vi "ControlProgram5.7.vi"() -> ()   [LabVIEW 2016]
uses:
  <vilib>/Utility/miscctls.llb/LVPoint32TypeDef.ctl
  <vilib>/Platform/TimedLoop/XDataNode/timing_clust.ctl
  <vilib>/Platform/TimedLoop/XDataNode/nitl_modes.ctl
  <vilib>/Platform/TimedLoop/XDataNode/wakeup.ctl
  <vilib>/vision/Avi1.llb/AviRefnum.ctl
  <vilib>/Utility/error.llb/DialogType.ctl
  <vilib>/DAQmx/write.llb/DAQmx Write (Analog 1D DBL NChan 1Samp).vi
  <vilib>/DAQmx/read.llb/DAQmx Read (Analog 2D DBL NChan NSamp).vi
  <vilib>/Analysis/baseanly.llb/Mean (DBL).vi
  <vilib>/DAQmx/write.llb/DAQmx Write (Digital Bool 1Line 1Point).vi
  <vilib>/DAQmx/create/channels.llb/DAQmx Create Channel (DO-Digital Output).vi
  <vilib>/Instr/_visa.llb/VISA Configure Serial Port (Instr).vi
  <vilib>/DAQmx/create/channels.llb/DAQmx Create Channel (AI-Voltage-Basic).vi
  <vilib>/DAQmx/create/channels.llb/DAQmx Create Channel (AO-Voltage-Basic).vi
  <vilib>/DAQmx/configure/timing.llb/DAQmx Timing (Sample Clock).vi
  <vilib>/DAQmx/miscellaneous.llb/DAQmx Fill In Error Info.vi
  <vilib>/Utility/inputDevices.llb/mouseAcquire.vi
  <vilib>/Utility/inputDevices.llb/closeMouse.vi
  <vilib>/platform/TimedLoop/XDataNode/XDataNode.xnode
  <vilib>/Platform/TimedLoop/XDataNode/XDNodeRunTimeDep.lvlib
  <resource>/objmgr/daqmx.rc
  <vilib>/Analysis/NI_AALBase.lvlib
panel:
  out "Primary Video Display":T1(plugin-control)
  in  "Save file index":i32
  out "Flush Sample Start Time":u32=2111292881
  out "Sample flush time (s)":dbl=48.0
  in  "Inject Sample":bool
  out "Chart Freq (Hz)":dbl=500.0
  out "Cal values":T2={"AX alpha"=612.9626061060078, "BX alpha"=549.6584469744151, "AX kappa"=0.3485731373010688, "BX kappa"=0.3853424216291352, "AX offset"=-0.03900484438240665, "BX offset"=-0.11295550662085417, "AY alpha"=582.7562541114835, "BY alpha"=571.1587543790358, "AY kappa"=0.37498408087930674, "BY kappa"=0.36252029651198364, "AY offset"=-0.21125584642206058, "BY offset"=-0.12469077200400738}
  in  "Inject Pump 1":bool
  in  "Inject Pump 2":bool
  in  "Tab Control 2":T3(tab)
  in  "Force FB script":bool
  in  "Got ADig bead":bool
  in  "Move Cap. 2 (ADig Top)":bool
  in  "Dump beads":bool
  in  "Got DNA bead":bool
  in  "Flow on\ncap 2?":bool=TRUE
  in  "Flow on\ncap 1?":bool=TRUE
  in  "Flow on\ndump?":bool=TRUE
  in  "Fish After TA?":bool=TRUE
  in  "Delta after tether":dbl=1700.0
  in  "TA Cancel Save?":bool=TRUE
  in  "Min fish\ndelta (nm)":dbl=1425.0 min=0.0 max=5000.0 step=50.0
  in  "Max fish\ndelta (nm)":dbl=1900.0 min=0.0 max=5000.0 step=25.0
  in  "Fish Speed (ms)":i32=5000
  in  "Wait (ms)":i32=1500
  in  "# attempts":dbl=10.0
  in  "Cutoff force (pN)":dbl=4.5
  in  "Raster after\n tether?":bool=TRUE
  out "Tether":bool
  out "Attempt #":i32
  in  "Flow on\nwhile fish?":bool=TRUE
  in  "Flow on\nafter raster?":bool=TRUE
  in  "Offset @ Delta (nm)":dbl=1700.0
  in  "Cal @ Delta (nm)":dbl=2500.0
  in  "Cal stage position":i32=3
  out "Cal Final Sampling Rate":dbl=125000.0
  in  "Cal Averaging":i32=1
  in  "Wait before dip (s)":dbl=3.0
  in  "Start dipping after?":bool
  in  "Start trap delta (nm)":dbl=1700.0
  in  "Cancel dwell":bool
  in  "Pause dwell":bool
  in  "Return position":dbl=3.0
  in  "Dip duration":dbl=15.0
  in  "Dip position":dbl=4.0
  in  "Dip":bool
  out "Dip time":i32
  in  "Stop":bool=TRUE
  in  "?":T4(tab)
  in  "Cal time (s)":dbl=5.0
  in  "Save N sets":bool
  in  "N sets":i32=200
  out "Cal sets to save":i32=500
  in  "Reset data stream":bool
  out "Buffer Overflow":bool
  out "Stage moving":bool
  in  "Comment":string
  in  "Raster scan":bool
  out "Saving":bool
  in  "Save cal":bool
  in  "Save Data":bool
  in  "Stop saving":bool
  out "Calibrating":bool
  out "Progress":dbl(slide) scale=0.0..100.0
  in  "Read Cal":bool
  in  "Fish":bool
  in  "Averaging Number":i32=1250
  out "Final Sampling Rate":dbl=100.0
  in  "Trap position (V)":cluster{"X":dbl, "Y":dbl}={"X"=3.9042624789680316, "Y"=0.2}
  in  "Trap delta (nm)":dbl=2500.0 min=0.0 max=5000.0 step=50.0
  in  "Fixed X":dbl=1.3
  in  "Fixed Y":dbl=1.8
  in  "Shutter 1 (B)":bool
  in  "Shutter 2 (A)":bool
  in  "Pulling direction":bool
  out "Raster scanning...":bool
  out "Current file name":path=path "D:/data/160111/160111_006.dat"
  in  "AX alpha":dbl=612.9626061060078 format="%#_3p"
  in  "BX alpha":dbl=549.6584469744151 format="%#_3g"
  in  "AX kappa":dbl=0.3485731373010688 format="%#_3g"
  in  "BX kappa":dbl=0.3853424216291352 format="%#_3g"
  in  "AX offset":dbl=-0.03900484438240665 format="%#_3g"
  in  "BX offset":dbl=-0.11295550662085417 format="%#_3g"
  in  "AY alpha":dbl=582.7562541114835 format="%#_3g"
  in  "BY alpha":dbl=571.1587543790358 format="%#_3g"
  in  "AY kappa":dbl=0.37498408087930674 format="%#_3g"
  in  "BY kappa":dbl=0.36252029651198364 format="%#_3g"
  in  "AY offset":dbl=-0.21125584642206058 format="%#_3g"
  in  "BY offset":dbl=-0.12469077200400738 format="%#_3g"
  out "Buffer status":u8(slide) scale=0.0..100.0
  in  "Target":bool
  in  "Set Current\nPos to (0,0,0)":bool
  in  "dump spot":string="Dump beads spot"
  in  "up flow spot":string="Upper flow spot"
  in  "low flow spot":string="Lower flow spot"
  in  "up cap":string="Upper capillary (ADig beads)"
  in  "bottom cap":string="Lower capillary (DNA beads)"
  in  "Move to Position 5":bool
  in  "Set Position 5":bool
  in  "Saved stage positions":dbl[][](array[numeric])=[[1.0, 0.0, 0.0, 0.0], [2.0, -0.13716, -3.21132, 0.01436], [3.0, 0.45, -0.73974, 0.005], [4.0, 0.45, -2.1978, 0.005], [5.0, 0.45, -2.63158, -0.02256]]
  in  "Set Position 2":bool
  in  "Move to Position 2":bool
  in  "Set Position 1":bool
  in  "Move to Position 1":bool
  in  "Set Position 4":bool
  in  "Move to Position 4":bool
  in  "Set Position 3":bool
  in  "Move to Position 3":bool
  out "Stage error":errorcluster
  in  "Clear Volume":bool
  out "Sample Flush Meter":u8(slide) scale=0.0..100.0
  out "Flushing Sample":bool
  in  "Flush Sample":bool
  in  "Normal \nRate (ul/hr)  3":dbl=100.0
  in  "Normal \nVolume (ul) 3":dbl=250.0
  in  "Normal \nVolume (ul) 2":dbl
  in  "Normal \nRate (ul/hr)":dbl
  in  "Normal \nVolume (ul)":dbl
  in  "Flush\nRate (ul/min)":dbl
  in  "Flush\nVolume (ul)":dbl
  in  "Flush \nRate (ul/min)  2":dbl
  in  "Flush Pump 2":bool
  in  "Flush\nVolume (ul)  2":dbl
  in  "Flush Pump 1":bool
  in  "Normal \nRate (ul/hr)  2":dbl
  in  "Write Wait":i32=1000
  in  "Flush \nRate (ul/min)  3":dbl=100.0
  in  "Flush\nVolume (ul)  3":dbl=80.0
  out "error out":errorcluster
  in  "Use Mouse to Move Trap?":bool
  in  "Pause Mouse/Mirror Connection":bool
  out "Reference Voltage":cluster{dbl, dbl}={0.0, -0.0}
  out "Saved voltage":cluster{dbl, dbl}={5.766666666666665, 1.45}
  out "Real Coordinates":cluster{"Horizontal":i32, "Vertical":i32}={"Horizontal"=897, "Vertical"=-1271}
  out "CoordinatesMousePressed":T5
  out "Sum error":dbl(knob) scale=-0.03..0.03
  out "Trap sep":waveform(dbl)[](graph)=[{"t0"=timestamp(16.979999999999855 s since 1904-01-01), "dt"=0.002, "Y"=[2501.0314192873643, 2501.00154430026, 2501.0038423761266, 2500.885491465706, 2500.985457768662], "attributes"=variant("NI_ChannelName"=variant(string "T2 X"))}, {"t0"=timestamp(16.979999999999855 s since 1904-01-01), "dt"=0.002, "Y"=[3.686857270925411, 3.6764288887082217, 3.712276452521894, 3.65426857654364, 3.634715359919401], "attributes"=variant("NI_ChannelName"=variant(string "T2 Y"))}]
  in  "Set reading to\nsetpoint":bool
  in  "Offset Y (nm)":dbl format="%0.2f"
  in  "Offset X (nm)":dbl format="%0.2f"
  in  "Remove offsets":bool
  in  "Force Feedback":bool
  out "Feedback Output Voltage 2":cluster{dbl, dbl} {"?" format="%#_4g"; "?" format="%#_4g"}
  in  "Offset":cluster{"Off Y":dbl, "Off X":dbl}={"Off Y"=1.5, "Off X"=0.17}
  in  "Setpoint voltage":cluster{"SP Y":dbl, "SP X":dbl}={"SP Y"=0.6, "SP X"=0.0}
  in  "Feedback const":T6={"Ki_B_Y"=0.5, "Ki_B_X"=0.0, "Kp Y"=1.0, "Kp X"=0.0}
  out "Mean Trap Pos X 2 (nm)":dbl=2500.981551039624 format="%0.2f"
  out "Mean Trp Pos Y 2 (nm)":dbl=3.6729093097237135 format="%0.2f"
  out "T2 X RMS (A)":dbl=0.5025172745235221 format="%0.2f"
  out "T2 Y RMS (A)":dbl=0.2669441786272784 format="%0.2f"
  in  "Scan range (nm)":dbl=425.0
  in  "Scan speed (nm/s)":dbl=100.0 min=0.0 max=100.0
  in  "Step size (nm)":dbl=1.0
  in  "Save scans":bool=TRUE
  in  "# scans":i32=1
  in  "Load param":bool
  in  "Scan Parameters":T7(array[cluster])=[{"Label"="Offset", "Max delta 2"=3.8, "Start delta 2"=2.4, "Speed (ms) 2"=10000, "# scans 2"=1}]
  in  "Trap delta\nafter (nm)":dbl=1750.0
  in  "Stop raster":bool
  out "Scan range (V)":dbl=0.47672462142456534
  out "Scan steps (mirror)":u64=425
  out "Scan increment (V)":dbl=0.0011217049915872126
  out "Time per step (ms)":dbl=10.0
  out "Total raster time (s)":dbl=8.5
  out "N sets to be saved":dbl=850.0
  in  "Zoom Factor":sgl=7.0
  in  "Center Point":cluster{"X":i32, "Y":i32}={"X"=335, "Y"=271}
  in  "Intensity Upper":dbl=88.0
  in  "Intensity Lower":dbl=66.0
  out "Window Size":cluster{"Height":i32, "Width":i32}
  in  "Image Index":dbl=1.0 min=1.0
  in  "Save Image":bool
  in  "Averaging":bool
  in  "Reset Averaging":bool
  in  "Save Video":bool
  in  "New Video File":bool
  in  "Video Index":dbl=1.0 min=1.0 step=1.0
  in  "Video Capture Rate (Hz)":dbl=30.0
  in  "Initial Window Size":cluster{"Width":i32, "Height":i32}={"Width"=884, "Height"=619}
  in  "Initial Window Position":cluster{"X Position":i32, "Y Position":i32}={"X Position"=796, "Y Position"=4}
  out "Window Position":cluster{"X Position":i32, "Y Position":i32}={"X Position"=40, "Y Position"=40}
  out "Path Out":path
  in  "Target coordinates":cluster{"X1":dbl, "Y1":dbl, "X2":dbl, "Y2":dbl}={"X1"=328.0, "Y1"=274.0, "X2"=368.0, "Y2"=314.0}
  in  "# Samples/channel (in)":i32=40000 format="%.2f"
  out "Buffer size\n(Samples/channel)":u32=511
  out "DAQ rate\n(Samples/s)":dbl=125000.0 format="%#_6p"
  out "# Samples/channel":i32=1250
  out "# Samples/channel/s":dbl=100.0
  out "AvailSampPerChan":u32=9
  out "Data update period (s/set)":dbl=0.01 format="%#_6p"
  out "AvailSampPerChan 2":u32=110
  in  "PC samp per channel":i32=1000
  in  "Sampling Rate":dbl=125000.0 format="%0.0p"
  in  "DAQ Rate2":dbl=1000000.0 format="%#_6p"
  out "Data period (s)":dbl=8e-06 format="%#_6p"
  in  "Tether break\nforce (pN)":dbl=1.0
  in  "Path":path=path "E:/Data"
  out "Mirror task":refnum<k21>
  in  "Conv X (nm/V)":dbl=891.5
  in  "Conv Y (nm/V)":dbl=505.7
  in  "Min value Y":dbl format="%.1g"
  in  "Max value Y":dbl=10.0 format="%.1f"
  in  "Min value X":dbl format="%0.1f"
  in  "Max value X":dbl=10.0 format="%.1f"
  in  "HWP1":string="Half waveplate 1: differential trap power"
  in  "HWP0":string="Half waveplate 0: total trap power"
  in  "Move 1":bool
  in  "\"Degrees\" 1":dbl
  in  "Move 0":bool
  in  "\"Degrees\" 0":dbl
  out "Deflection":T5
  in  "Sampling Rate":dbl=125000.0 format="%0.2f"
  in  "Averaging Number":i32=12500
  in  "DAQ Rate":dbl=1000000.0
  out "Final Sampling Rate":dbl
  in  "Tab Control":T8(tab)
  in  "Downsamp\nfact":dbl=250.0
  out "Bead sep":waveform(dbl)[](graph)=[{"t0"=timestamp(16.979999999999855 s since 1904-01-01), "dt"=0.002, "Y"=[1328.897036761212, 1305.1388835394264, 1332.9488147379952, 1348.9983032616292, 1330.6351248700973], "attributes"=variant("NI_ChannelName"=variant(string "T2"))}, {"t0"=timestamp(16.979999999999855 s since 1904-01-01), "dt"=0.002, "Y"=[125.02264592216193, 122.42682026580995, 123.20185663198687, 125.52620860986364, 123.54404369854063], "attributes"=variant("NI_ChannelName"=variant(string "T1"))}]
  out "Force (pN)":waveform(dbl)[](graph)=[{"t0"=timestamp(16.979999999999855 s since 1904-01-01), "dt"=0.002, "Y"=[464.2815568920448, 456.0098292427729, 465.67524311796336, 471.29790632841843, 464.8843576940994], "attributes"=variant("NI_ChannelName"=variant(string "T2"))}, {"t0"=timestamp(16.979999999999855 s since 1904-01-01), "dt"=0.002, "Y"=[45.46636056045166, 44.5015348242116, 44.800567281242486, 45.640259630893546, 44.914644785188166], "attributes"=variant("NI_ChannelName"=variant(string "T1"))}]
  out "Mean force (pN)":dbl=254.74722603572863 format="%0.2f"
  out "Force noise (pN)":dbl=2.6193969378282405 format="%0.2f"
  out "Mean Bead Sep\n(nm)":dbl=726.6339738298723 format="%0.2f"
  out "Bead Sep Noise\n(A)":dbl=74.90033509004418 format="%0.2f"
  out "PSD 2":cluster{dbl[], dbl[]}(graph)
  out "PSD 1":cluster{dbl[], dbl[]}(graph)
  out "PSD 1 Sum":dbl(slide) scale=0.0..10.0
  out "PSD 2 Sum":dbl(slide) scale=0.0..10.0
  in  "Start":bool
  out "All signals":waveform(dbl)[](graph)=[{"t0"=timestamp(16.979999999999855 s since 1904-01-01), "dt"=0.002, "Y"=[0.0016346282006063629, 0.0016395264340522623, 0.0015951845291293394, 0.001643393460571591, 0.001619417895638828], "attributes"=variant("NI_ChannelName"=variant(string "A y"))}, {"t0"=timestamp(16.979999999999855 s since 1904-01-01), "dt"=0.002, "Y"=[0.019187765824921398, 0.019071754997447867, 0.019093410352219186, 0.01908722310790174, 0.01906840357389384], "attributes"=variant("NI_ChannelName"=variant(string "A x"))}, {"t0"=timestamp(16.979999999999855 s since 1904-01-01), "dt"=0.002, "Y"=[-0.0018054787241975109, -0.0017869169958937155, -0.0017822765638718496, -0.001786143590850525, -0.0017809875549530127], "attributes"=variant("NI_ChannelName"=variant(string "B y"))}, {"t0"=timestamp(16.979999999999855 s since 1904-01-01), "dt"=0.002, "Y"=[-0.00033504945472925915, -0.00036108743413889715, -0.0003409788953336346, -0.00033788527392585174, -0.0003489707505394131], "attributes"=variant("NI_ChannelName"=variant(string "B x"))}, {"t0"=timestamp(16.979999999999855 s since 1904-01-01), "dt"=0.002, "Y"=[0.009149844795781155, 0.009267130525609176, 0.00907380239980559, 0.008962960940972408, 0.00908024667059773], "attributes"=variant("NI_ChannelName"=variant(string "A sum"))}, {"t0"=timestamp(16.979999999999855 s since 1904-01-01), "dt"=0.002, "Y"=[0.005338703023696027, 0.005341280732029953, 0.005316792503079397, 0.005262660628286258, 0.005297459690626533], "attributes"=variant("NI_ChannelName"=variant(string "B sum"))}, {"t0"=timestamp(16.979999999999855 s since 1904-01-01), "dt"=0.002, "Y"=[3.905419427131087, 3.9053859162089286, 3.9053884939720995, 3.9052557391651215, 3.905367871866138], "attributes"=variant("NI_ChannelName"=variant(string "Trap x"))}, {"t0"=timestamp(16.979999999999855 s since 1904-01-01), "dt"=0.002, "Y"=[0.2072906016826684, 0.2072699800053554, 0.20734086702100435, 0.2072261589411581, 0.20718749329626143], "attributes"=variant("NI_ChannelName"=variant(string "Trap y"))}]
  # "Bead Calibration"
  # "Y"
  # "X"
  # "Pump #1 Controls"
  # "Pump #2 Controls"
  # "Sample Pump Controls"
  # "Retract the pumps manually. Change it back to INFUSE when you're done. Suck it up, don't whine."
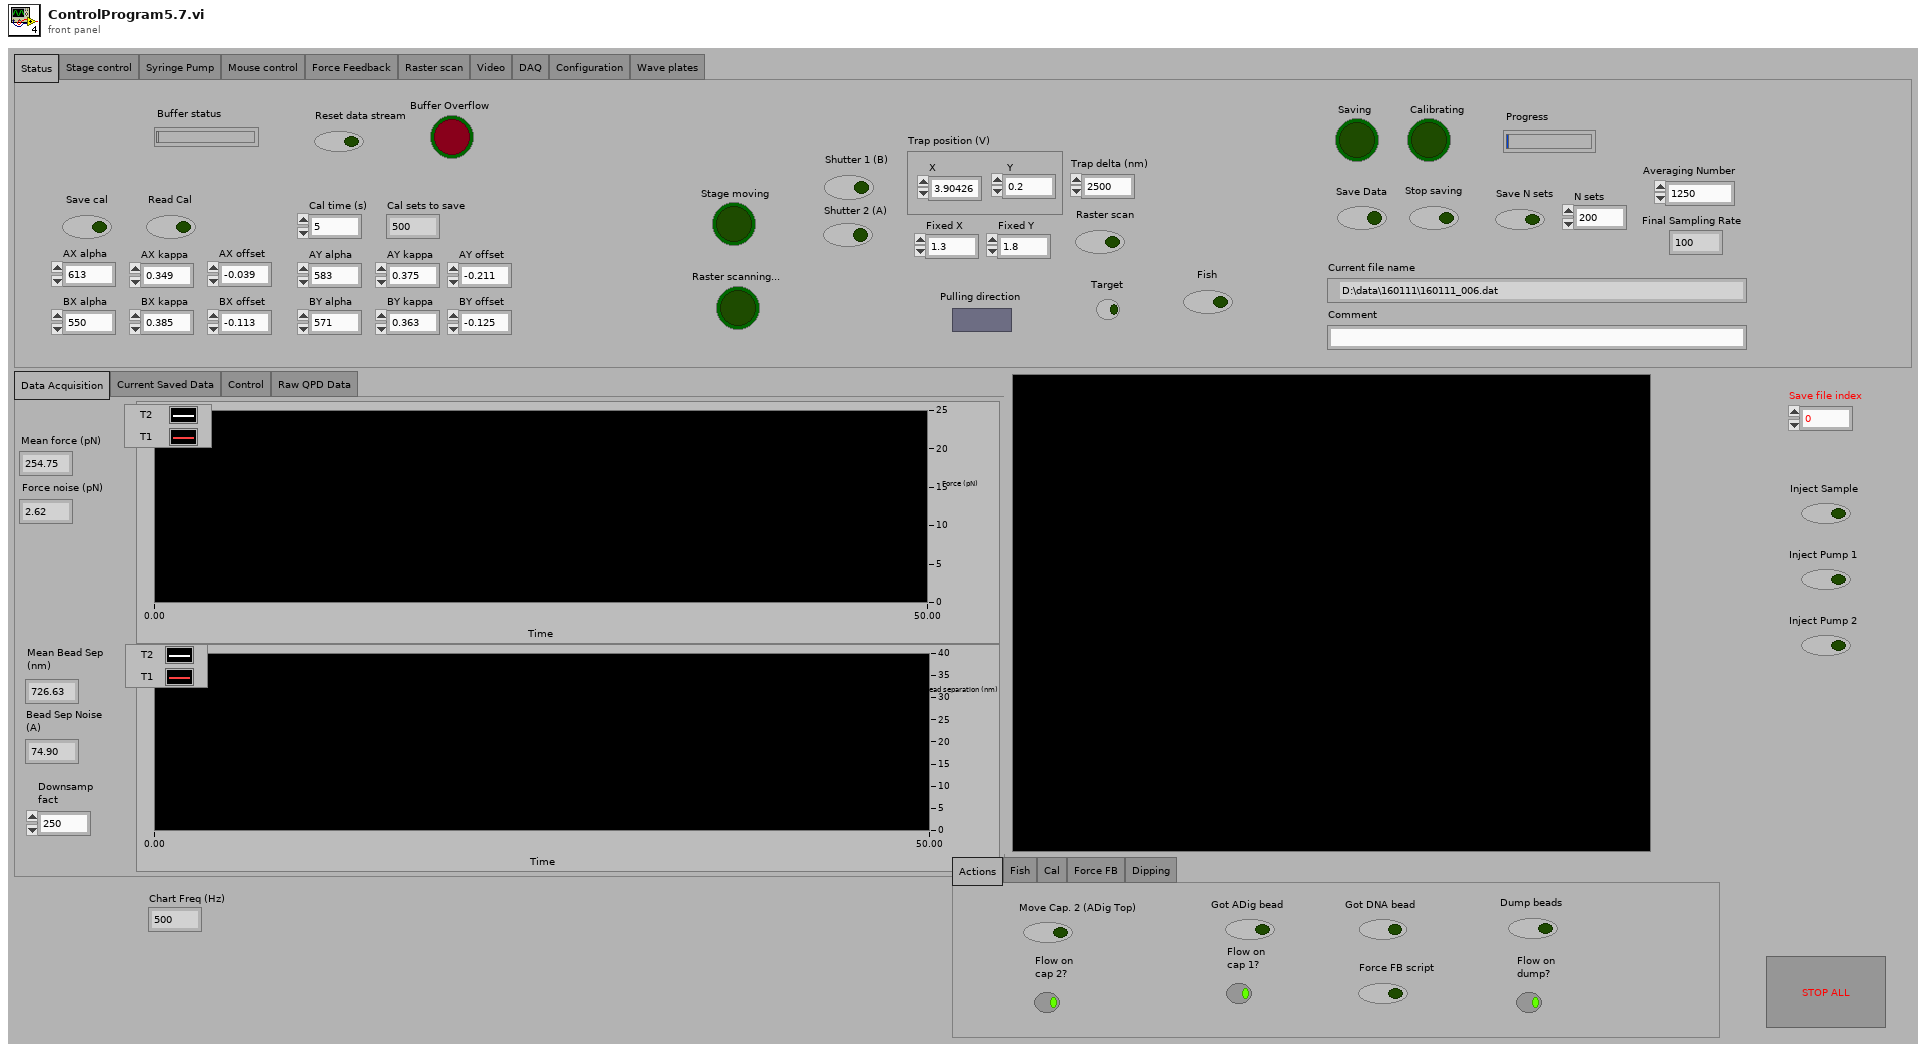
[diagram p1: front panel]
types:
  T1 = typedef "IMAQ Image.ctl" = refnum<image>
  T2 = cluster{"AX alpha":dbl, "BX alpha":dbl, "AX kappa":dbl, "BX kappa":dbl, "AX offset":dbl, "BX offset":dbl, "AY alpha":dbl, "BY alpha":dbl, "AY kappa":dbl, "BY kappa":dbl, "AY offset":dbl, "BY offset":dbl}
  T3 = enum32{"Actions", "Fish", "Cal", "Force FB", "Dipping"}
  T4 = enum32{"Status", "Stage control", "Syringe Pump", "Mouse control", "Force Feedback", "Raster scan", "Video", "DAQ", "Configuration", "Wave plates"}
  T5 = typedef "LVPoint32TypeDef.ctl" = cluster{"Horizontal":i32, "Vertical":i32}
  T6 = cluster{"Ki_B_Y":dbl, "Ki_B_X":dbl, "Kp Y":dbl, "Kp X":dbl}
  T7 = cluster{"Label":string, "Max delta 2":dbl, "Start delta 2":dbl, "Speed (ms) 2":i32, "# scans 2":i32}[]
  T8 = enum32{"Data Acquisition", "Current Saved Data", "Control", "Raw QPD Data"}
  T9 = enum32{"setting", "request", "request control", "info", "statistics", "system settings", "I/O sub system", "HRT control", "camera descriptions", "device specific data", "event sub system settings", "event sub system results", "image memory manager"}
  T10 = typedef "AviRefnum.ctl" = refnum<k1>
  T11 = typedef "XDNodeRunTimeDep.lvlib/timing_clust.ctl" = cluster{"Expected End [f-1]":u64, "Actual End [f-1]":u64, "Finished Late? [f-1]":bool, "Expected End [i-1]":u64, "Actual End [i-1]":u64, "Finished Late? [i-1]":bool, "Expected Start [i]":u64, "Actual Start [i]":u64, "Expected Start [f]":u64, "Actual Start [f]":u64, "Source Name":string, "Structure Name":string, "Period":i64, "Deadline":i64, "Offset":i64, "Start":i64, "Priority":i32, "Timeout":i32, "Mode":T12, "Wakeup Reason":T13, "Error":errorcluster, "Source Type":string, "Secondary Source Type":string, "Global End Time":u64, "Global Start Time":u64, "Frame Duration":u64, "Iteration Duration":u64, "Assigned CPU":i32, "I/O Scan Engine Mode":u32}
  T12 = typedef "XDNodeRunTimeDep.lvlib/nitl_modes.ctl" = enum32{"No Change", "Process missed periods, maintain original phase", "Discard missed periods, maintain original phase", "Process missed periods, ignore original phase", "Discard missed periods, ignore original phase"}
  T13 = typedef "XDNodeRunTimeDep.lvlib/wakeup.ctl" = enum32{"Normal", "Aborted", "Asynchronous wakeup", "Timing source error", "Timed loop error", "Timeout"}
  T14 = typedef "Image Type" = u32
  T15 = typedef "imagedata.ctl" = cluster{"image type":i32, "image depth":i32, "image":u8[], "mask":u8[], "colors":u32[], "Rectangle":cluster{"left":i16, "top":i16, "right":i16, "bottom":i16}}
  T16 = enum16{"open", "replace", "create", "open or create", "replace or create", "replace or create with confirmation"}
  T17 = enum16{"big-endian, network order", "native, host order", "little-endian"}
  T18 = cluster{string, string, string, string, string, string, string, string}
  T19 = typedef "DialogType.ctl" = u16
  T20 = cluster{"button 1":bool, "button 2":bool, "button 3":bool, "button 4":bool}
  T21 = cluster{"[0]":dbl, "[1]":dbl, "[2]":dbl, "[3]":dbl, "[4]":dbl, "[5]":dbl, "[6]":dbl, "[7]":dbl, "[8]":dbl, "[9]":dbl, "[10]":dbl, "[11]":dbl}
  T22 = cluster{"Label":string, "Max delta 2":dbl, "Start delta 2":dbl, "Speed (ms) 2":i32, "# scans 2":i32}
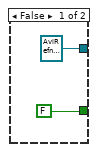
[diagram p2: hidden frame]
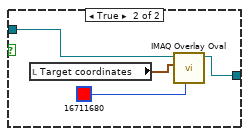
[diagram p5: hidden frame]
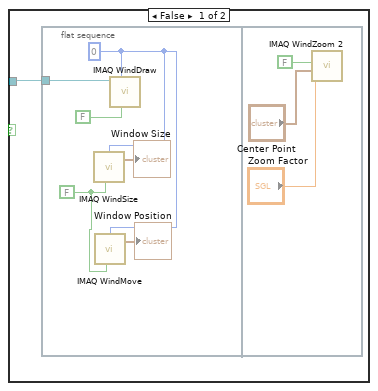
[diagram p6: hidden frame]
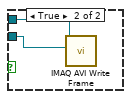
[diagram p8: hidden frame]
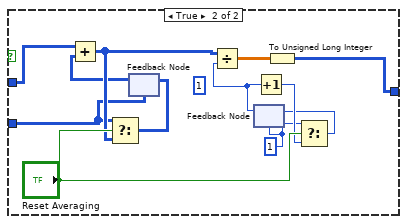
[diagram p9: hidden frame]
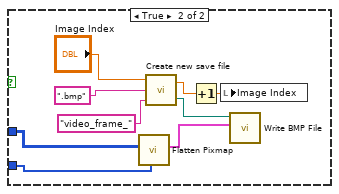
[diagram p10: hidden frame]
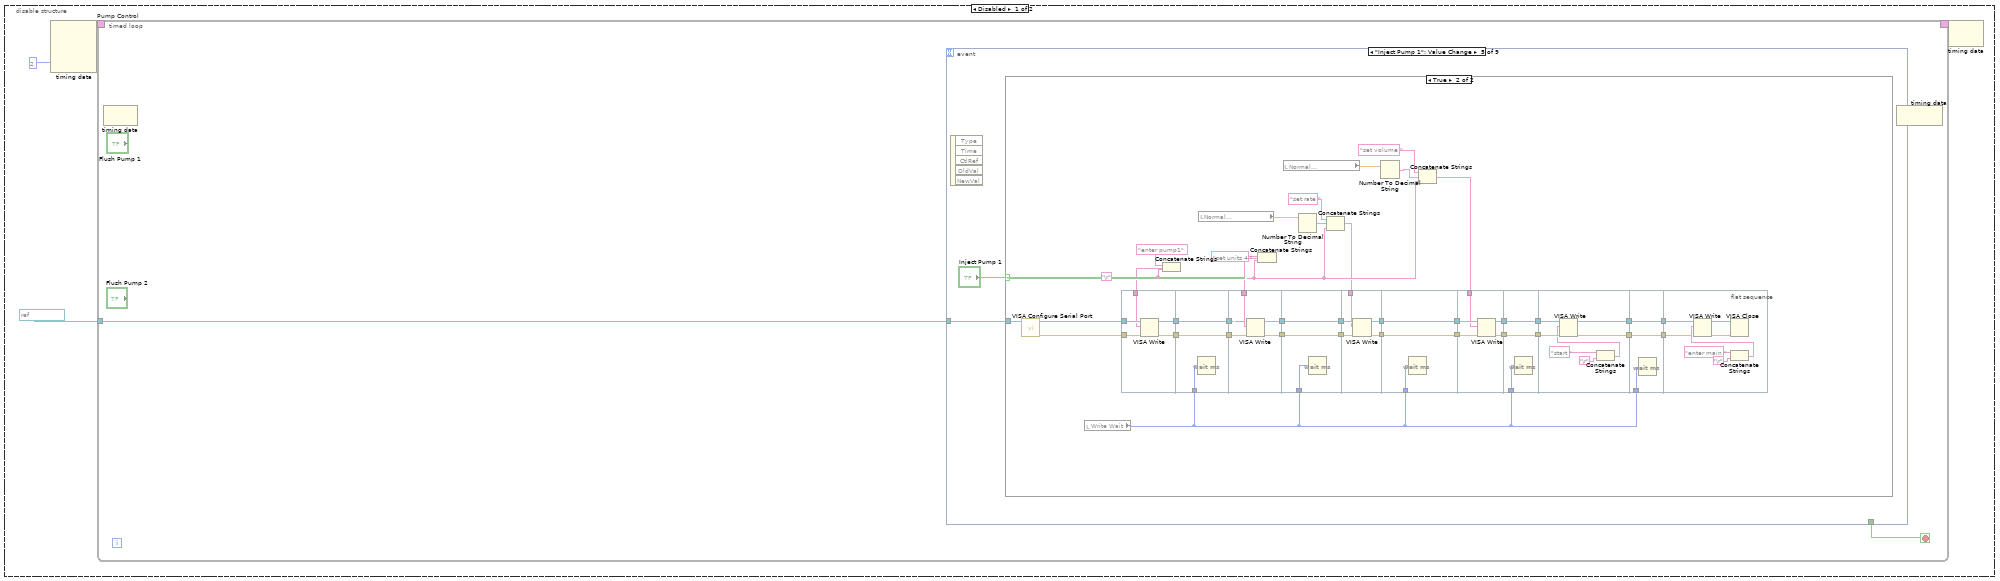
[diagram p11: hidden frame]
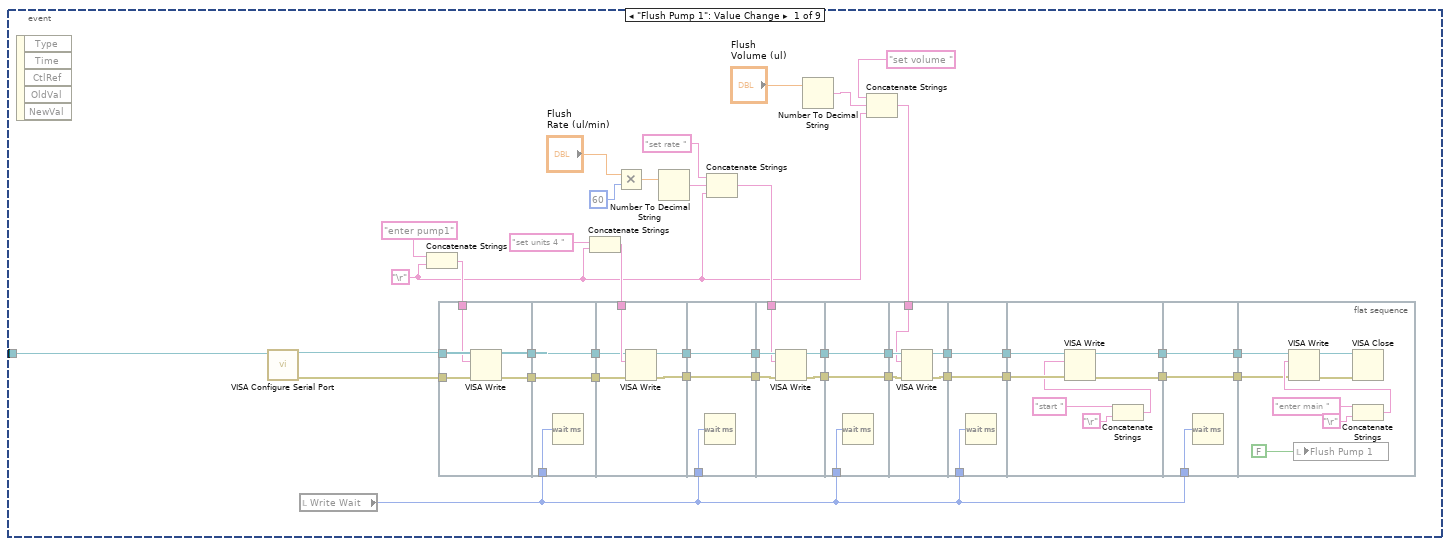
[diagram p12: hidden frame]
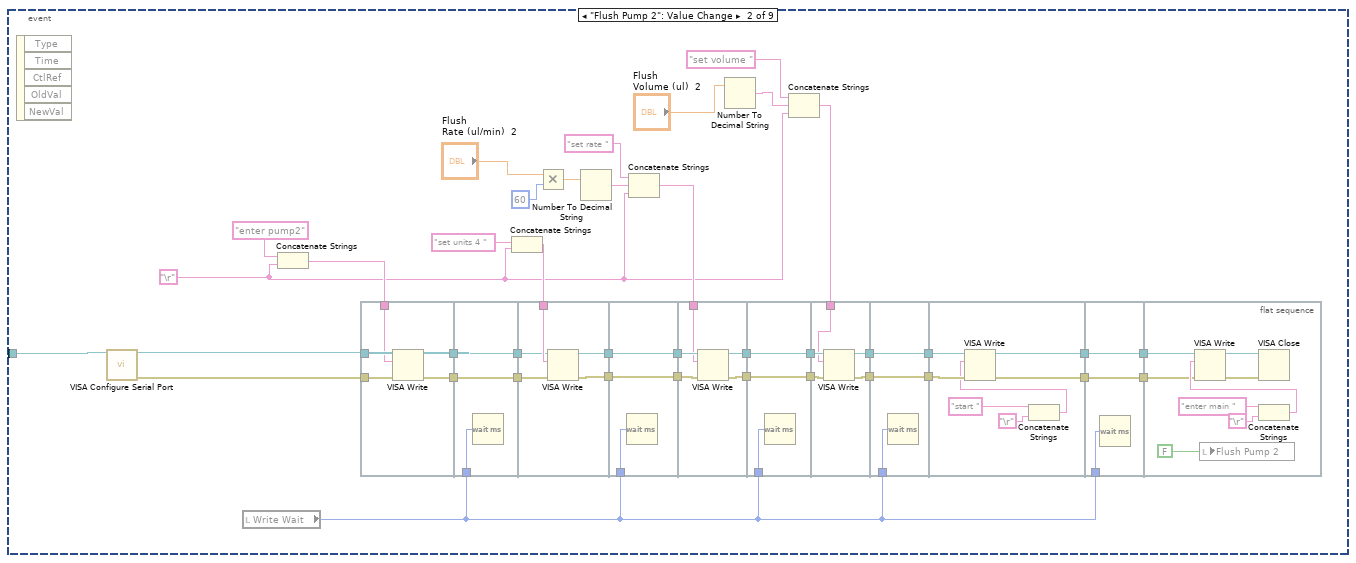
[diagram p13: hidden frame]
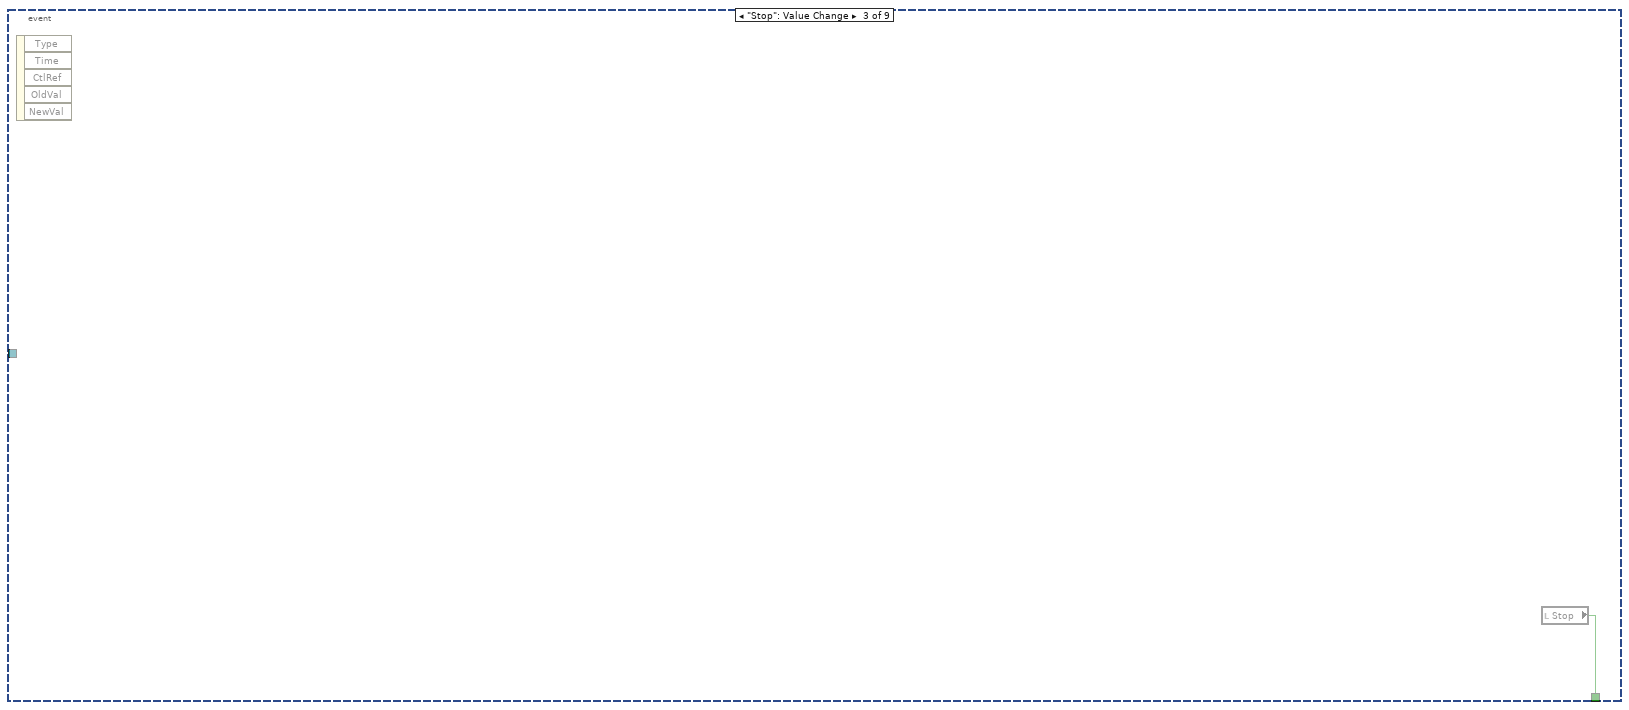
[diagram p14: hidden frame]
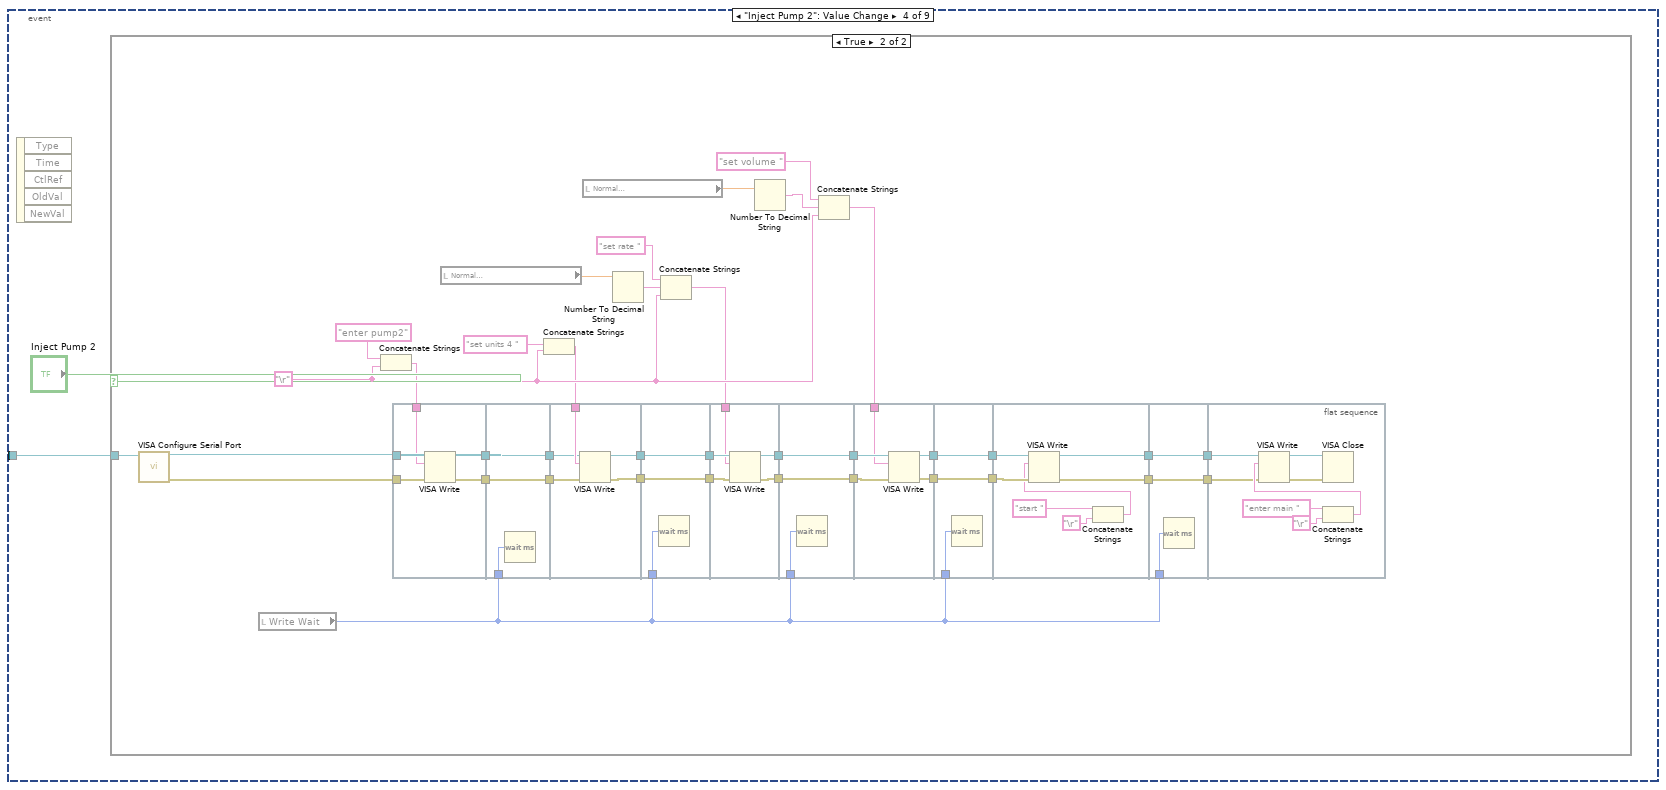
[diagram p15: hidden frame]
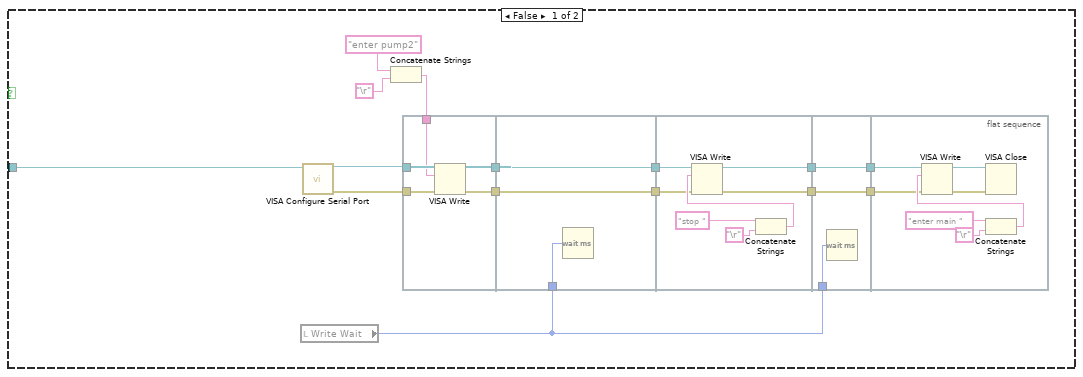
[diagram p16: hidden frame]
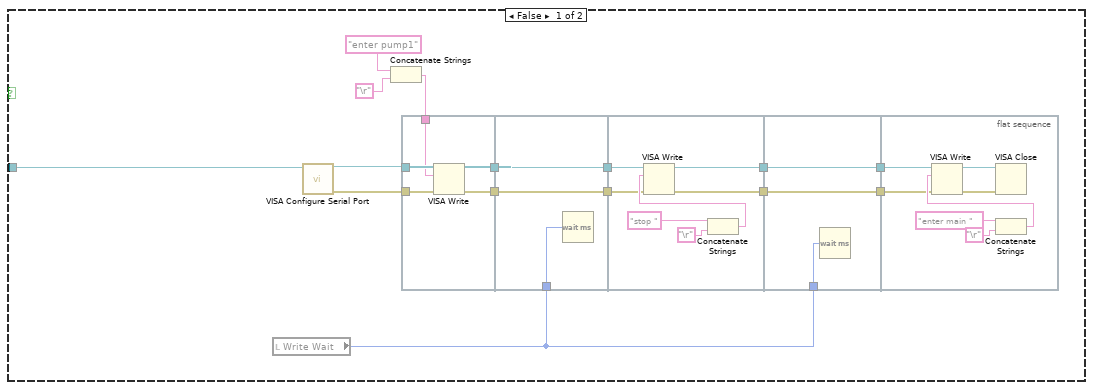
[diagram p17: hidden frame]
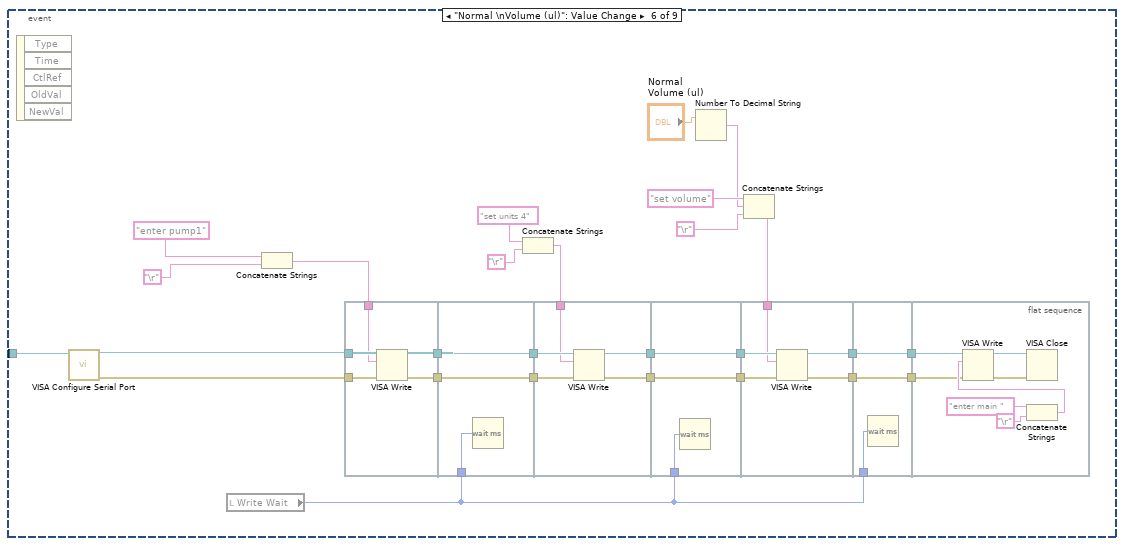
[diagram p18: hidden frame]
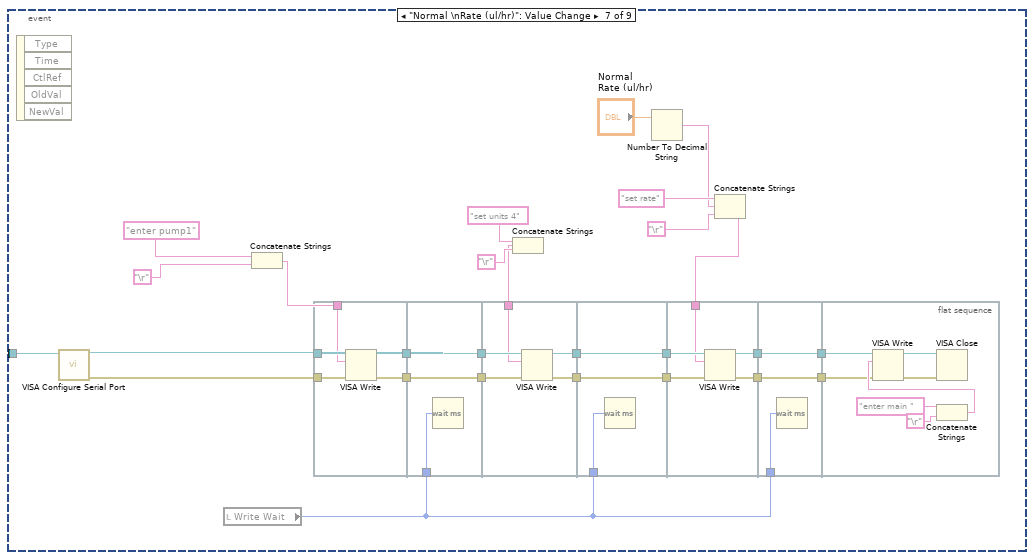
[diagram p19: hidden frame]
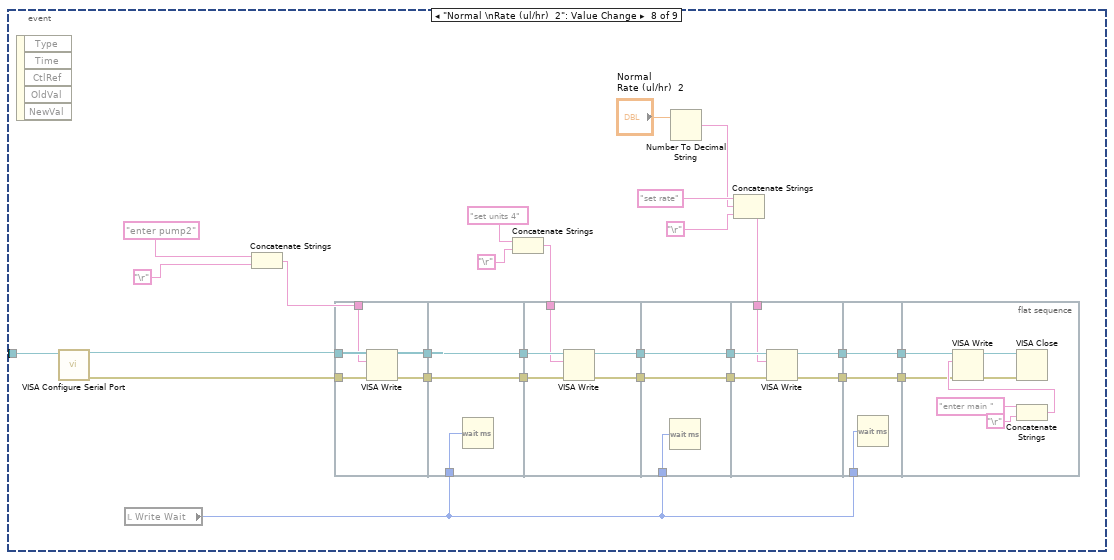
[diagram p20: hidden frame]
diagram:
  w38 = 10.0 ("Minimum Value")
  w39 = -10.0 ("Minimum Value")
  w41 = -2.0 ("Minimum Value")
  w42 = 2.0 ("Maximum Value")
  w67 = 10123 items=["Finite Samples"=10178, "Continuous Samples"=10123] ("sample mode")
  w88 = tag "Dev1/port2/line1"  # Shutter 2
  w91 = tag "Dev1/port1/line4"  # Shutter 1
  # "Create channels for movable mirror"
  # "Create channels for detectors"
  n1 = call-poly <vilib>:"DAQmx Create Virtual Channel.vi"("maximum value"=w42, "minimum value"=w41, "physical channels"=tag "Dev1/ai0" ("Physical Channel")) -> ("task out"=w43:refnum<k21>, "error out"=w66:errorcluster)  [unwired: 11 in]
  n2 = call-poly <vilib>:"DAQmx Create Virtual Channel.vi"("task in"=w43, "maximum value"=w42, "minimum value"=w41, "physical channels"=tag "Dev1/ai1", "error in"=w66) -> ("task out"=w64:refnum<k21>, "error out"=w63:errorcluster)  [unwired: 9 in]
  n3 = call-poly <vilib>:"DAQmx Create Virtual Channel.vi"("task in"=w64, "maximum value"=w42, "minimum value"=w41, "physical channels"=tag "Dev1/ai2", "error in"=w63) -> ("task out"=w55:refnum<k21>, "error out"=w54:errorcluster)  [unwired: 9 in]
  n4 = call-poly <vilib>:"DAQmx Create Virtual Channel.vi"("task in"=w55, "maximum value"=w42, "minimum value"=w41, "physical channels"=tag "Dev1/ai3" ("Physical Channel"), "error in"=w54) -> ("task out"=w40:refnum<k21>, "error out"=w60:errorcluster)  [unwired: 9 in]
  n5 = call-poly <vilib>:"DAQmx Create Virtual Channel.vi"("task in"=w40, "maximum value"=w38, "minimum value"=w39, "physical channels"=tag "Dev1/ai4", "error in"=w60) -> ("task out"=w58:refnum<k21>, "error out"=w57:errorcluster)  [unwired: 9 in]
  n6 = call-poly <vilib>:"DAQmx Create Virtual Channel.vi"("task in"=w58, "maximum value"=w38, "minimum value"=w39, "physical channels"=tag "Dev1/ai5", "error in"=w57) -> ("task out"=w53:refnum<k21>, "error out"=w52:errorcluster)  [unwired: 9 in]
  n7 = call-poly <vilib>:"DAQmx Create Virtual Channel.vi"("task in"=w53, "maximum value"=w38, "minimum value"=w39, "physical channels"=tag "Dev1/ai6", "error in"=w52) -> ("task out"=w47:refnum<k21>, "error out"=w45:errorcluster)  [unwired: 9 in]
  n8 = call-poly <vilib>:"DAQmx Create Virtual Channel.vi"("task in"=w47, "maximum value"=w38, "minimum value"=w39, "physical channels"=tag "Dev1/ai7", "error in"=w45) -> ("task out"=w46:refnum<k21>, "error out"=w44:errorcluster)  [unwired: 9 in]
  n9 = call-poly <vilib>:"DAQmx Timing.vi"("task/channels in"=w46, "sample mode"=w67, "samples per channel"="PC samp per channel", "rate"="Sampling Rate", "error in"=w44) -> ("task out"=w50:refnum<k21>, "error out"=w49:errorcluster)  [unwired: 9 in]
  n10 = call-poly <vilib>:"DAQmx Create Virtual Channel.vi"("maximum value"="Max value Y", "minimum value"="Min value Y", "physical channels"=tag "Dev1/ao1" ("Trap X Axis")) -> ("task out"=w35:refnum<k21>, "error out"=w37:errorcluster)  [unwired: 11 in]
  n11 = property class="DAQmx Timing"(reference=w50, error in=w49, "More:AI Convert:Rate"="DAQ Rate2") -> (reference out=w7:refnum<k21>, error out=w6:errorcluster, "SampClk.Rate"=→"DAQ rate\n(Samples/s)":dbl)
  n12 = call-poly <vilib>:"DAQmx Create Virtual Channel.vi"("task in"=w35, "maximum value"="Max value X", "minimum value"="Min value X", "physical channels"=tag "Dev1/ao0" ("Trap Y Axis"), "error in"=w37) -> ("task out"=w26:refnum<k21>, "error out"=w25:errorcluster)  [unwired: 9 in]
  "Mirror task" <- w26
  n13 = property class="DAQmx Buffer"(reference=w7, error in=w6) -> (reference out=w4:refnum<k21>, error out=w3:errorcluster, "Input.OnbrdBufSize"=→"Buffer size\n(Samples/channel)":u32)
  n14 = call <vilib>:"DAQmx Start Task.vi"("task/channels in"=w4, "error in"=w3) -> ("task out"=w27:refnum<k21>)  [unwired: 12 in, 1 out]
  n15 = flat-sequence "Video" {
    tunnel: [w104] -> w1
    tunnel: w1 -> [w145]
    frame #0 {
      n16 = while {
        stop <- w97 continue-if-true
        n17 = call "Close Video Capture.vi"() -> ("error code OUT"=w99:i32)
        n18 = Equal?(x=w99, y=0) -> (x = y?=w97:bool)
      }
      n19 = local write "Stop"(FALSE ("Stop All")) -> ()
    }
    frame #1 {
      n20 = call "DMR_Init.vi"() -> ()  [unwired: 3 out]
    }
    frame #2 {
      # "Setting the destination format to Mono8 makes sure that the image can be displayed in the intensity plot."
      n21 = call "DMR_GetDevice.vi"("search string IN"="DE514724602") -> ("device handle OUT"=w122:i32)  [unwired: 4 in, 2 out]
      n22 = call "DMR_OpenDevice.vi"("device handle IN"=w122) -> ("driver handle OUT"=w105:i32)  [unwired: 4 out]
      n23 = call "DMR_FindList.vi"("flags IN"=u32 0 ("flags"), "list name IN"="" ("String"), "list type IN"=T9."camera descriptions", "driver handle IN"=w105) -> ("list handle OUT"=w108:i32)  [unwired: 2 out]
      n24 = call "DMR_FindList.vi"("flags IN"=u32 0 ("flags"), "list name IN"="Base", "list type IN"=T9."setting", "driver handle IN"=w105) -> ("list handle OUT"=w106:i32)  [unwired: 2 out]
      n25 = call "OBJ_GetHandle.vi"("object name IN"="VideoStandard", "list handle IN"=w108) -> ("object handle OUT"=w102:i32)  [unwired: 3 out]
      n26 = call "OBJ_GetHandle.vi"("object name IN"="PixelFormat", "list handle IN"=w106) -> ("object handle OUT"=w116:i32)  [unwired: 3 out]
      n27 = call "OBJ_SetS.vi"("value index IN"=0, "value IN"="NTSC M", "object handle IN"=w102) -> ()  [unwired: 2 out]
      n28 = call "OBJ_SetS.vi"("value index IN"=0, "value IN"="Mono8" ("value"), "object handle IN"=w116) -> ()  [unwired: 2 out]
      n29 = call "OBJ_GetHandle.vi"("object name IN"="VideoChannel", "list handle IN"=w106) -> ("object handle OUT"=w112:i32)  [unwired: 3 out]
      n30 = while {
        tunnel: [w127] -> w104
        tunnel: w105 -> [w124]
        stop <- w125 continue-if-true
        n31 = call "DMR_ImageRequestSingle.vi"("request control IN"=0, "driver handle IN"=w124) -> ("error code OUT"=w126:i32, "driver handle OUT"=w127:i32)  [unwired: 2 out]
        n32 = Equal To 0?(x=w126) -> (x = 0?=w125:bool)
      }
      n33 = call "OBJ_SetI.vi"("value index IN"=0, "value IN"=0 ("Video channel"), "object handle IN"=w112) -> ()  [unwired: 2 out]
    }
    frame #3 {
      w133 = T14 0 items=["Grayscale (U8)", "Grayscale (I16)", "Grayscale (SGL)", "Complex (CSG)", "RGB (U32)", "HSL (U32)", "RGB (U64)"] ("Image Type")
      w141 = T14 0 items=["Grayscale (U8)", "Grayscale (I16)", "Grayscale (SGL)", "Complex (CSG)", "RGB (U32)", "HSL (U32)", "RGB (U64)"] ("Image Type")
      n34 = for "Create Greyscale map" {
        N: 256 -> [_]
        tunnel: [w147] -> w130 mode=indexing
        workers-P: _ -> [_]
        i -> [w150]
        n35 = To Unsigned Byte Integer(number=w150) -> (unsigned 8bit integer=w146:u8)
        n36 = Join Numbers(hi=w146, lo=w146) -> ((hi.lo)=w149:u16)
        n37 = Join Numbers(hi=w146, lo=w146) -> ((hi.lo)=w148:u16)
        n38 = Join Numbers(hi=w149, lo=w148) -> ((hi.lo)=w147:u32)
      }
      n39 = call "IMAQ Create"("Image Name"="Scaled video", "Image Type"=w133) -> ("New Image"=w132:T1)  [unwired: 2 in, 2 out]
      n40 = call "IMAQ Create"("Image Name"="Main video", "Image Type"=w141) -> ("New Image"=w142:T1)  [unwired: 2 in, 2 out]
      n41 = node-c288(0 ("Processor")) -> (w140:T11)  [unwired: 3 out]
      n42 = Initialize Array(u32 0 ("Window Number (0...15)"), 480 ("dimension size"), 640 ("dimension size")) -> (w135:u32[][])
      n43 = timed-loop {
        tunnel: w145 -> [w167]
        tunnel: [w166] -> w144
        tunnel: w142 -> [w165]
        timing: w140 -> [_]
        timing-out: [_] -> w139
        tunnel: w135 -> [w154]
        tunnel: w132 -> [w152]
        tunnel: w130 -> [w151]
        stop <- w153 stop-if-true
        # "This block performs the \nactual image capture."
        n44 = node-c288() -> ()  [unwired: 2 out]
        n45 = local read "Stop"() -> (w153:bool)
        n46 = Reciprocal(x="Video Capture Rate (Hz)") -> (1/x=w157:dbl)
        n47 = Multiply(x=w157, y=1000.0) -> (x*y=w155:dbl)
        n48 = call "DMR_ImageRequestWaitFor.vi"("queue number IN"=0, "timeout(ms) IN"=500, "driver handle IN"=w167) -> ("error code OUT"=w171:i32, "request number OUT"=w168:i32, "driver handle OUT"=w169:i32)
        n49 = feedback #1(T10 refnum ("Avi Refnum")) -> (w159:T10)
        n50 = case shown="True" "New Video File" {
          tunnel: [T10 refnum ("Avi Refnum") w188] -> w161
          tunnel: [FALSE TRUE] -> w162
          tunnel: w159 -> [_ w184]
          frame False {
          }
          frame True {
            n51 = call "Create new save file.vi"("Ext"=".avi" ("string"), "Index In"="Video Index") -> ("Path Out"=w180:path, "Index Out"=w181:dbl)  [unwired: 1 in]
            "Path Out" <- w180
            n52 = Not Equal?(x=w184, y=T10 refnum ("Avi Refnum")) -> (x != y?=w185:bool)
            n53 = Increment(x=w181) -> (x+1=w190:dbl)
            n54 = case shown="True" w185 {
              tunnel: w184 -> [_ w191]
              frame False {
              }
              frame True {
                n55 = call "IMAQ AVI Close"("Avi Refnum"=w191) -> ()  [unwired: 1 in, 10 out]
              }
            }
            n56 = local write "Video Index"(w190) -> ()
            n57 = call "IMAQ AVI Create"("Frames Per Second"=u32 30, "AVI Path"=w180) -> ("Avi Refnum"=w188:T10)  [unwired: 5 in, 4 out]
          }
        }
        n58 = Equal To 0?(x=w171) -> (x = 0?=w170:bool)
        n59 = Select(t=w161, s=w162, f=w159) -> (s? t:f=w160:T10)
        n60 = feedback-in #1(w160) -> ()
        n61 = case shown="True" w170 {
          tunnel: w169 -> [w192 w219]
          tunnel: w168 -> [_ w218]
          tunnel: [w192 w215] -> w166
          tunnel: w165 -> [_ w196]
          tunnel: w154 -> [_ w203]
          tunnel: w160 -> [_ w201]
          tunnel: w152 -> [_ w197]
          tunnel: w151 -> [_ w198]
          frame False {
          }
          frame True {
            w209 = u32 0 ("X-offset IN")
            n62 = call "DMR_GetImageRequestBufferData.vi"("driver handle IN"=w219, "request number IN"=w218) -> ("width OUT"=w208:i32, "height OUT"=w207:i32, "driver handle OUT"=w214:i32, "request number OUT"=w213:i32, "bytes per pixel OUT"=w210:i32)  [unwired: 13 out]
            n63 = call "DMR_GetImageRequestBufferImageData.vi"("driver handle IN"=w214, "request number IN"=w213, "bytes per pixel IN"=w210, "X-offset IN"=w209, "Y-offset IN"=w209, "height IN"=w207, "width IN"=w208) -> ("driver handle OUT"=w212:u32, "request number OUT"=w211:u32, "image OUT"=w204:u32[][])  [unwired: 10 out]
            n64 = call "DMR_ImageRequestUnlock.vi"("request number IN"=w211, "driver handle IN"=w212) -> ("driver handle OUT"=w217:i32)  [unwired: 1 in, 2 out]
            n65 = case shown="False" "Averaging" {
              tunnel: w204 -> [w260 w265]
              tunnel: [w260 w264] -> w200
              tunnel: w203 -> [_ w262]
              frame False {
              }
              frame True {
                (unwired) 1
                w270 = 1
                n66 = feedback #2(w262) -> (w261:u32[][])
                n67 = Add(x=w265, y=w261) -> (x+y=w266:u32[][])
                n68 = Select(t=w262, s="Reset Averaging", f=w266) -> (s? t:f=w268:u32[][])
                n69 = feedback-in #2(w268) -> ()
                n70 = feedback #3(w270) -> (w263:i32)
                n71 = Divide(x=w266, y=w263) -> (x/y=w267:dbl[][])
                n72 = Increment(x=w263) -> (x+1=w271:i32)
                n73 = To Unsigned Long Integer(number=w267) -> (unsigned 32bit integer=w264:u32[][])
                n74 = Select(t=w270, s="Reset Averaging", f=w271) -> (s? t:f=w269:i32)
                n75 = feedback-in #3(w269) -> ()
              }
            }
            n76 = call "DMR_ImageRequestSingle.vi"("request control IN"=0, "driver handle IN"=w217) -> ("driver handle OUT"=w215:i32)  [unwired: 3 out]
            n77 = disable-structure shown="Disabled" {
              disable-tunnel: w200 -> [w237 _]
              disable-tunnel: w197 -> [w236 _]
              frame Disabled {
                n78 = To Double Precision Float(number=w237) -> (double precision float=w235:dbl[][])
                n79 = In Range and Coerce(upper limit="Intensity Upper", x=w235, lower limit="Intensity Lower") -> (coerced(x)=w234:dbl[][])  [unwired: 1 out]
                n80 = Subtract(x="Intensity Upper", y="Intensity Lower") -> (x-y=w231:dbl)
                n81 = Subtract(x=w234, y="Intensity Lower") -> (x-y=w232:dbl[][])
                n82 = Divide(x=w232, y=w231) -> (x/y=w233:dbl[][])
                n83 = Multiply(x=255.0, y=w233) -> (x*y=w229:dbl[][])
                n84 = To Unsigned Byte Integer(number=w229) -> (unsigned 8bit integer=w238:u8[][])
                n85 = call "IMAQ ArrayToImage"("Image Pixels (U8)"=w238, "Image"=w236) -> ("Image Out"=w225:T1)  [unwired: 4 in, 5 out]
                n86 = First Call?() -> (First Call?: T/F=w226:bool)
                n87 = case shown="True" w226 {
                  tunnel: w225 -> [w239 w250]
                  frame False {
                    n88 = flat-sequence {
                      tunnel: w239 -> [w245]
                      frame #0 {
                        w242 = FALSE ("Get/Set Status? (Set)")
                        w241 = 0 ("Window Number (0...15)")
                        n89 = call "IMAQ WindSize"("Get/Set Status? (Set)"=w242, "Window Number"=w241) -> ("Width & Height out"=→"Window Size":cluster{"Width":i32, "Height":i32})  [unwired: 4 in, 2 out]
                        n90 = call "IMAQ WindMove"("Window Number (0...15)"=w241, "Get/Set Status? (Set)"=w242) -> ("Coordinates (screen)"=→"Window Position":cluster{"X Position":i32, "Y Position":i32})  [unwired: 3 in, 1 out]
                        n91 = call "IMAQ WindDraw"("Resize to Image Size? (Y)"=FALSE, "Window Number (0...15)"=w241, "Image"=w245) -> ()  [unwired: 7 in, 2 out]
                      }
                      frame #1 {
                        n92 = call "IMAQ WindZoom 2"("Center Point"="Center Point", "Zoom to Fit? (False)"=FALSE, "Zoom Factor"="Zoom Factor") -> ()  [unwired: 5 in, 4 out]
                      }
                    }
                  }
                  frame True {
                    n93 = flat-sequence {
                      tunnel: w250 -> [w253]
                      tunnel: [w251] -> w249
                      tunnel: w249 -> [w255]
                      frame #0 {
                        w252 = TRUE ("Resize to Image Size? (Y)")
                        w251 = 0 ("Window Number (0...15)")
                        n94 = call "IMAQ WindNonTearing"("Window Number"=w251, "NonTearing? (True)"=w252) -> ()  [unwired: 8 in, 2 out]
                        n95 = call "IMAQ WindDraw"("Resize to Image Size? (Y)"=w252, "Window Number (0...15)"=w251, "Image"=w253) -> ()  [unwired: 7 in, 2 out]
                      }
                      frame #1 {
                        n96 = call "IMAQ WindSize"("Scrollbars? (N)"=FALSE, "Width & Height"="Initial Window Size", "Window Number"=w255) -> ()  [unwired: 3 in, 3 out]
                        n97 = call "IMAQ WindMove"("Window Number (0...15)"=w255, "Coordinates (screen)"="Initial Window Position") -> ()  [unwired: 3 in, 2 out]
                      }
                    }
                  }
                }
              }
              frame Enabled {
              }
            }
            n98 = To Unsigned Byte Integer(number=w200) -> (unsigned 8bit integer=w199:u8[][])
            n99 = call "IMAQ ArrayToImage"("Image Pixels (U8)"=w199, "Image"=w196) -> ("Image Out"=w194:T1)  [unwired: 4 in, 5 out]
            n100 = case shown="False" "Save Video" {
              tunnel: w201 -> [_ w259]
              tunnel: w194 -> [_ w258]
              frame False {
              }
              frame True {
                n101 = call "IMAQ AVI Write Frame"("Image"=w258, "Avi Refnum"=w259) -> ()  [unwired: 2 in, 8 out]
              }
            }
            n102 = case shown="False" "Save Image" {
              tunnel: w199 -> [_ w274]
              tunnel: w198 -> [_ w273]
              frame False {
              }
              frame True {
                n103 = call <vilib>:"Flatten Pixmap.vi"("colors"=w273, "8-bit pixmap"=w274) -> ("image data"=w280:T15)  [unwired: 4 in, 5 out]
                n104 = call "Create new save file.vi"("Insert"="video_frame_" ("string"), "Ext"=".bmp" ("string"), "Index In"="Image Index") -> ("Path Out"=w276:path, "Index Out"=w281:dbl)
                n105 = Increment(x=w281) -> (x+1=w275:dbl)
                n106 = local write "Image Index"(w275) -> ()
                n107 = call <vilib>:"Write BMP File.vi"("image data"=w280, "path to BMP file"=w276) -> ()  [unwired: 1 in, 9 out]
              }
            }
            n108 = case shown="False" "Target" {
              tunnel: w194 -> [w220 w224]
              tunnel: [w220 w222] -> w193
              frame False {
              }
              frame True {
                n109 = local read "Target coordinates"() -> (w221:cluster{"X1":dbl, "Y1":dbl, "X2":dbl, "Y2":dbl})
                n110 = call "IMAQ Overlay Oval"("Color"=u32 16711680, "Bounding Rectangle"=w221, "Image"=w224) -> ("Image Out"=w222:T1)  [unwired: 7 in, 1 out]
              }
            }
            "Primary Video Display" <- w193
          }
        }
        n111 = node-c288(w155) -> ()  [unwired: 1 out]
      }
      n112 = node-c288(w139) -> ()  [unwired: 1 out]
      n113 = call "DMR_CloseDevice2.vi"("driver handle IN"=w144) -> ()  [unwired: 3 in, 2 out]
    }
    frame #4 {
      n114 = call "DMR_Close.vi"() -> ()  [unwired: 1 out]
    }
  }
  n115 = while {
    tunnel: [w311] -> w73
    tunnel: [w502] -> w74
    tunnel: [w309] -> w72
    tunnel: [w614] -> w69
    tunnel: w27 -> [w296]
    tunnel: w26 -> [w610]
    tunnel: w25 -> [w615]
    stop <- w614 stop-if-true
    w351 = "NI_ChannelName" ("name")
    w427 = -1
    # "Scan # counter"
    # "DAQ loop iteration\ncounter (for timing)"
    # "Step counter"
    # "Force feedback"
    # "Raster scan"
    # "Rewire everything"
    # "Invert these because changed\nfrom PSD to QPD"
    # "Trap Y"
    # "Trap X"
    # "Convert to\npN"
    # "Convert to\nnm"
    # "Subtract\noffset"
    # "Normalize by\nsum"
    # "B sum"
    # "BX"
    # "BY"
    # "AX"
    # "AY"
    # "A sum"
    # "Close files when done saving"
    n116 = disable-structure shown="Disabled" {
      frame Disabled {
        n117 = property class="DAQmx Read"() -> ("AvailSampPerChan"=→"AvailSampPerChan 2":u32)  [unwired: 2 in, 2 out]
      }
      frame Enabled {
      }
    }
    n118 = local read "Averaging Number"() -> (w319:i32)
    n119 = local read "Averaging Number"() -> (w322:i32)
    "# Samples/channel" <- w322
    n120 = local read "Sampling Rate"() -> (w613:dbl)
    n121 = call-poly <vilib>:"DAQmx Read.vi"("task/channels in"=w296, "number of samples per channel"=w319, "timeout"=10.0) -> ("task out"=w295:refnum<k21>, "data"=w320:dbl[][], "error out"=w430:errorcluster)  [unwired: 10 in]
    n122 = Unbundle By Name(w430) -> ("status"=w550:bool)
    n123 = Divide(x=w613, y="Cal Averaging") -> (x/y=→"Cal Final Sampling Rate":dbl)
    n124 = Divide(x=w613, y=w322) -> (x/y=→"Final Sampling Rate" →"# Samples/channel/s":dbl)
    n125 = disable-structure shown="Disabled" {
      frame Disabled {
        n126 = local read "Buffer size\n(Samples/channel)"() -> (w617:u32)
        n127 = property class="DAQmx Read"() -> ("AvailSampPerChan"=w618:u32)  [unwired: 2 in, 2 out]
        "AvailSampPerChan" <- w618
        n128 = Divide(x=w618, y=w617) -> (x/y=→"Buffer status":dbl)
      }
      frame Enabled {
      }
    }
    n129 = case shown="True" w550 {
      frame False {
      }
      frame True {
        n130 = call <vilib>:"Beep.vi"() -> ()  [unwired: 12 in]
        "Buffer Overflow" <- TRUE
      }
    }
    n131 = local read "Cal values"() -> (w542:T2)
    n132 = Index Array(array=w320, index (row)=4) -> (element=w419:dbl[])  [unwired: 1 in]
    n133 = Index Array(array=w320, index (row)=0) -> (element=w429:dbl[])  [unwired: 1 in]
    n134 = Index Array(array=w320, index (row)=2) -> (element=w424:dbl[])  [unwired: 1 in]
    n135 = Index Array(array=w320, index (row)=1) -> (element=w428:dbl[])  [unwired: 1 in]
    n136 = Index Array(array=w320, index (row)=3) -> (element=w422:dbl[])  [unwired: 1 in]
    n137 = Index Array(array=w320, index (row)=6) -> (element=w421:dbl[])  [unwired: 1 in]
    n138 = Index Array(array=w320, index (row)=7) -> (element=w420:dbl[])  [unwired: 1 in]
    n139 = Index Array(array=w320, index (row)=5) -> (element=w418:dbl[])  [unwired: 1 in]
    n140 = Unbundle(w542) -> ("AX alpha"=w530:dbl, "BX alpha"=w526:dbl, "AX kappa"=w522:dbl, "BX kappa"=w518:dbl, "AX offset"=w536:dbl, "BX offset"=w534:dbl, "AY alpha"=w533:dbl, "BY alpha"=w528:dbl, "AY kappa"=w524:dbl, "BY kappa"=w520:dbl, "AY offset"=w540:dbl, "BY offset"=w538:dbl)
    n141 = Multiply(x=w428, y=w427) -> (x*y=w423:dbl[])
    n142 = Multiply(x=w429, y=w427) -> (x*y=w425:dbl[])
    n143 = local write "AX alpha"(w530) -> ()
    n144 = local write "BY offset"(w538) -> ()
    n145 = Build Array(w425, w424, w423, w422, w421, w420, w419, w418) -> (w348:dbl[][])
    n146 = local write "BX alpha"(w526) -> ()
    n147 = case shown="True" "Reset data stream" {
      selector: "Reset data stream" -> [_ w757]
      tunnel: w295 -> [w749 w755]
      tunnel: [w749 w753] -> w502
      tunnel: w430 -> [w748 w752]
      tunnel: [w748 w750] -> _
      frame False {
      }
      frame True {
        n148 = Not(x=w757) -> (.not. x?=w756:bool)
        n149 = call <vilib>:"DAQmx Stop Task.vi"("task/channels in"=w755, "error in"=w752) -> ("task out"=w754:refnum<k21>, "error out"=w751:errorcluster)  [unwired: 12 in]
        n150 = local write "Reset data stream"(w756) -> ()
        n151 = local write "Buffer Overflow"(w756) -> ()
        n152 = call <vilib>:"DAQmx Start Task.vi"("task/channels in"=w754, "error in"=w751) -> ("task out"=w753:refnum<k21>, "error out"=w750:errorcluster)  [unwired: 12 in]
      }
    }
    n153 = call-poly <vilib>:"Mean.vi"("X"=w418) -> ("mean"=w556:dbl)  [unwired: 1 out]
    n154 = local write "AY offset"(w540) -> ()
    n155 = call-poly <vilib>:"Mean.vi"("X"=w419) -> ("mean"=w557:dbl)  [unwired: 1 out]
    n156 = call-poly <vilib>:"Mean.vi"("X"=w424) -> ("mean"=w563:dbl)  [unwired: 1 out]
    n157 = call-poly <vilib>:"Mean.vi"("X"=w422) -> ("mean"=w561:dbl)  [unwired: 1 out]
    n158 = call-poly <vilib>:"Mean.vi"("X"=w421) -> ("mean"=w560:dbl)  [unwired: 1 out]
    n159 = call-poly <vilib>:"Mean.vi"("X"=w420) -> ("mean"=w559:dbl)  [unwired: 1 out]
    n160 = local read "Averaging Number"() -> (w318:i32)
    n161 = local write "BY kappa"(w520) -> ()
    n162 = local write "AX kappa"(w522) -> ()
    n163 = call-poly <vilib>:"Mean.vi"("X"=w423) -> ("mean"=w562:dbl)  [unwired: 1 out]
    n164 = local write "AY kappa"(w524) -> ()
    n165 = call-poly <vilib>:"Mean.vi"("X"=w425) -> ("mean"=w564:dbl)  [unwired: 1 out]
    n166 = local read "DAQ rate\n(Samples/s)"() -> (w326:dbl)
    n167 = Build Array(w557, w556) -> (w555:dbl[])
    n168 = local write "BX kappa"(w518) -> ()
    n169 = local write "BY alpha"(w528) -> ()
    n170 = local write "AX offset"(w536) -> ()
    n171 = local write "BX offset"(w534) -> ()
    n172 = local write "AY alpha"(w533) -> ()
    n173 = Build Array(w564, w563, w562, w561, w560, w559) -> (w553:dbl[])
    n174 = local read "Total raster time (s)"() -> (w292:dbl)
    n175 = Divide(x=w318, y=w326) -> (x/y=w288:dbl)
    "Data update period (s/set)" <- w288
    n176 = Reciprocal(x=w326) -> (1/x=w327:dbl)
    "Data period (s)" <- w327
    n177 = Divide(x=w292, y=w288) -> (x/y=w291:dbl)
    n178 = Divide(x="Cal time (s)", y=w288) -> (x/y=w287:dbl)
    n179 = Divide(x=w564, y=w560) -> (x/y=w594:dbl)
    n180 = Divide(x=w563, y=w560) -> (x/y=w595:dbl)
    n181 = Round Toward -Infinity(1:w291) -> (0:w290:dbl)
    n182 = Divide(x=w562, y=w559) -> (x/y=w602:dbl)
    n183 = Divide(x=w561, y=w559) -> (x/y=w603:dbl)
    n184 = Round Toward -Infinity(1:w287) -> (0:→"Cal sets to save":dbl)
    n185 = local write "N sets to be saved"(w290) -> ()
    n186 = Subtract(x=w594, y="AY offset") -> (x-y=w576:dbl)
    n187 = Subtract(x=w595, y="AX offset") -> (x-y=w577:dbl)
    n188 = Subtract(x=w602, y="BY offset") -> (x-y=w575:dbl)
    n189 = Subtract(x=w603, y="BX offset") -> (x-y=w578:dbl)
    n190 = Subtract(x=w602, y=w594) -> (x-y=w592:dbl)
    n191 = Subtract(x=w603, y=w595) -> (x-y=w593:dbl)
    n192 = feedback #4(0.0) -> (w501:dbl)
    n193 = Multiply(x="Downsamp\nfact", y=w327) -> (x*y=w328:dbl)
    n194 = Multiply(x=w576, y="AY alpha") -> (x*y=w510:dbl)
    n195 = Multiply(x=w577, y="AX alpha") -> (x*y=w508:dbl)
    n196 = Multiply(x=w578, y="BX alpha") -> (x*y=w509:dbl)
    n197 = Multiply(x=w575, y="BY alpha") -> (x*y=w511:dbl)
    n198 = Add(x=w288, y=w501) -> (x+y=w499:dbl)
    n199 = feedback-in #4(w499) -> ()
    n200 = Square(x=w510) -> (x^2=w586:dbl)
    n201 = Square(x=w508) -> (x^2=w587:dbl)
    n202 = Square(x=w511) -> (x^2=w588:dbl)
    n203 = Square(x=w509) -> (x^2=w589:dbl)
    n204 = Bundle(w592, w593) -> (w321:cluster{dbl, dbl})  [unwired: 1 in]
    n205 = case shown="True" "Set reading to\nsetpoint" {
      tunnel: w321 -> [_ w746]
      frame False {
      }
      frame True {
        n206 = local write "Set reading to\nsetpoint"(FALSE ("Set reading to\nsetpoint")) -> ()
        n207 = local read "Trap position (V)"() -> (w745:cluster{"X":dbl, "Y":dbl})
        n208 = property on="Setpoint voltage" class="Clust (strict)"("Val(Sgnl)"=w746) -> ()  [unwired: 2 in, 2 out]
        n209 = Unbundle(w745) -> ("X"=w744:dbl, "Y"=w743:dbl)
        n210 = Bundle("Y"=w743, "X"=w744) -> (w742:cluster{"Y":dbl, "X":dbl})  [unwired: 1 in]
        n211 = property on="Offset" class="Clust (strict)"("Val(Sgnl)"=w742) -> ()  [unwired: 2 in, 2 out]
      }
    }
    n212 = Reciprocal(x=w328) -> (1/x=→"Chart Freq (Hz)":dbl)
    n213 = To Time Stamp(1:w499) -> (0:w498:timestamp)
    n214 = Add(x=w586, y=w587) -> (x+y=w590:dbl)
    n215 = Add(x=w588, y=w589) -> (x+y=w601:dbl)
    n216 = Multiply(x=w508, y="AX kappa") -> (x*y=w504:dbl)
    n217 = Bundle("A y", "A x", "B y", "B x", "A sum", "B sum", "Trap x", "Trap y") -> (w489:T18)  [unwired: 1 in]
    n218 = Multiply(x=w509, y="BX kappa") -> (x*y=w505:dbl)
    n219 = Square Root(x=w590) -> (sqrt(x)=w606:dbl)
    n220 = Square Root(x=w601) -> (sqrt(x)=w605:dbl)
    n221 = Multiply(x=w510, y="AY kappa") -> (x*y=w506:dbl)
    n222 = Multiply(x=w511, y="BY kappa") -> (x*y=w507:dbl)
    n223 = Subtract(x=w556, y="Fixed Y") -> (x-y=w591:dbl)
    n224 = Subtract(x=w557, y="Fixed X") -> (x-y=w596:dbl)
    n225 = Cluster To Array(cluster=w489) -> (array=w488:string[])
    n226 = for {
      tunnel: w348 -> [w734] mode=indexing
      tunnel: w328 -> [w733]
      tunnel: "Downsamp\nfact" -> [w739]
      tunnel: [w737] -> w404 mode=indexing
      tunnel: w498 -> [w741]
      tunnel: w488 -> [w736] mode=indexing
      tunnel: "NI_ChannelName" ("name") -> [w735]
      n227 = call "Downsample 1D array.vi"("Ave N"=w739, "Arrray In"=w734) -> ("Array Out"=w740:dbl[])  [unwired: 9 in]
      n228 = Bundle By Name("Y"=w740, "dt"=w733, "t0"=w741) -> (w738:waveform(dbl))  [unwired: 1 in]
      n229 = Set Waveform Attribute(5:w736, 6:w735, 7:w738) -> (3:w737:waveform(dbl))  [unwired: 1 in, 2 out]
    }
    "All signals" <- w404
    n230 = Square(x=w506) -> (x^2=w579:dbl)
    n231 = Square(x=w504) -> (x^2=w580:dbl)
    n232 = Square(x=w507) -> (x^2=w581:dbl)
    n233 = Square(x=w505) -> (x^2=w582:dbl)
    n234 = Add(x=w579, y=w580) -> (x+y=w583:dbl)
    n235 = Add(x=w581, y=w582) -> (x+y=w584:dbl)
    n236 = Multiply(x=w591, y="Conv Y (nm/V)") -> (x*y=w513:dbl)
    n237 = Multiply(x=w596, y="Conv X (nm/V)") -> (x*y=w514:dbl)
    n238 = feedback #5() -> (w551:cluster{"B_Y":dbl, "B_X":dbl})  [unwired: 1 in]
    n239 = case shown="True" "Force Feedback" {
      tunnel: [w1031 w1047] -> w312
      tunnel: [w1030 w1046] -> w310
      tunnel: w321 -> [_ w1045]
      tunnel: [cluster{"B_Y":dbl, "B_X":dbl} {"B_Y"=0.0, "B_X"=0.0} ("Sum error past") w1037] -> w552
      tunnel: w551 -> [_ w1044]
      tunnel: w610 -> [w1031 w1040]
      tunnel: w615 -> [w1030 w1039]
      frame False {
        # "Force feedback"
      }
      frame True {
        n240 = call "ForceFeedback2.vi"("PSD/Mirror Voltages"=w1045, "Sum error"=w1044, "task/channels in"=w1040, "error in"=w1039, "Desired voltage"="Setpoint voltage", "Feedback const"="Feedback const", "offset"="Offset") -> ("task out"=w1047:refnum<k21>, "Sum error past"=w1037:cluster{"B_Y":dbl, "B_X":dbl}, "Output Voltage"=→"Feedback Output Voltage 2":cluster{dbl, dbl}, "error out"=w1046:errorcluster)  [unwired: 8 in, 1 out]
        n241 = local read "Pulling direction"() -> (w1036:bool)
        n242 = Unbundle(w1037) -> ("B_Y"=w1034:dbl, "B_X"=w1033:dbl)
        n243 = Select(t=w1034, s=w1036, f=w1033) -> (s? t:f=→"Sum error":dbl)
      }
    }
    n244 = feedback-in #5(w552) -> ()
    n245 = Square Root(x=w583) -> (sqrt(x)=w512:dbl)
    n246 = Square Root(x=w584) -> (sqrt(x)=w607:dbl)
    n247 = Add(x=w512, y=w607) -> (x+y=w585:dbl)
    n248 = Build Array(w594, w595, w602, w603, w560, w559, w512, w607, w606, w605, w514, w513) -> ()  [unwired: 1 out]
    n249 = Divide(x=w585, y=2.0) -> (x/y=w549:dbl)
    n250 = Index Array(array=w404, index=6) -> (element=w353:waveform(dbl))
    n251 = Index Array(array=w404, index=7) -> (element=w355:waveform(dbl))
    n252 = local read "Fixed X"() -> (w408:dbl)
    n253 = local read "Fixed Y"() -> (w410:dbl)
    n254 = Unbundle By Name(w353) -> ("Y"=w412:dbl[])
    n255 = Unbundle By Name(w355) -> ("Y"=w411:dbl[])
    n256 = Index Array(array=w404, index=0) -> (element=w361:waveform(dbl))
    n257 = Index Array(array=w404, index=1) -> (element=w485:waveform(dbl))
    n258 = Index Array(array=w404, index=4) -> (element=w479:waveform(dbl))
    n259 = Subtract(x=w412, y=w408) -> (x-y=w409:dbl[])
    n260 = Subtract(x=w411, y=w410) -> (x-y=w406:dbl[])
    n261 = Unbundle By Name(w361) -> ("Y"=w477:dbl[])
    n262 = Unbundle By Name(w485) -> ("Y"=w476:dbl[])
    n263 = Unbundle By Name(w479) -> ("Y"=w475:dbl[])
    n264 = Index Array(array=w404, index=5) -> (element=w478:waveform(dbl))
    n265 = local read "Conv X (nm/V)"() -> (w407:dbl)
    n266 = local read "Conv Y (nm/V)"() -> (w405:dbl)
    n267 = Index Array(array=w404, index=2) -> (element=w358:waveform(dbl))
    n268 = Index Array(array=w404, index=3) -> (element=w482:waveform(dbl))
    n269 = Set Waveform Attribute(5:"T2 X", 6:w351, 7:w353) -> (3:w352:waveform(dbl))  [unwired: 1 in, 2 out]
    n270 = Set Waveform Attribute(5:"T2 Y", 6:w351, 7:w355) -> (3:w354:waveform(dbl))  [unwired: 1 in, 2 out]
    n271 = Unbundle By Name(w478) -> ("Y"=w472:dbl[])
    n272 = Unbundle By Name(w358) -> ("Y"=w474:dbl[])
    n273 = Unbundle By Name(w482) -> ("Y"=w473:dbl[])
    n274 = Divide(x=w477, y=w475) -> (x/y=w376:dbl[])
    n275 = Divide(x=w476, y=w475) -> (x/y=w374:dbl[])
    n276 = local read "AY offset"() -> (w463:dbl)
    n277 = local read "AX offset"() -> (w461:dbl)
    n278 = Multiply(x=w409, y=w407) -> (x*y=w345:dbl[])
    n279 = Multiply(x=w406, y=w405) -> (x*y=w347:dbl[])
    n280 = Divide(x=w473, y=w472) -> (x/y=w375:dbl[])
    n281 = Subtract(x=w374, y=w461) -> (x-y=w464:dbl[])
    n282 = local read "BY offset"() -> (w468:dbl)
    n283 = local read "BX offset"() -> (w471:dbl)
    n284 = Subtract(x=w376, y=w463) -> (x-y=w465:dbl[])
    n285 = Divide(x=w474, y=w472) -> (x/y=w377:dbl[])
    n286 = local read "AY alpha"() -> (w462:dbl)
    n287 = local read "AX alpha"() -> (w460:dbl)
    n288 = call-poly <vilib>:"Mean.vi"("X"=w347) -> ("mean"=w387:dbl)  [unwired: 1 out]
    "Mean Trp Pos Y 2 (nm)" <- w387
    n289 = Subtract(x=w377, y=w376) -> (x-y=w373:dbl[])
    n290 = Subtract(x=w375, y=w374) -> (x-y=w372:dbl[])
    n291 = Subtract(x=w345, y="Offset X (nm)") -> (x-y=w344:dbl[])
    n292 = Subtract(x=w347, y="Offset Y (nm)") -> (x-y=w346:dbl[])
    n293 = Subtract(x=w377, y=w468) -> (x-y=w470:dbl[])
    n294 = Subtract(x=w375, y=w471) -> (x-y=w469:dbl[])
    n295 = Subtract(x=w387, y=w347) -> (x-y=w386:dbl[])
    n296 = call-poly <vilib>:"Mean.vi"("X"=w345) -> ("mean"=w391:dbl)  [unwired: 1 out]
    "Mean Trap Pos X 2 (nm)" <- w391
    n297 = Build Array(w373, w372) -> (w370:dbl[][])
    n298 = Index Array(array=w370, index (row)=0) -> (element=w368:dbl[])  [unwired: 1 in]
    n299 = Index Array(array=w370, index (row)=1) -> (element=w367:dbl[])  [unwired: 1 in]
    n300 = call-poly <vilib>:"Mean.vi"("X"=w368) -> ("mean"=w366:dbl)  [unwired: 1 out]
    n301 = call-poly <vilib>:"Mean.vi"("X"=w367) -> ("mean"=w365:dbl)  [unwired: 1 out]
    n302 = Bundle("mean"=w366, "mean"=w365) -> ()  [unwired: 1 in, 1 out]
    n303 = local read "BY alpha"() -> (w467:dbl)
    n304 = local read "BX alpha"() -> (w466:dbl)
    n305 = Multiply(x=w465, y=w462) -> (x*y=w453:dbl[])
    n306 = Multiply(x=w464, y=w460) -> (x*y=w452:dbl[])
    n307 = Square(x=w386) -> (x^2=w385:dbl[])
    n308 = Subtract(x=w391, y=w345) -> (x-y=w390:dbl[])
    n309 = Bundle By Name(cluster=w354, "Y"=w346) -> (w402:waveform(dbl))
    n310 = Bundle By Name(cluster=w352, "Y"=w344) -> (w403:waveform(dbl))
    n311 = local read "Raster scanning..."() -> (w294:bool)
    n312 = local read "Saving"() -> (w515:bool)
    n313 = local read "Tether"() -> (w516:bool)
    n314 = Square(x=w390) -> (x^2=w389:dbl[])
    n315 = call-poly <vilib>:"Mean.vi"("X"=w385) -> ("mean"=w384:dbl)  [unwired: 1 out]
    n316 = Square(x=w453) -> (x^2=w459:dbl[])
    n317 = Multiply(x=w470, y=w467) -> (x*y=w451:dbl[])
    n318 = Square(x=w452) -> (x^2=w458:dbl[])
    n319 = Multiply(x=w469, y=w466) -> (x*y=w450:dbl[])
    n320 = Less?(x=w549, y="Tether break\nforce (pN)") -> (x < y?=w547:bool)
    n321 = call-poly <vilib>:"Mean.vi"("X"=w389) -> ("mean"=w388:dbl)  [unwired: 1 out]
    n322 = Build Array(w403, w402) -> (w313:waveform(dbl)[])
    "Trap sep" <- w313
    n323 = Square Root(x=w384) -> (sqrt(x)=w383:dbl)
    n324 = Square(x=w451) -> (x^2=w457:dbl[])
    n325 = Square(x=w450) -> (x^2=w456:dbl[])
    n326 = Add(x=w459, y=w458) -> (x+y=w455:dbl[])
    n327 = Square Root(x=w388) -> (sqrt(x)=w381:dbl)
    n328 = Compound Arithmetic op=AND(w515, w516, w547) -> (w546:bool)
    n329 = Multiply(x=w383, y=10) -> (x*y=→"T2 Y RMS (A)":dbl)
    n330 = Square Root(x=w455) -> (sqrt(x)=w340:dbl[])
    n331 = Add(x=w457, y=w456) -> (x+y=w454:dbl[])
    n332 = Set Waveform Attribute(5:"T2", 6:"NI_ChannelName" ("name"), 7:w361) -> (3:w360:waveform(dbl))  [unwired: 1 in, 2 out]
    n333 = Set Waveform Attribute(5:"T1", 6:"NI_ChannelName" ("name"), 7:w358) -> (3:w357:waveform(dbl))  [unwired: 1 in, 2 out]
    n334 = case shown="True" w546 {
      selector: w546 -> [_ w764]
      tunnel: w294 -> [w758 w759]
      tunnel: [w758 w759] -> w293
      frame False {
      }
      frame True {
        n335 = call <vilib>:"Beep.vi"() -> ()  [unwired: 12 in]
        n336 = Not(x=w764) -> (.not. x?=w762:bool)
        n337 = And(x=w759, y="Fish After TA?") -> (x .and. y?=w761:bool)
        n338 = local write "Tether"(w762) -> ()
        n339 = local write "Force Feedback"(w762) -> ()
        n340 = case shown="True" w761 {
          selector: w761 -> [_ w765]
          frame False {
          }
          frame True {
            n341 = property on="Fish" class="Bool (strict)"("Val(Sgnl)"=w765) -> ()  [unwired: 2 in, 2 out]
          }
        }
        n342 = property on="Stop saving" class="Bool (strict)"("Val(Sgnl)"="TA Cancel Save?") -> ()  [unwired: 2 in, 2 out]
      }
    }
    n343 = Square Root(x=w454) -> (sqrt(x)=w339:dbl[])
    n344 = Multiply(x=w381, y=10) -> (x*y=→"T2 X RMS (A)":dbl)
    n345 = Bundle By Name(cluster=w360, "Y"=w340) -> (w364:waveform(dbl))
    n346 = Bundle By Name(cluster=w357, "Y"=w339) -> (w432:waveform(dbl))
    n347 = Add(x=w340, y=w339) -> (x+y=w338:dbl[])
    n348 = case shown="True" "Remove offsets" {
      selector: "Remove offsets" -> [_ w731]
      frame False {
      }
      frame True {
        n349 = local read "Mean Trp Pos Y 2 (nm)"() -> (w729:dbl)
        n350 = Not(x=w731) -> (.not. x?=w732:bool)
        n351 = local read "Mean Trap Pos X 2 (nm)"() -> (w730:dbl)
        n352 = local write "Remove offsets"(w732) -> ()
        n353 = local write "Offset Y (nm)"(w729) -> ()
        n354 = local write "Offset X (nm)"(w730) -> ()
      }
    }
    n355 = Build Array(w364, w432) -> (→"Bead sep":waveform(dbl)[])
    n356 = local read "AY kappa"() -> (w449:dbl)
    n357 = local read "AX kappa"() -> (w448:dbl)
    n358 = Divide(x=w338, y=2) -> (x/y=w336:dbl[])
    n359 = local read "BX kappa"() -> (w446:dbl)
    n360 = local read "BY kappa"() -> (w447:dbl)
    n361 = call-poly <vilib>:"Mean.vi"("X"=w336) -> ("mean"=w335:dbl)  [unwired: 1 out]
    "Mean Bead Sep\n(nm)" <- w335
    n362 = local read "Calibrating"() -> (w608:bool)
    n363 = Multiply(x=w453, y=w449) -> (x*y=w442:dbl[])
    n364 = Multiply(x=w452, y=w448) -> (x*y=w443:dbl[])
    n365 = Square(x=w442) -> (x^2=w441:dbl[])
    n366 = Square(x=w443) -> (x^2=w440:dbl[])
    n367 = Subtract(x=w336, y=w335) -> (x-y=w334:dbl[])
    n368 = Multiply(x=w451, y=w447) -> (x*y=w444:dbl[])
    n369 = Multiply(x=w450, y=w446) -> (x*y=w445:dbl[])
    n370 = Or(x=w293, y="Raster scan") -> (x .or. y?=w308:bool)
    n371 = Add(x=w441, y=w440) -> (x+y=w437:dbl[])
    n372 = Square(x=w334) -> (x^2=w333:dbl[])
    n373 = Square Root(x=w437) -> (sqrt(x)=w401:dbl[])
    n374 = Square(x=w444) -> (x^2=w439:dbl[])
    n375 = Square(x=w445) -> (x^2=w438:dbl[])
    n376 = call-poly <vilib>:"Mean.vi"("X"=w333) -> ("mean"=w332:dbl)  [unwired: 1 out]
    n377 = Add(x=w439, y=w438) -> (x+y=w436:dbl[])
    n378 = Bundle By Name(cluster=w360, "Y"=w401) -> (w435:waveform(dbl))
    n379 = local read "Saving"() -> (w545:bool)
    n380 = Or(x=w608, y=w545) -> ()  [unwired: 1 out]
    n381 = Square Root(x=w332) -> (sqrt(x)=w331:dbl)
    n382 = Square Root(x=w436) -> (sqrt(x)=w400:dbl[])
    n383 = Multiply(x=10, y=w331) -> (x*y=→"Bead Sep Noise\n(A)":dbl)
    n384 = Bundle By Name(cluster=w357, "Y"=w400) -> (w434:waveform(dbl))
    n385 = Add(x=w401, y=w400) -> (x+y=w399:dbl[])
    n386 = Build Array(w435, w434) -> (→"Force (pN)":waveform(dbl)[])
    n387 = Divide(x=w399, y=2) -> (x/y=w396:dbl[])
    n388 = call-poly <vilib>:"Mean.vi"("X"=w396) -> ("mean"=w397:dbl)  [unwired: 1 out]
    "Mean force (pN)" <- w397
    n389 = Subtract(x=w397, y=w396) -> (x-y=w395:dbl[])
    n390 = Square(x=w395) -> (x^2=w394:dbl[])
    n391 = call-poly <vilib>:"Mean.vi"("X"=w394) -> ("mean"=w393:dbl)  [unwired: 1 out]
    n392 = Square Root(x=w393) -> (sqrt(x)=→"Force noise (pN)":dbl)
    n393 = flat-sequence {
      tunnel: w608 -> [w805]
      tunnel: w545 -> [_]
      tunnel: w608 -> [_]
      tunnel: w545 -> [_]
      tunnel: w348 -> [w792]
      tunnel: [w792] -> w566
      tunnel: w430 -> [w791]
      tunnel: [w791] -> w565
      tunnel: w553 -> [w790]
      tunnel: [w790] -> w558
      tunnel: w555 -> [w789]
      tunnel: [w789] -> w554
      tunnel: [w786] -> w544
      tunnel: [w783] -> w543
      tunnel: [w780] -> w417
      tunnel: [w779] -> w416
      tunnel: [w776] -> w415
      tunnel: w315 -> [w773]
      tunnel: ["Save Data"] -> w314
      tunnel: w566 -> [w953]
      tunnel: w565 -> [w952]
      tunnel: w558 -> [_]
      tunnel: w554 -> [_]
      tunnel: w544 -> [w951]
      tunnel: w543 -> [w950]
      tunnel: w417 -> [w949]
      tunnel: w416 -> [w948]
      tunnel: w415 -> [w947]
      tunnel: w314 -> [w945]
      tunnel: w313 -> [w944]
      frame #0 {
        w771 = 0.0
        # "1: old trap\n0: fleezers"
        # "Create files if saving data"
        n394 = local read "Save N sets"() -> (w775:bool)
        n395 = local read "Sampling Rate"() -> (w803:dbl)
        n396 = Or(x=w775, y="Save Data") -> (x .or. y?=w774:bool)
        n397 = Build Array(w774, "Save cal", w773) -> (w794:bool[])
        n398 = Compound Arithmetic op=OR("Save Data", "Save cal", w773) -> (w796:bool)
        n399 = Boolean Array To Number(Boolean array=w794) -> (number=w793:u32)
        n400 = local read "Trap position (V)"() -> (w800:cluster{"X":dbl, "Y":dbl})
        n401 = local read "Fixed X"() -> (w770:dbl)
        n402 = local read "Fixed Y"() -> (w769:dbl)
        n403 = Unbundle(w800) -> ("X"=w768:dbl, "Y"=w767:dbl)
        n404 = Build Array(w768, w767, w770, w769, w771, w771) -> (w799:dbl[])
        n405 = feedback #6(refnum<k0> refnum) -> (w784:refnum<file>)
        n406 = feedback #7() -> (w781:dbl)  [unwired: 1 in]
        n407 = feedback #8(FALSE) -> (w777:bool)
        n408 = feedback #9(0) -> (w797:i32)
        n409 = feedback #10(refnum<k0> refnum) -> (w787:refnum<file>)
        n410 = case shown="True" w796 {
          tunnel: w805 -> [_ _]
          tunnel: 9 -> [_ w848]
          tunnel: w803 -> [_ w847]
          tunnel: 6 -> [_ w846]
          tunnel: 5 -> [_ w845]
          tunnel: w799 -> [_ w844]
          tunnel: [w810 1] -> w780
          tunnel: w797 -> [w811 _]
          tunnel: w793 -> [_ w819]
          tunnel: [w809 w818] -> w786
          tunnel: w787 -> [w809 _]
          tunnel: [w808 w817] -> w783
          tunnel: w784 -> [w808 _]
          tunnel: 1.0 -> [_ w816]
          tunnel: [w807 w815] -> w779
          tunnel: w781 -> [w807 _]
          tunnel: [w806 w814] -> w776
          tunnel: w777 -> [w806 _]
          frame False {
            n411 = Increment(x=w811) -> (x+1=w810:i32)
          }
          frame True {
            w820 = FALSE ("Save Data")
            w826 = FALSE
            w827 = T17."big-endian, network order" ("byte order (0:big-endian, network order)")
            n412 = local write "Save cal"(w820) -> ()
            n413 = local write "Save Data"(w820) -> ()
            n414 = case shown="4" w819 {
              tunnel: w848 -> [w895 w913 w943]
              tunnel: w847 -> [w873 w912 w918]
              tunnel: w846 -> [w894 w910 w939]
              tunnel: w845 -> [w893 w909 w938]
              tunnel: w844 -> [w891 w906 w935]
              tunnel: [w890 w905 w924] -> w841
              tunnel: [w892 w902 w923] -> w814
              tunnel: ["Averaging Number" 200 w921] -> _
              tunnel: w816 -> [w878 w897 w920]
              tunnel: [w874 w896 w914] -> w815
              frame 1, Default {
                w892 = TRUE
                w879 = 0.0
                # "Time trace"
                n415 = local read "Averaging Number"() -> (w889:i32)
                n416 = Boolean To (0,1)(Boolean=w892) -> (0, 1=w884:i16)
                n417 = Increment(x=w884) -> (x+1=w883:i16)
                n418 = Divide(x=w873, y=w889) -> (x/y=w888:dbl)
                n419 = To Double Precision Float(number=w883) -> (double precision float=w882:dbl)
                n420 = Reciprocal(x=w888) -> (1/x=w887:dbl)
                n421 = Reciprocal(x=w873) -> (1/x=w872:dbl)
                n422 = Build Array(w895, w872, w887, w894, w893, 0 ("f")) -> (w886:dbl[])
                n423 = Build Array(w882, w878, w879, w879, w879) -> (w885:dbl[])
                n424 = Build Array (concatenate)(w886, w891, w885) -> (w890:dbl[])
                n425 = Select(t="N sets", s="Save N sets", f=2147483647) -> (s? t:f=w874:i32)
              }
              frame 2 {
                w902 = FALSE
                w900 = 0.0
                # "Calibration file"
                n426 = Reciprocal(x=w912) -> (1/x=w911:dbl)
                n427 = Boolean To (0,1)(Boolean=w902) -> (0, 1=w904:i16)
                n428 = To Double Precision Float(number=w904) -> (double precision float=w903:dbl)
                n429 = Build Array(w913, w911, w911, w910, w909, 1) -> (w907:dbl[])
                n430 = Build Array(w903, w897, w900, w900, w900) -> (w901:dbl[])
                n431 = Build Array (concatenate)(w907, w906, w901) -> (w905:dbl[])
                n432 = local read "Cal sets to save"() -> (w896:i32)
                "Calibrating" <- TRUE ("Calibrating")
              }
              frame 4 {
                w931 = 0.0
                w923 = TRUE
                # "Not using ncycles"
                # "FX curve"
                n433 = local read "Averaging Number"() -> (w942:i32)
                n434 = Boolean To (0,1)(Boolean=w923) -> (0, 1=w934:i16)
                n435 = Increment(x=w934) -> (x+1=w933:i16)
                n436 = local write "Raster scan"(FALSE ("Raster scan")) -> ()
                n437 = To Double Precision Float(number=w933) -> (double precision float=w932:dbl)
                n438 = Divide(x=w918, y=w942) -> (x/y=w941:dbl)
                n439 = Reciprocal(x=w941) -> (1/x=w940:dbl)
                n440 = Build Array(w932, w920, w931, w931, w931) -> (w930:dbl[])
                n441 = Reciprocal(x=w918) -> (1/x=w917:dbl)
                n442 = Build Array(w943, w917, w940, w939, w938, 2) -> (w936:dbl[])
                n443 = local read "Pulling direction"() -> (w928:bool)
                n444 = local read "Scan range (V)"() -> (w915:dbl)
                n445 = local read "N sets to be saved"() -> (w914:dbl)
                n446 = local read "Scan steps (mirror)"() -> (w916:u64)
                n447 = local read "# scans"() -> (w926:i32)
                n448 = Not(x=w928) -> (.not. x?=w927:bool)
                n449 = local read "Averaging Number"() -> (w921:i32)
                n450 = Boolean To (0,1)(Boolean=w927) -> (0, 1=w929:i16)
                n451 = Build Array(w929, w915, w916, 0, w926) -> (w925:dbl[])
                n452 = Build Array (concatenate)(w936, w935, w930, w925) -> (w924:dbl[])
              }
            }
            n453 = call "CreateSaveFile.vi"("Index In"="Save file index", "Ext"=".dat", "Insert"="", "Directory"="Path") -> ("Index Out"=w813:i32, "Path Out"=w825:path)  [unwired: 6 in]
            "Current file name" <- w825
            n454 = Open/Create/Replace File(file path (use dialog)=w825, operation (0:open)=T16."create", access (0:read/write)=enum16{"read/write", "read-only", "write-only"}."write-only") -> (refnum out=w834:refnum<file>, error out=w835:errorcluster)  [unwired: 3 in, 1 out]
            n455 = local write "Save file index"(w813) -> ()
            n456 = Array Size(array=w841) -> (size(s)=w843:i32)
            n457 = case shown="True" w814 {
              tunnel: w825 -> [_ w871]
              tunnel: [refnum<k0> refnum w850] -> w817
              frame False {
              }
              frame True {
                w857 = 0.0
                n458 = Path To String(path=w871) -> (string=w867:string)
                n459 = Build Array(w857, w857, w857, w857, w857, w857, w857, w857) -> (w854:dbl[])
                n460 = String Length(string=w867) -> (length=w870:i32)
                n461 = Array Size(array=w854) -> (size(s)=w856:i32)
                n462 = Subtract(x=w870, y=4) -> (x-y=w868:i32)
                n463 = To Double Precision Float(number=w856) -> (double precision float=w855:dbl)
                n464 = String Subset(string=w867, length (rest)=w868) -> (substring=w866:string)  [unwired: 1 in]
                n465 = Build Array (concatenate)(w855, w854) -> (w853:dbl[])
                n466 = Concatenate Strings(w866, "_pos.dat" ("string")) -> (w864:string)
                n467 = String To Path(string=w864) -> (path=w863:path)
                n468 = Open/Create/Replace File(file path (use dialog)=w863, operation (0:open)=T16."create", access (0:read/write)=enum16{"read/write", "read-only", "write-only"}."write-only") -> (refnum out=w859:refnum<file>, error out=w860:errorcluster)  [unwired: 3 in, 1 out]
                n469 = Deny Access(4:w860, 7:w859) -> (3:w858:refnum<file>)  [unwired: 1 in, 1 out]
                n470 = Write to Binary File(file (use dialog)=w858, data=w853, 5:FALSE ("prepend array or string size? (T)"), 9:T17."big-endian, network order" ("byte order (0:big-endian, network order)")) -> (refnum out=w850:refnum<file>)  [unwired: 2 in, 2 out]
              }
            }
            n471 = Deny Access(4:w835, 7:w834) -> (0:w824:errorcluster, 3:w833:refnum<file>)  [unwired: 1 in]
            n472 = String Length(string="Comment") -> (length=w840:i32)
            n473 = To Double Precision Float(number=w843) -> (double precision float=w842:dbl)
            n474 = To Double Precision Float(number=w840) -> (double precision float=w839:dbl)
            n475 = Build Array (concatenate)(w842, w841, w839) -> (w830:dbl[])
            n476 = Write to Binary File(file (use dialog)=w833, data=w830, error in=w824, 5:w826, 9:w827) -> (refnum out=w829:refnum<file>, error out=w823:errorcluster)  [unwired: 1 in, 1 out]
            n477 = Write to Binary File(file (use dialog)=w829, data="Comment", error in=w823, 5:w826, 9:w827) -> (refnum out=w818:refnum<file>)  [unwired: 1 in, 2 out]
            "Saving" <- TRUE
          }
        }
        n478 = feedback-in #6(w783) -> ()
        n479 = feedback-in #7(w779) -> ()
        n480 = feedback-in #8(w776) -> ()
        n481 = feedback-in #9(w780) -> ()
        n482 = feedback-in #10(w786) -> ()
      }
      frame #1 {
        n483 = local read "Saving"() -> (w946:bool)
        n484 = case shown="True" w946 {
          tunnel: w953 -> [_ w972]
          tunnel: w952 -> [_ w971]
          tunnel: w951 -> [_ w970]
          tunnel: w950 -> [_ w969]
          tunnel: w949 -> [_ w959]
          tunnel: w948 -> [_ w960]
          tunnel: w947 -> [_ w963]
          tunnel: w945 -> [_ w955]
          tunnel: w944 -> [_ w954]
          frame False {
            (unwired) FALSE ("Calibrating")
          }
          frame True {
            n485 = local read "Stop"() -> (w967:bool)
            n486 = Less Or Equal?(x=w959, y=w960) -> (x <= y?=w968:bool)
            n487 = Divide(x=w959, y=w960) -> (x/y=w958:dbl)
            n488 = Or(x=w967, y="Stop saving") -> (x .or. y?=w966:bool)
            n489 = Not(x=w966) -> (.not. x?=w965:bool)
            n490 = Multiply(x=100.0, y=w958) -> (x*y=w957:dbl)
            n491 = And(x=w968, y=w965) -> (x .and. y?=w964:bool)
            n492 = case shown="False" w964 {
              tunnel: w970 -> [w977 w986]
              tunnel: w971 -> [_ w985]
              tunnel: w972 -> [_ w984]
              tunnel: w969 -> [w976 w983]
              tunnel: w963 -> [w974 _]
              tunnel: [0.0 ("Progress") w982] -> w962
              tunnel: w957 -> [_ w982]
              tunnel: w955 -> [_ w979]
              tunnel: w954 -> [_ w980]
              frame False {
                w975 = FALSE
                n493 = Close File(refnum=w977) -> ()  [unwired: 1 in, 2 out]
                n494 = case shown="True" w974 {
                  tunnel: w976 -> [_ w978]
                  frame False {
                  }
                  frame True {
                    n495 = Close File(refnum=w978) -> ()  [unwired: 1 in, 2 out]
                  }
                }
                n496 = call <vilib>:"Beep.vi"() -> ()  [unwired: 12 in]
                n497 = local write "Saving"(w975) -> ()
                n498 = local write "Stop saving"(w975) -> ()
                n499 = local write "Calibrating"(w975) -> ()
              }
              frame True {
                n500 = local read "Calibrating"() -> (w981:bool)
                n501 = case shown="True" w981 {
                  tunnel: w986 -> [w1013 w1029]
                  tunnel: w985 -> [_ w1028]
                  tunnel: w984 -> [w1000 w1022]
                  tunnel: w983 -> [w999 _]
                  tunnel: w980 -> [w991 _]
                  tunnel: w979 -> [_ _]
                  frame False {
                    n502 = local read "Averaging Number"() -> (w1007:i32)
                    n503 = Array Subset(array=w1000, index (row)=0 ("index"), length (row)=6 ("length")) -> (w996:dbl[][])  [unwired: 2 in]
                    n504 = Array Subset(array=w1000, index (row)=6 ("index"), length (row)=2 ("length")) -> (w995:dbl[][])  [unwired: 2 in]
                    n505 = Array Size(array=w995) -> (size(s)=w1006:i32[])
                    n506 = Array Size(array=w996) -> (size(s)=w1003:i32[])
                    n507 = Index Array(array=w991, index=0) -> (element=w988:waveform(dbl))
                    n508 = Index Array(array=w991, index=1) -> (element=w987:waveform(dbl))
                    n509 = for {
                      tunnel: w996 -> [w1017] mode=indexing
                      tunnel: w1007 -> [w1019]
                      tunnel: [w1018] -> w994 mode=indexing
                      n510 = call "Downsample 1D array.vi"("Ave N"=w1019, "Arrray In"=w1017) -> ("Array Out"=w1018:dbl[])  [unwired: 9 in]
                    }
                    n511 = Unbundle By Name(w988) -> ()  [unwired: 1 out]
                    n512 = Unbundle By Name(w987) -> ()  [unwired: 1 out]
                    n513 = Multiply Array Elements(1:w1003) -> (0:w1002:i32)
                    n514 = for {
                      tunnel: w995 -> [w1016] mode=indexing
                      tunnel: w1007 -> [w1015]
                      tunnel: [w1014] -> w998 mode=indexing
                      n515 = call "Downsample 1D array.vi"("Ave N"=w1015, "Arrray In"=w1016) -> ("Array Out"=w1014:dbl[])  [unwired: 9 in]
                    }
                    n516 = Multiply Array Elements(1:w1006) -> (0:w1005:i32)
                    n517 = Divide(x=w1002, y=w1007) -> (x/y=w1008:dbl)
                    n518 = Divide(x=w1005, y=w1007) -> (x/y=w1004:dbl)
                    n519 = Transpose 2D Array(2D array=w994) -> (transposed array=w993:dbl[][])
                    n520 = Transpose 2D Array(2D array=w998) -> (transposed array=w992:dbl[][])
                    n521 = Reshape Array(w993, w1008) -> (w997:dbl[])
                    n522 = Reshape Array(w992, w1004) -> (w1001:dbl[])
                    n523 = call <vilib>:"Write File+ [SGL].vi"("1D array"=w1001, "refnum"=w999) -> ()  [unwired: 7 in, 3 out]
                    n524 = call <vilib>:"Write File+ [SGL].vi"("1D array"=w997, "refnum"=w1013) -> ()  [unwired: 7 in, 3 out]
                  }
                  frame True {
                    n525 = Array Subset(array=w1022, index (row)=0 ("index"), length (row)=6 ("length")) -> (w1020:dbl[][])  [unwired: 2 in]
                    n526 = Transpose 2D Array(2D array=w1020) -> (transposed array=w1026:dbl[][])
                    n527 = Array Size(array=w1020) -> (size(s)=w1021:i32[])
                    n528 = Multiply Array Elements(1:w1021) -> (0:w1027:i32)
                    n529 = Reshape Array(w1026, w1027) -> (w1025:dbl[])
                    n530 = call <vilib>:"Write File+ [SGL].vi"("1D array"=w1025, "error in (no error)"=w1028, "refnum"=w1029) -> ()  [unwired: 6 in, 3 out]
                  }
                }
              }
            }
            "Progress" <- w962
          }
        }
      }
    }
    n531 = local read "Flushing Sample"() -> (w317:bool)
    n532 = case shown="True" w317 {
      frame False {
      }
      frame True {
        n533 = local read "Flush Sample Start Time"() -> (w725:u32)
        n534 = local read "Sample flush time (s)"() -> (w718:dbl)
        n535 = Tick Count (ms)() -> (millisecond timer value=w726:u32)
        n536 = Subtract(x=w726, y=w725) -> (x-y=w716:u32)
        n537 = Multiply(x=u32 1000, y=w718) -> (x*y=w717:dbl)
        n538 = Divide(x=w716, y=w717) -> (x/y=w721:dbl)
        n539 = Greater?(x=w716, y=w717) -> (0:w724:bool)
        n540 = Not(x=w724) -> (.not. x?=w723:bool)
        n541 = Boolean To (0,1)(Boolean=w723) -> (0, 1=w722:i16)
        n542 = Compound Arithmetic op=MULTIPLY(w722, w721, 100.0 ("value")) -> (→"Sample Flush Meter":dbl)
        n543 = case shown="True" w724 {
          frame False {
          }
          frame True {
            w728 = FALSE ("Inject Sample")
            n544 = property on="Clear Volume" class="Bool (strict)"("Val(Sgnl)"=TRUE ("Value (Signaling)")) -> ()  [unwired: 2 in, 2 out]
            n545 = local write "Inject Sample"(w728) -> ()
            n546 = local write "Flushing Sample"(w728) -> ()
          }
        }
      }
    }
    n547 = feedback #11(0) -> (w301:i32)
    n548 = feedback #12(0) -> (w298:i32)
    n549 = feedback #13(0) -> (w303:i32)
    n550 = case shown="True" w308 {
      tunnel: w312 -> [w626 w674]
      tunnel: [w626 w658] -> w311
      tunnel: w310 -> [w625 w673]
      tunnel: [w625 w657] -> w309
      tunnel: "Raster scan" -> [w624 w650]
      tunnel: [w624 w649] -> w306
      tunnel: [0 w648] -> w304
      tunnel: w303 -> [_ w642]
      tunnel: w301 -> [_ w630]
      tunnel: [0 w633] -> w300
      tunnel: w298 -> [_ w639]
      tunnel: [0 w638] -> w297
      frame False {
      }
      frame True {
        # "Reset step counter"
        # "Current position"
        # "Initial values"
        n551 = disable-structure shown="Disabled" {
          frame Disabled {
            n552 = local write "Raster scan"(FALSE ("Raster scan")) -> ()
            n553 = property on="Reset data stream" class="Bool (strict)"("Val(Sgnl)"=TRUE) -> ()  [unwired: 2 in, 2 out]
          }
          frame Enabled {
          }
        }
        n554 = local read "Data update period (s/set)"() -> (w647:dbl)
        n555 = local read "Time per step (ms)"() -> (w644:dbl)
        n556 = local read "Trap position (V)"() -> (w629:cluster{"X":dbl, "Y":dbl})
        n557 = local read "Fixed X"() -> (w667:dbl)
        n558 = local read "Fixed Y"() -> (w668:dbl)
        n559 = Unbundle(w629) -> ("X"=w627:dbl, "Y"=w628:dbl)
        n560 = local read "Scan steps (mirror)"() -> (w656:u64)
        n561 = Multiply(x=w647, y=1000.0) -> (x*y=w645:dbl)
        n562 = local read "Stop raster"() -> (w663:bool)
        n563 = local read "Stop saving"() -> (w664:bool)
        n564 = Select(t=w667, s="Pulling direction", f=w668) -> (s? t:f=w675:dbl)
        n565 = Divide(x=w644, y=w645) -> (x/y=w643:dbl)
        n566 = Quotient & Remainder(x=w642, y=w643) -> (x-y*floor(x/y)=w641:dbl)  [unwired: 1 out]
        n567 = Not(x=w663) -> (.not. x?=w662:bool)
        n568 = Not(x=w664) -> (.not. x?=w661:bool)
        n569 = Multiply(x=u64 2, y=w656) -> (x*y=w652:u64)
        n570 = Select(t=w628, s="Pulling direction", f=w627) -> (s? t:f=w651:dbl)
        n571 = Equal To 0?(x=w641) -> (x = 0?=w640:bool)
        n572 = Less?(x=w630, y=w652) -> (x < y?=w653:bool)
        n573 = Compound Arithmetic op=AND(w653, w662, w661, w640) -> (w654:bool)
        n574 = Not(x=w653) -> (.not. x?=w636:bool)
        n575 = feedback #14() -> (w659:dbl)  [unwired: 1 in]
        n576 = case shown="True" w654 {
          tunnel: w675 -> [_ w711]
          tunnel: w651 -> [_ w693]
          tunnel: w674 -> [w688 w710]
          tunnel: w673 -> [w687 w709]
          tunnel: [w688 w708] -> w658
          tunnel: [w687 w707] -> w657
          tunnel: [w684 w696] -> w660
          tunnel: w630 -> [w685 w691]
          tunnel: w659 -> [w684 w690]
          tunnel: w650 -> [w686 w695]
          tunnel: [w686 w695] -> w649
          tunnel: [w685 w694] -> w634
          frame False {
          }
          frame True {
            # "Go forward or backward?"
            n577 = local read "Scan increment (V)"() -> (w689:dbl)
            n578 = local read "Scan steps (mirror)"() -> (w700:u64)
            n579 = Multiply(x=w689, y=w691) -> (x*y=w692:dbl)
            n580 = Less?(x=w691, y=w700) -> (x < y?=w699:bool)
            n581 = Add(x=w693, y=w692) -> (x+y=w702:dbl)
            n582 = Subtract(x=w690, y=w689) -> (x-y=w701:dbl)
            n583 = Select(t=w702, s=w699, f=w701) -> (s? t:f=w696:dbl)
            n584 = local read "Pulling direction"() -> (w698:bool)
            n585 = Build Array(w696, w711) -> (w705:dbl[])
            n586 = Build Array(w711, w696) -> (w704:dbl[])
            n587 = Select(t=w705, s=w698, f=w704) -> (s? t:f=w703:dbl[])
            n588 = call-poly <vilib>:"DAQmx Write.vi"("task/channels in"=w710, "auto start"=TRUE, "data"=w703, "error in"=w709) -> ("task out"=w708:refnum<k21>, "error out"=w707:errorcluster)  [unwired: 9 in, 1 out]
            n589 = Increment(x=w691) -> (x+1=w694:i32)
            "Raster scanning..." <- TRUE ("Raster scanning...")
          }
        }
        n590 = feedback-in #14(w660) -> ()
        n591 = case shown="True" w636 {
          tunnel: w639 -> [w681 w683]
          tunnel: [w681 w682] -> w638
          frame False {
          }
          frame True {
            n592 = Increment(x=w683) -> (x+1=w682:i32)
          }
        }
        n593 = local read "# scans"() -> (w637:i32)
        n594 = local read "Stop saving"() -> (w666:bool)
        n595 = Greater Or Equal?(x=w638, y=w637) -> (x >= y?=w631:bool)
        n596 = Not(x=w631) -> (.not. x?=w632:bool)
        n597 = And(x=w636, y=w632) -> (x .and. y?=w635:bool)
        n598 = Compound Arithmetic op=OR(w631, "Stop raster", w666) -> (w669:bool)
        n599 = case shown="True" w669 {
          frame False {
          }
          frame True {
            n600 = flat-sequence {
              frame #0 {
                n601 = Wait (ms)(milliseconds to wait=u32 300) -> ()  [unwired: 1 out]
              }
              frame #1 {
                n602 = property on="Trap delta (nm)" class="DigNum (strict)"("Val(Sgnl)"="Trap delta\nafter (nm)") -> ()  [unwired: 2 in, 2 out]
              }
            }
          }
        }
        n603 = And(x="Flow on\nafter raster?", y=w669) -> (x .and. y?=w670:bool)
        n604 = case shown="True" w670 {
          frame False {
          }
          frame True {
            n605 = property on="Inject Sample" class="Bool (strict)"("Val(Sgnl)"=TRUE ("Value (Signaling)")) -> ()  [unwired: 2 in, 2 out]
          }
        }
        n606 = case shown="True" w635 {
          tunnel: w634 -> [w679 _]
          tunnel: [w679 0] -> w633
          frame False {
          }
          frame True {
          }
        }
        n607 = Not(x=w669) -> (.not. x?=w672:bool)
        n608 = local write "Raster scanning..."(w672) -> ()
        n609 = Increment(x=w642) -> (x+1=w648:i32)
      }
    }
    n610 = And(x="Save scans", y=w306) -> (x .and. y?=w315:bool)
    n611 = feedback-in #11(w300) -> ()
    n612 = feedback-in #12(w297) -> ()
    n613 = feedback-in #13(w304) -> ()
    n614 = local read "Stop"() -> (w614:bool)
  }
  n615 = local write "Progress"(u8 0 ("Progress")) -> ()
  n616 = local write "Calibrating"(FALSE ("Calibrating")) -> ()
  n617 = call-poly "VISA Configure Serial Port"("VISA resource name"=refnum<visa-resource-name> "COM6") -> ("VISA resource name out"=w17:refnum<visa-resource-name>, "error out"=w16:errorcluster)  [unwired: 13 in]
  n618 = node-c288(i64 100 ("Period"), 2 ("Processor")) -> (w19:T11)  [unwired: 2 in]
  n619 = timed-loop {
    timing: w19 -> [_]
    timing-out: [_] -> w18
    tunnel: w17 -> [w1048]
    tunnel: w16 -> [w1050]
    tunnel: [w1048] -> w15
    stop <- w1049 stop-if-true
    n620 = node-c288() -> ()  [unwired: 1 in, 1 out]
    n621 = event shown="[3] \"Got ADig bead\": Value Change" {
      selector: _ -> [_ _ _ _ _ _ _ _ _ _ _ _]
      dyn-events: _ -> [_ _ _ _ _ _ _ _ _ _ _ _]
      timeout: _ -> [_ _ _ _ _ _ _ _ _ _ _ _]
      tunnel: w1048 -> [w1057 w1096 w1116 w1133 w1150 w1169 w1192 w1202 _ _ _ _]
      tunnel: w1050 -> [w1056 w1095 w1115 w1132 w1149 w1168 w1191 w1201 _ _ _ _]
      tunnel: [_ _ _ _ _ _ _ _ _ _ _ w1255] -> w1049
      event "Got DNA bead": Value Change {
        n622 = event-data() -> ()  [unwired: 1 in, 5 out]
        n623 = flat-sequence {
          tunnel: w1057 -> [w1061]
          tunnel: w1056 -> [w1059]
          tunnel: [w1076] -> w1055
          tunnel: w1055 -> [w1079]
          tunnel: [w1079] -> w1054
          tunnel: w1054 -> [w1081]
          tunnel: [w1081] -> w1053
          tunnel: w1053 -> [w1085]
          tunnel: [w1085] -> w1052
          tunnel: w1052 -> [w1087]
          tunnel: [w1087] -> w1051
          tunnel: w1051 -> [w1089]
          frame #0 {
            n624 = local read "Saved stage positions"() -> (w1062:dbl[][])
            n625 = disable-structure shown="Disabled" {
              frame Disabled {
                n626 = property on="Inject Pump 2" class="Bool (strict)"("Val(Sgnl)"=FALSE ("Inject Pump 2")) -> ()  [unwired: 2 in, 2 out]
              }
              frame Enabled {
              }
            }
            n627 = property on="Inject Sample" class="Bool (strict)"("Val(Sgnl)"=TRUE ("Value (Signaling)")) -> ()  [unwired: 2 in, 2 out]
            n628 = local write "Stage moving"(TRUE ("Stage moving")) -> ()
            n629 = property on="Trap delta (nm)" class="DigNum (strict)"("Val(Sgnl)"="Cal @ Delta (nm)") -> ()  [unwired: 2 in, 2 out]
            n630 = call "move to saved stage position.vi"("error in"=w1059, "Stage VISA resource name in"=w1061, "Position"="Cal stage position", "Saved Stage Positions"=w1062) -> ()  [unwired: 2 out]
          }
          frame #1 {
            n631 = local write "Stage moving"(FALSE ("Stage moving")) -> ()
            n632 = property on="Inject Sample" class="Bool (strict)"("Val(Sgnl)"=FALSE ("Value (Signaling)")) -> ()  [unwired: 2 in, 2 out]
            n633 = call <vilib>:"Beep.vi"() -> ()  [unwired: 12 in]
          }
          frame #2 {
            n634 = Wait (ms)(milliseconds to wait=u32 1000) -> ()  [unwired: 1 out]
          }
          frame #3 {
            n635 = property on="Save cal" class="Bool (strict)"("Val(Sgnl)"=TRUE ("Value (Signaling)")) -> ()  [unwired: 2 in, 2 out]
          }
          frame #4 {
            n636 = Wait (ms)(milliseconds to wait=u32 2000) -> ()  [unwired: 1 out]
          }
          frame #5 {
            n637 = while {
              stop <- w1072 stop-if-true
              n638 = local read "Saving"() -> (w1073:bool)
              n639 = Not(x=w1073) -> (.not. x?=w1072:bool)
              n640 = Wait (ms)(milliseconds to wait=u32 100) -> ()  [unwired: 1 out]
            }
          }
          frame #6 {
            n641 = Wait (ms)(milliseconds to wait=u32 2000) -> ()  [unwired: 1 out]
            n642 = property on="Trap delta (nm)" class="DigNum (strict)"("Val(Sgnl)"="Offset @ Delta (nm)") -> ()  [unwired: 2 in, 2 out]
          }
          frame #7 {
            # "Only continue if there is no buffer\noverflow error"
            n643 = local read "Buffer Overflow"() -> (w1077:bool)
            n644 = Not(x=w1077) -> (.not. x?=w1076:bool)
            n645 = case shown="True" w1076 {
              frame False {
              }
              frame True {
                n646 = property on="Raster scan" class="Bool (strict)"("Val(Sgnl)"=TRUE ("Value (Signaling)")) -> ()  [unwired: 2 in, 2 out]
              }
            }
          }
          frame #8 {
            n647 = case shown="True" w1079 {
              frame False {
              }
              frame True {
                n648 = Wait (ms)(milliseconds to wait=u32 2000) -> ()  [unwired: 1 out]
              }
            }
          }
          frame #9 {
            n649 = case shown="True" w1081 {
              frame False {
              }
              frame True {
                n650 = while {
                  stop <- w1083 stop-if-true
                  n651 = local read "Saving"() -> (w1084:bool)
                  n652 = Not(x=w1084) -> (.not. x?=w1083:bool)
                  n653 = Wait (ms)(milliseconds to wait=u32 100) -> ()  [unwired: 1 out]
                }
              }
            }
          }
          frame #10 {
            n654 = case shown="True" w1085 {
              frame False {
              }
              frame True {
                n655 = property on="Read Cal" class="Bool (strict)"("Val(Sgnl)"=TRUE ("Value (Signaling)")) -> ()  [unwired: 2 in, 2 out]
              }
            }
          }
          frame #11 {
            n656 = case shown="True" w1087 {
              frame False {
              }
              frame True {
                n657 = Wait (ms)(milliseconds to wait=u32 1000) -> ()  [unwired: 1 out]
              }
            }
          }
          frame #12 {
            n658 = case shown="True" w1089 {
              frame False {
              }
              frame True {
                n659 = property on="Fish" class="Bool (strict)"("Val(Sgnl)"=TRUE ("Value (Signaling)")) -> ()  [unwired: 2 in, 2 out]
                n660 = case shown="True" "Flow on\nwhile fish?" {
                  frame False {
                  }
                  frame True {
                    n661 = property on="Inject Sample" class="Bool (strict)"("Val(Sgnl)"=TRUE ("Value (Signaling)")) -> ()  [unwired: 2 in, 2 out]
                  }
                }
              }
            }
          }
        }
      }
      event "Dump beads": Value Change {
        n662 = event-data() -> ()  [unwired: 1 in, 5 out]
        n663 = flat-sequence {
          tunnel: w1095 -> [w1099]
          tunnel: w1096 -> [w1100]
          tunnel: [w1100] -> w1094
          tunnel: [w1099] -> w1093
          tunnel: w1094 -> [w1103]
          tunnel: w1093 -> [w1102]
          frame #0 {
            w1097 = FALSE ("Fish")
            n664 = local read "Saving"() -> (w1098:bool)
            n665 = local write "Pause dwell"(w1097) -> ()
            n666 = local write "Force Feedback"(w1097) -> ()
            n667 = local write "Dump beads"(w1097) -> ()
            n668 = property on="Stop saving" class="Bool (strict)"("Val(Sgnl)"=w1098) -> ()  [unwired: 2 in, 2 out]
            n669 = local write "Fish"(w1097) -> ()
          }
          frame #1 {
            n670 = local read "Saved stage positions"() -> (w1105:dbl[][])
            n671 = case shown="True" "Flow on\ndump?" {
              frame False {
              }
              frame True {
                n672 = property on="Inject Sample" class="Bool (strict)"("Val(Sgnl)"=TRUE ("Value (Signaling)")) -> ()  [unwired: 2 in, 2 out]
              }
            }
            n673 = local write "Stage moving"(TRUE ("Stage moving")) -> ()
            n674 = call "move to saved stage position.vi"("error in"=w1102, "Stage VISA resource name in"=w1103, "Position"=5, "Saved Stage Positions"=w1105) -> ()  [unwired: 2 out]
          }
          frame #2 {
            n675 = local read "Shutter 1 (B)"() -> (w1110:bool)
            n676 = local read "Shutter 2 (A)"() -> (w1109:bool)
            n677 = call <vilib>:"Beep.vi"() -> ()  [unwired: 12 in]
            n678 = case shown="True" w1110 {
              frame False {
              }
              frame True {
                n679 = property on="Shutter 1 (B)" class="Bool (strict)"("Val(Sgnl)"=FALSE ("Value (Signaling)")) -> ()  [unwired: 2 in, 2 out]
              }
            }
            n680 = case shown="True" w1109 {
              frame False {
              }
              frame True {
                n681 = property on="Shutter 2 (A)" class="Bool (strict)"("Val(Sgnl)"=FALSE) -> ()  [unwired: 2 in, 2 out]
              }
            }
            n682 = local write "Stage moving"(FALSE ("Stage moving")) -> ()
            n683 = local write "Tether"(FALSE ("Tether")) -> ()
          }
          frame #3 {
            n684 = property on="Move Cap. 2 (ADig Top)" class="Bool (strict)"("Val(Sgnl)"=TRUE ("Value (Signaling)")) -> ()  [unwired: 2 in, 2 out]
          }
        }
      }
      event "Move Cap. 2 (ADig Top)": Value Change {
        n685 = event-data() -> ()  [unwired: 1 in, 5 out]
        n686 = flat-sequence {
          tunnel: w1116 -> [w1120]
          tunnel: w1115 -> [w1119]
          frame #0 {
            n687 = local read "Saved stage positions"() -> (w1118:dbl[][])
            n688 = case shown="True" "Flow on\ncap 2?" {
              frame False {
              }
              frame True {
                n689 = property on="Inject Sample" class="Bool (strict)"("Val(Sgnl)"=TRUE ("Value (Signaling)")) -> ()  [unwired: 2 in, 2 out]
              }
            }
            n690 = local write "Move Cap. 2 (ADig Top)"(FALSE ("Move Cap. 2 (ADig Top)")) -> ()
            n691 = local write "Stage moving"(TRUE ("Stage moving")) -> ()
            n692 = call "move to saved stage position.vi"("error in"=w1119, "Stage VISA resource name in"=w1120, "Position"=2, "Saved Stage Positions"=w1118) -> ()  [unwired: 2 out]
          }
          frame #1 {
            # "Make sure you don't reverse\nwhich is ON and OFF"
            n693 = local read "Cal @ Delta (nm)"() -> (w1127:dbl)
            n694 = local write "Stage moving"(FALSE ("Stage moving")) -> ()
            n695 = call <vilib>:"Beep.vi"() -> ()  [unwired: 12 in]
            n696 = property on="Trap delta (nm)" class="DigNum (strict)"("Val(Sgnl)"=w1127) -> ()  [unwired: 2 in, 2 out]
            n697 = disable-structure shown="Disabled" {
              frame Disabled {
                n698 = property on="Inject Pump 1" class="Bool (strict)"("Val(Sgnl)"=TRUE ("Inject Pump 2")) -> ()  [unwired: 2 in, 2 out]
              }
              frame Enabled {
              }
            }
            n699 = local read "Shutter 2 (A)"() -> (w1126:bool)
            n700 = case shown="False" w1126 {
              frame False {
                n701 = property on="Shutter 2 (A)" class="Bool (strict)"("Val(Sgnl)"=TRUE ("Value (Signaling)")) -> ()  [unwired: 2 in, 2 out]
              }
              frame True {
              }
            }
            n702 = property on="Inject Sample" class="Bool (strict)"("Val(Sgnl)"=FALSE ("Value (Signaling)")) -> ()  [unwired: 2 in, 2 out]
          }
        }
      }
      event "Got ADig bead": Value Change {
        n703 = event-data() -> ()  [unwired: 1 in, 5 out]
        n704 = flat-sequence {
          tunnel: w1133 -> [w1137]
          tunnel: w1132 -> [w1136]
          frame #0 {
            n705 = local read "Saved stage positions"() -> (w1139:dbl[][])
            n706 = property on="Inject Pump 1" class="Bool (strict)"("Val(Sgnl)"=FALSE ("Inject Pump 2")) -> ()  [unwired: 2 in, 2 out]
            n707 = case shown="True" "Flow on\ncap 1?" {
              frame False {
              }
              frame True {
                n708 = property on="Inject Sample" class="Bool (strict)"("Val(Sgnl)"=TRUE ("Value (Signaling)")) -> ()  [unwired: 2 in, 2 out]
              }
            }
            n709 = local write "Stage moving"(TRUE ("Stage moving")) -> ()
            n710 = call "move to saved stage position.vi"("error in"=w1136, "Stage VISA resource name in"=w1137, "Position"=1, "Saved Stage Positions"=w1139) -> ()  [unwired: 2 out]
          }
          frame #1 {
            n711 = local read "Shutter 1 (B)"() -> (w1143:bool)
            n712 = disable-structure shown="Disabled" {
              frame Disabled {
                n713 = property on="Inject Pump 2" class="Bool (strict)"("Val(Sgnl)"=TRUE ("Inject Pump 2")) -> ()  [unwired: 2 in, 2 out]
              }
              frame Enabled {
              }
            }
            n714 = local write "Stage moving"(FALSE ("Stage moving")) -> ()
            n715 = case shown="False" w1143 {
              frame False {
                n716 = property on="Shutter 1 (B)" class="Bool (strict)"("Val(Sgnl)"=TRUE ("Value (Signaling)")) -> ()  [unwired: 2 in, 2 out]
              }
              frame True {
              }
            }
            n717 = property on="Inject Sample" class="Bool (strict)"("Val(Sgnl)"=FALSE ("Value (Signaling)")) -> ()  [unwired: 2 in, 2 out]
            n718 = call <vilib>:"Beep.vi"() -> ()  [unwired: 12 in]
          }
        }
        n719 = local write "Got ADig bead"(FALSE ("Got ADig bead")) -> ()
      }
      event "Set Position 1", "Set Position 2", "Set Position 3", "Set Position 4", "Set Position 5": Value Change {
        n720 = event-data() -> ()  [unwired: 1 in, 5 out]
        n721 = Build Array("Set Position 1", "Set Position 2", "Set Position 3", "Set Position 4", "Set Position 5") -> (w1162:bool[])
        n722 = Boolean Array To Number(Boolean array=w1162) -> (number=w1161:u32)
        n723 = call "Read Stage Position.vi"("error in"=w1149, "VISA resource name in"=w1150) -> ("Current Position"=w1147:cluster{dbl, dbl, dbl}, "error out"=→"Stage error":errorcluster)  [unwired: 1 in, 1 out]
        n724 = Logarithm Base 2(1:w1161) -> (0:w1155:dbl)
        n725 = Cluster To Array(cluster=w1147) -> (array=w1157:dbl[])
        n726 = Increment(x=w1155) -> (x+1=w1158:dbl)
        n727 = Build Array (concatenate)(w1158, w1157) -> (w1156:dbl[])
        n728 = Replace Array Subset(array="Saved stage positions", new element=w1156, index (row)=w1155) -> (w1159:dbl[][])  [unwired: 1 in]
        n729 = local write "Saved stage positions"(w1159) -> ()
      }
      event "Move to Position 2", "Move to Position 4", "Move to Position 3", "Move to Position 5", "Move to Position 1": Value Change {
        n730 = event-data() -> ()  [unwired: 1 in, 5 out]
        n731 = Build Array("Move to Position 1", "Move to Position 2", "Move to Position 3", "Move to Position 4", "Move to Position 5") -> (w1172:bool[])
        n732 = Boolean Array To Number(Boolean array=w1172) -> (number=w1171:u32)
        n733 = Logarithm Base 2(1:w1171) -> (0:w1170:dbl)
        n734 = flat-sequence {
          tunnel: w1170 -> [w1177]
          tunnel: w1169 -> [w1176]
          tunnel: w1168 -> [w1175]
          frame #0 {
            n735 = local read "Saved stage positions"() -> (w1178:dbl[][])
            n736 = Increment(x=w1177) -> (x+1=w1174:dbl)
            n737 = call "move to saved stage position.vi"("error in"=w1175, "Stage VISA resource name in"=w1176, "Position"=w1174, "Saved Stage Positions"=w1178) -> ()  [unwired: 2 out]
            "Stage moving" <- TRUE ("Stage moving")
          }
          frame #1 {
            n738 = call <vilib>:"Beep.vi"() -> ()  [unwired: 12 in]
            n739 = local write "Stage moving"(FALSE ("Stage moving")) -> ()
          }
        }
      }
      event "Set Current\nPos to (0,0,0)": Value Change {
        w1182 = ";" ("string")
        # "DH is \"Define Home\" -KW"
        n740 = event-data() -> ()  [unwired: 1 in, 5 out]
        n741 = local write "Set Current\nPos to (0,0,0)"(FALSE ("Set Current\nPos to (0,0,0)")) -> ()
        n742 = call-poly "VISA Configure Serial Port"("VISA resource name"=w1192, "baud rate (9600)"=u32 19200, "error in (no error)"=w1191) -> ("VISA resource name out"=w1186:refnum<visa-resource-name>, "error out"=w1185:errorcluster)  [unwired: 11 in]
        n743 = Concatenate Strings("1DH" ("string"), w1182, "2DH" ("string"), w1182, "3DH" ("string"), "\r") -> (w1184:string)
        n744 = VISA Write(VISA resource name=w1186, write buffer=w1184, error in (no error)=w1185) -> (error out=w1183:errorcluster)  [unwired: 2 out]
        n745 = local write "Stage error"(w1183) -> ()
      }
      event "Dip": Value Change {
        n746 = event-data() -> ()  [unwired: 1 in, 5 out]
        n747 = local write "Dip"(FALSE ("Dip")) -> ()
        n748 = flat-sequence {
          tunnel: w1202 -> [w1204]
          tunnel: w1201 -> [w1203]
          tunnel: [w1205] -> w1199
          tunnel: [w1204] -> w1197
          tunnel: [w1203] -> w1195
          tunnel: [w1213] -> w1200
          tunnel: w1199 -> [w1213]
          tunnel: [w1212] -> w1198
          tunnel: w1197 -> [w1212]
          tunnel: [w1211] -> w1196
          tunnel: w1195 -> [w1211]
          tunnel: w1200 -> [w1232]
          tunnel: w1198 -> [w1231]
          tunnel: w1196 -> [w1230]
          frame #0 {
            n749 = local read "Saved stage positions"() -> (w1205:dbl[][])
            n750 = local write "Stage moving"(TRUE) -> ()
            n751 = call "move to saved stage position.vi"("error in"=w1203, "Stage VISA resource name in"=w1204, "Position"="Dip position", "Saved Stage Positions"=w1205) -> ()  [unwired: 2 out]
          }
          frame #1 {
            n752 = node-c288() -> (w1210:T11)  [unwired: 4 in]
            n753 = timed-loop {
              timing: w1210 -> [_]
              timing-out: [_] -> w1209
              i -> [w1223]
              stop <- w1214 stop-if-true
              n754 = node-c288() -> ()  [unwired: 1 in, 1 out]
              n755 = Greater Or Equal?(x=w1223, y="Dip duration") -> (x >= y?=w1219:bool)
              n756 = local read "Dump beads"() -> (w1216:bool)
              n757 = Or(x=w1219, y="Cancel dwell") -> (x .or. y?=w1217:bool)
              n758 = Not(x="Pause dwell") -> (.not. x?=w1220:bool)
              n759 = node-c288() -> ()  [unwired: 1 in, 1 out]
              n760 = And(x=w1220, y=w1217) -> (x .and. y?=w1215:bool)
              n761 = Or(x=w1215, y=w1216) -> (x .or. y?=w1214:bool)
              "Dip time" <- w1223
            }
            n762 = local write "Stage moving"(FALSE ("Stage moving")) -> ()
            n763 = node-c288(w1209) -> ()  [unwired: 1 out]
          }
          frame #2 {
            n764 = local write "Cancel dwell"(FALSE ("Cancel dwell")) -> ()
            n765 = call "move to saved stage position.vi"("error in"=w1230, "Stage VISA resource name in"=w1231, "Position"="Return position", "Saved Stage Positions"=w1232) -> ()  [unwired: 2 out]
          }
          frame #3 {
            n766 = local write "Stage moving"(FALSE ("Stage moving")) -> ()
          }
        }
      }
      event "Force FB script": Value Change {
        n767 = event-data() -> ()  [unwired: 1 in, 5 out]
        n768 = flat-sequence {
          frame #0 {
            n769 = disable-structure shown="Disabled" {
              frame Disabled {
                n770 = local read "# Samples/channel"() -> (w1236:i32)
                n771 = local write "# Samples/channel (in)"(w1236) -> ()
              }
              frame Enabled {
              }
            }
            n772 = local write "Force FB script"(FALSE ("Force FB script")) -> ()
            n773 = property on="Trap delta (nm)" class="DigNum (strict)"("Val(Sgnl)"="Start trap delta (nm)") -> ()  [unwired: 2 in, 2 out]
          }
          frame #1 {
            n774 = Wait (ms)(milliseconds to wait=u32 500) -> ()  [unwired: 1 out]
          }
          frame #2 {
            n775 = property on="Set reading to\nsetpoint" class="Bool (strict)"("Val(Sgnl)"=TRUE ("Value (Signaling)")) -> ()  [unwired: 2 in, 2 out]
          }
          frame #3 {
            n776 = Wait (ms)(milliseconds to wait=u32 300) -> ()  [unwired: 1 out]
          }
          frame #4 {
            n777 = local write "Force Feedback"(TRUE ("Force Feedback")) -> ()
            n778 = property on="Tabs" class="TabCtl (strict)"("Val(Sgnl)"=T4."Force Feedback" ("Value (Signaling)")) -> ()  [unwired: 2 in, 2 out]
          }
          frame #5 {
            n779 = property on="Save Data" class="Bool (strict)"("Val(Sgnl)"=TRUE ("Value (Signaling)")) -> ()  [unwired: 2 in, 2 out]
          }
          frame #6 {
            n780 = Multiply(x="Wait before dip (s)", y=1000) -> (x*y=w1243:dbl)
            n781 = Wait (ms)(milliseconds to wait=w1243) -> ()  [unwired: 1 out]
          }
          frame #7 {
            n782 = case shown="True" "Start dipping after?" {
              selector: "Start dipping after?" -> [_ w1248]
              frame False {
              }
              frame True {
                n783 = property on="Dip" class="Bool (strict)"("Val(Sgnl)"=w1248) -> ()  [unwired: 2 in, 2 out]
              }
            }
            n784 = property on="Remove offsets" class="Bool (strict)"("Val(Sgnl)"=TRUE ("Value (Signaling)")) -> ()  [unwired: 2 in, 2 out]
          }
        }
      }
      event "Move 0": Value Change {
        n785 = event-data() -> ()  [unwired: 1 in, 5 out]
        n786 = local write "Move 0"(FALSE) -> ()
        n787 = call "HalfWavePlate.vi"("Degrees"="\"Degrees\" 0", "Motor"=0) -> ()  [unwired: 1 in]
      }
      event "Move 1": Value Change {
        n788 = event-data() -> ()  [unwired: 1 in, 5 out]
        n789 = local write "Move 1"(FALSE) -> ()
        n790 = call "HalfWavePlate.vi"("Degrees"="\"Degrees\" 1", "Motor"=1) -> ()  [unwired: 1 in]
      }
      event "Stop": Value Change {
        n791 = event-data() -> ()  [unwired: 1 in, 5 out]
        n792 = local read "Stop"() -> (w1255:bool)
      }
    }
    n793 = node-c288() -> ()  [unwired: 1 in, 1 out]
  }
  n794 = node-c288(2 ("Processor")) -> (w71:T11)  [unwired: 3 in]
  n795 = node-c288(2 ("Processor")) -> (w23:T11)  [unwired: 3 in]
  n796 = timed-loop {
    timing: w71 -> [_]
    timing-out: [_] -> w70
    stop <- w1258 stop-if-true
    n797 = node-c288() -> ()  [unwired: 1 in, 1 out]
    n798 = case shown="\"Current Saved Data\"" "Tab Control" {
      frame "Control" {
        n799 = case shown="True" "Start" {
          frame False {
          }
          frame True {
            w1271 = T19 3 items=["no dialog", "OK message", "continue or stop message", "OK message + warnings", "continue/stop + warnings"] ("type of dialog (OK msg:1)")
            n800 = call "InitializeAcquireFF.vi"("DAQ Rate"="DAQ Rate", "Averaging Number"="Averaging Number", "Sampling Rate"="Sampling Rate") -> ("error out"=w1265:errorcluster, "task out"=w1264:refnum<k21>, "Final Sampling Rate"=→"Final Sampling Rate":dbl)  [unwired: 4 in, 2 out]
            n801 = while {
              tunnel: [w1283] -> w1270
              tunnel: [w1282] -> w1263
              tunnel: "Averaging Number" -> [w1281]
              tunnel: w1265 -> [w1280]
              tunnel: w1264 -> [w1278]
              stop <- w1279 continue-if-true
              n802 = call "Acquire2_QPD.vi"("task/channels in"=w1278, "Save Data?"=FALSE ("Take Data?"), "Averaging Number"=w1281, "error in"=w1280) -> ("PSD 1"=→"PSD 1":cluster{dbl[], dbl[]}, "PSD 1 Sum"=→"PSD 1 Sum":dbl, "PSD 2"=→"PSD 2":cluster{dbl[], dbl[]}, "PSD 2 Sum"=→"PSD 2 Sum":dbl, "task out"=w1283:refnum<k21>, "error out"=w1282:errorcluster)  [unwired: 14 in, 4 out]
              n803 = local read "Start"() -> (w1279:bool)
            }
            n804 = call <vilib>:"DAQmx Clear Task.vi"("task in"=w1270, "error in"=w1263) -> ("error out"=w1272:errorcluster)  [unwired: 13 in]
            n805 = call <vilib>:"Simple Error Handler.vi"("type of dialog (OK msg:1)"=w1271, "error in (no error)"=w1272) -> ()  [unwired: 3 in, 5 out]
          }
        }
      }
      frame "Current Saved Data" {
      }
      frame "Data Acquisition" {
      }
      frame "Raw QPD Data" {
      }
    }
    n806 = local read "Stop"() -> (w1258:bool)
    n807 = node-c288() -> ()  [unwired: 1 in, 1 out]
  }
  n808 = call-poly <vilib>:"DAQmx Create Virtual Channel.vi"("lines"=w88) -> ("task out"=w87:refnum<k21>)  [unwired: 13 in, 1 out]
  n809 = call-poly <vilib>:"DAQmx Create Virtual Channel.vi"("lines"=w91) -> ("task out"=w90:refnum<k21>)  [unwired: 13 in, 1 out]
  n810 = timed-loop {
    timing: w23 -> [_]
    timing-out: [_] -> w22
    stop <- w1284 stop-if-true
    n811 = node-c288() -> ()  [unwired: 1 in, 1 out]
    n812 = event shown="[0] \"Pause Mouse/Mirror Connection\": Value Change" {
      selector: _ -> [_ _]
      dyn-events: _ -> [_ _]
      timeout: _ -> [_ _]
      tunnel: [w1377 _] -> w1285
      tunnel: [_ w1378] -> w1284
      event "Pause Mouse/Mirror Connection": Value Change {
        n813 = event-data() -> ("NewVal"=w1377:bool)  [unwired: 1 in]
      }
      event "Stop": Value Change {
        n814 = event-data() -> ("NewVal"=w1378:bool)  [unwired: 1 in]
      }
    }
    n815 = case shown="True" w1285 {
      frame False {
      }
      frame True {
        n816 = call "InitializeMouseControl.vi"() -> ("error out 2"=w1294:errorcluster, "task out"=w1295:refnum<k21>, "error out"=w1297:errorcluster, "device ID"=w1296:refnum<k1>)  [unwired: 8 in]
        n817 = while {
          tunnel: w1297 -> [w1309]
          tunnel: w1296 -> [w1308]
          tunnel: w1295 -> [w1307]
          tunnel: w1294 -> [w1306]
          tunnel: [w1305] -> w1292
          tunnel: [w1304] -> w1291
          tunnel: [w1303] -> w1288
          tunnel: [w1302] -> w1289
          stop <- w1301 stop-if-true
          n818 = case shown="True" "Use Mouse to Move Trap?" {
            tunnel: w1308 -> [w1316 w1339]
            tunnel: w1309 -> [w1315 w1338]
            tunnel: w1307 -> [w1314 w1337]
            tunnel: w1306 -> [w1313 w1336]
            tunnel: [w1316 w1335] -> w1303
            tunnel: [w1315 w1334] -> w1302
            tunnel: [w1314 w1333] -> w1305
            tunnel: [w1313 w1332] -> w1304
            frame False {
              (unwired) FALSE ("button 1")
            }
            frame True {
              w1327 = 0.0 ("y")
              w1329 = 10
              n819 = local read "Deflection"() -> (w1340:T5)
              n820 = call-poly <vilib>:"Acquire Input Data.vi"("device ID"=w1339, "error in (no error)"=w1338) -> ("device ID"=w1335:refnum<k1>, "button info"=w1353:T20, "error out"=w1334:errorcluster)  [unwired: 14 in, 1 out]
              n821 = Unbundle By Name(w1340) -> ("Horizontal"=w1342:i32, "Vertical"=w1341:i32)
              n822 = local read "Saved voltage"() -> (w1318:cluster{dbl, dbl})
              n823 = Divide(x=w1342, y=30) -> (x/y=w1345:dbl)
              n824 = Divide(x=w1341, y=-20) -> (x/y=w1346:dbl)
              n825 = Unbundle By Name(w1353) -> ("button 1"=w1331:bool, "button 2"=w1347:bool)
              n826 = Bundle(w1345, w1346) -> (w1323:cluster{dbl, dbl})  [unwired: 1 in]
              n827 = local write "Reference Voltage"(w1323) -> ()
              n828 = Add(x=w1323, y=w1318) -> (x+y=w1351:cluster{dbl, dbl})
              n829 = case shown="True" w1331 {
                frame False {
                  n830 = stacked-sequence {
                    frame #0 {
                      n831 = local write "CoordinatesMousePressed"(T5 {"Horizontal"=0, "Vertical"=0} ("Coords when pressed")) -> ()
                      n832 = local write "Deflection"(T5 {"Horizontal"=0, "Vertical"=0} ("deflaction")) -> ()
                    }
                  }
                }
                frame True {
                  n833 = local read "CoordinatesMousePressed"() -> (w1376:T5)
                  n834 = local read "Real Coordinates"() -> (w1375:cluster{"Horizontal":i32, "Vertical":i32})
                  n835 = Subtract(x=w1375, y=w1376) -> (x-y=w1374:T5)
                  n836 = local write "Deflection"(w1374) -> ()
                }
              }
              n837 = Unbundle(w1351) -> (w1328:dbl, w1319:dbl)
              n838 = case shown="True" w1347 {
                frame False {
                }
                frame True {
                  n839 = local read "Reference Voltage"() -> (w1357:cluster{dbl, dbl})
                  n840 = local read "Saved voltage"() -> (w1355:cluster{dbl, dbl})
                  n841 = Add(x=w1357, y=w1355) -> (x+y=→"Saved voltage":cluster{dbl, dbl})
                  n842 = local read "Real Coordinates"() -> (w1356:cluster{"Horizontal":i32, "Vertical":i32})
                  n843 = local write "CoordinatesMousePressed"(w1356) -> ()
                }
              }
              n844 = Less?(x=w1328, y=w1329) -> (x < y?=w1326:bool)
              n845 = Greater?(x=w1328, y=w1327) -> (0:w1325:bool)
              n846 = Greater?(x=w1319, y=w1327) -> (0:w1321:bool)
              n847 = Less?(x=w1319, y=w1329) -> (x < y?=w1322:bool)
              n848 = And(x=w1321, y=w1322) -> (x .and. y?=w1320:bool)
              n849 = And(x=w1326, y=w1325) -> (x .and. y?=w1324:bool)
              n850 = case shown="False" w1320 {
                tunnel: [w1367 w1371] -> w1330
                tunnel: w1319 -> [w1365 w1371]
                frame False {
                  n851 = Greater?(x=w1365, y=10.0) -> (0:w1368:bool)
                  n852 = case shown="True" w1368 {
                    tunnel: [0.0 10.0] -> w1367
                    frame False {
                    }
                    frame True {
                    }
                  }
                }
                frame True {
                }
              }
              n853 = case shown="False" w1324 {
                tunnel: w1328 -> [w1359 w1364]
                tunnel: [w1360 w1364] -> w1352
                frame False {
                  n854 = Greater?(x=w1359, y=10.0) -> (0:w1361:bool)
                  n855 = case shown="True" w1361 {
                    tunnel: [0.0 10.0] -> w1360
                    frame False {
                    }
                    frame True {
                    }
                  }
                }
                frame True {
                }
              }
              n856 = Bundle(w1352, w1330) -> (w1317:cluster{dbl, dbl})  [unwired: 1 in]
              n857 = Cluster To Array(cluster=w1317) -> (array=w1348:dbl[])
              n858 = call-poly <vilib>:"DAQmx Write.vi"("task/channels in"=w1337, "data"=w1348, "error in"=w1336) -> ("task out"=w1350:refnum<k21>, "error out"=w1349:errorcluster)  [unwired: 10 in, 1 out]
              n859 = call <vilib>:"DAQmx Is Task Done.vi"("task/channels in"=w1350, "error in"=w1349) -> ("task out"=w1333:refnum<k21>, "error out"=w1332:errorcluster)  [unwired: 11 in, 1 out]
            }
          }
          n860 = event shown="[0] \"Pane\": Mouse Move" {
            selector: _ -> [_ _ _]
            dyn-events: _ -> [_ _ _]
            timeout: _ -> [_ _ _]
            event Mouse Move {
              n861 = event-data() -> ("Coords"=w1311:T5)  [unwired: 1 in]
              n862 = local write "Real Coordinates"(w1311) -> ()
            }
            event Mouse Down {
              n863 = event-data() -> ("Coords"=w1312:T5)  [unwired: 1 in]
              n864 = local write "CoordinatesMousePressed"(w1312) -> ()
            }
            event "Pause Mouse/Mirror Connection": Value Change {
              n865 = event-data() -> ()  [unwired: 1 in, 3 out]
            }
          }
          n866 = local read "Stop"() -> (w1298:bool)
          n867 = Not(x="Pause Mouse/Mirror Connection") -> (.not. x?=w1299:bool)
          n868 = Or(x=w1299, y=w1298) -> (x .or. y?=w1301:bool)
        }
        n869 = call <vilib>:"DAQmx Clear Task.vi"("task in"=w1292, "error in"=w1291) -> ("error out"=w1293:errorcluster)  [unwired: 13 in]
        n870 = call <vilib>:"Simple Error Handler.vi"("error in (no error)"=w1293) -> ()  [unwired: 4 in, 5 out]
        n871 = call-poly <vilib>:"Close Input Device.vi"("error in (no error)"=w1289, "device ID"=w1288) -> ("error out"=w1290:errorcluster)  [unwired: 8 in]
        n872 = call <vilib>:"Simple Error Handler.vi"("error in (no error)"=w1290) -> ()  [unwired: 4 in, 5 out]
      }
    }
    n873 = node-c288() -> ()  [unwired: 1 in, 1 out]
  }
  n874 = node-c288(i64 100 ("Period")) -> (w85:T11)  [unwired: 3 in]
  n875 = timed-loop {
    tunnel: w87 -> [w1381]
    tunnel: [w1380] -> w86
    tunnel: w90 -> [w1383]
    tunnel: [w1382] -> w89
    timing: w85 -> [_]
    timing-out: [_] -> w84
    stop <- w1379 stop-if-true
    n876 = node-c288() -> ()  [unwired: 1 in, 1 out]
    n877 = event shown="[1] \"Shutter 2 (A)\": Value Change" {
      selector: _ -> [_ _ _]
      dyn-events: _ -> [_ _ _]
      timeout: _ -> [_ _ _]
      tunnel: w1383 -> [w1387 _ _]
      tunnel: [w1386 _ _] -> w1382
      tunnel: w1381 -> [_ w1407 _]
      tunnel: [_ w1405 _] -> w1380
      tunnel: [_ _ w1424] -> w1379
      event "Shutter 1 (B)": Value Change {
        n878 = event-data() -> ()  [unwired: 1 in, 1 out]
        n879 = flat-sequence {
          tunnel: [w1393] -> w1390
          tunnel: w1387 -> [w1392]
          tunnel: [w1397] -> w1389
          tunnel: [w1400] -> w1388
          tunnel: w1390 -> [w1395]
          tunnel: w1389 -> [w1404]
          tunnel: w1388 -> [w1402]
          tunnel: [w1401] -> w1386
          frame #0 {
            n880 = call-poly <vilib>:"DAQmx Write.vi"("task/channels in"=w1392, "data"=FALSE) -> ("task out"=w1393:refnum<k21>)  [unwired: 11 in, 2 out]
            n881 = Wait (ms)(milliseconds to wait=100) -> ()  [unwired: 1 out]
          }
          frame #1 {
            n882 = Or(x="Shutter 1 (B)", y=TRUE) -> (x .or. y?=w1397:bool)
            n883 = call-poly <vilib>:"DAQmx Write.vi"("task/channels in"=w1395, "data"=w1397) -> ("task out"=w1400:refnum<k21>)  [unwired: 11 in, 2 out]
            n884 = Wait (ms)(milliseconds to wait=100) -> ()  [unwired: 1 out]
          }
          frame #2 {
            n885 = Not(x=w1404) -> (.not. x?=w1403:bool)
            n886 = call-poly <vilib>:"DAQmx Write.vi"("task/channels in"=w1402, "data"=w1403) -> ("task out"=w1401:refnum<k21>)  [unwired: 11 in, 2 out]
          }
        }
      }
      event "Shutter 2 (A)": Value Change {
        n887 = event-data() -> ()  [unwired: 1 in, 1 out]
        n888 = flat-sequence {
          tunnel: w1407 -> [w1412]
          tunnel: [w1411] -> w1406
          tunnel: [w1416] -> w1409
          tunnel: [w1419] -> w1408
          tunnel: w1406 -> [w1414]
          tunnel: w1409 -> [w1423]
          tunnel: w1408 -> [w1421]
          tunnel: [w1420] -> w1405
          frame #0 {
            n889 = call-poly <vilib>:"DAQmx Write.vi"("task/channels in"=w1412, "data"=FALSE) -> ("task out"=w1411:refnum<k21>)  [unwired: 11 in, 2 out]
            n890 = Wait (ms)(milliseconds to wait=100) -> ()  [unwired: 1 out]
          }
          frame #1 {
            n891 = Or(x="Shutter 2 (A)", y=TRUE) -> (x .or. y?=w1416:bool)
            n892 = call-poly <vilib>:"DAQmx Write.vi"("task/channels in"=w1414, "data"=w1416) -> ("task out"=w1419:refnum<k21>)  [unwired: 11 in, 2 out]
            n893 = Wait (ms)(milliseconds to wait=100) -> ()  [unwired: 1 out]
          }
          frame #2 {
            n894 = Not(x=w1423) -> (.not. x?=w1422:bool)
            n895 = call-poly <vilib>:"DAQmx Write.vi"("task/channels in"=w1421, "data"=w1422) -> ("task out"=w1420:refnum<k21>)  [unwired: 11 in, 2 out]
          }
        }
      }
      event "Stop": Value Change {
        n896 = event-data() -> ("NewVal"=w1424:bool)  [unwired: 1 in, 5 out]
      }
    }
    n897 = node-c288() -> ()  [unwired: 1 in, 1 out]
  }
  n898 = node-c288(w84) -> ()  [unwired: 1 out]
  n899 = node-c288(w70) -> ()  [unwired: 1 out]
  n900 = call <vilib>:"DAQmx Clear Task.vi"("task in"=w86) -> ()  [unwired: 14 in, 1 out]
  n901 = call <vilib>:"DAQmx Clear Task.vi"("task in"=w89) -> ()  [unwired: 14 in, 1 out]
  n902 = node-c288(w22) -> ()  [unwired: 1 out]
  n903 = node-c288(w18) -> ()  [unwired: 1 out]
  n904 = local write "Tether"(FALSE ("Tether")) -> ()
  n905 = local read "Path"() -> (w77:path)
  n906 = node-c288(i64 1 ("Period"), 2 ("Processor")) -> (w83:T11)  [unwired: 2 in]
  n907 = VISA Close(VISA resource name=w15) -> (error out=w95:errorcluster)  [unwired: 1 in]
  n908 = timed-loop {
    timing: w83 -> [_]
    timing-out: [_] -> w82
    tunnel: w77 -> [w1426]
    stop <- w1425 stop-if-true
    n909 = node-c288() -> ()  [unwired: 1 in, 1 out]
    n910 = event shown="[5] \"Fish\": Value Change" {
      selector: _ -> [_ _ _ _ _ _ _ _ _]
      dyn-events: _ -> [_ _ _ _ _ _ _ _ _]
      timeout: _ -> [_ _ _ _ _ _ _ _ _]
      tunnel: w1426 -> [_ w1430 _ _ _ _ _ _ _]
      tunnel: [_ _ w1450 _ _ _ _ _ _] -> w1425
      event Timeout {
        n911 = event-data() -> ()  [unwired: 1 in, 2 out]
      }
      event "Read Cal": Value Change {
        n912 = event-data() -> ()  [unwired: 1 in, 6 out]
        n913 = Path To String(path=w1430) -> (string=w1429:string)
        n914 = Format Date/Time String(time format string (%c)="%y%m%d") -> (date/time string=w1431:string)  [unwired: 2 in]
        n915 = Concatenate Strings(w1429, "\\" ("string"), w1431, "\\" ("string"), "current.cal") -> (w1449:string)
        n916 = String To Path(string=w1449) -> (path=w1448:path)
        n917 = Open/Create/Replace File(file path (use dialog)=w1448, operation (0:open)=T16."open", access (0:read/write)=enum16{"read/write", "read-only", "write-only"}."read-only") -> (refnum out=w1444:refnum<file>, error out=w1445:errorcluster)  [unwired: 3 in, 1 out]
        n918 = Deny Access(4:w1445, 7:w1444) -> (0:w1443:errorcluster, 3:w1442:refnum<file>)  [unwired: 1 in]
        n919 = Read from Binary File(5:0.0, 8:w1443, 9:T17."big-endian, network order" ("byte order (0:big-endian, network order)"), 10:12 ("count"), 11:w1442) -> (0:w1438:errorcluster, 2:w1436:dbl[], 3:w1439:refnum<file>)  [unwired: 1 in, 1 out]
        n920 = Array To Cluster(array=w1436) -> (cluster=→"Cal values":T21)
        n921 = Close File(refnum=w1439, error in=w1438) -> ()  [unwired: 2 out]
        n922 = local write "Read Cal"(FALSE ("Read Cal")) -> ()
      }
      event "Stop": Value Change {
        n923 = event-data() -> ("NewVal"=w1450:bool)  [unwired: 1 in, 5 out]
      }
      event "Trap position (V)": Value Change {
        # "Need to rotate so X and Y don't get mixed up."
        n924 = event-data() -> ()  [unwired: 1 in, 6 out]
        n925 = local read "Mirror task"() -> (w1451:refnum<k21>)
        n926 = Cluster To Array(cluster="Trap position (V)") -> (array=w1454:dbl[])
        n927 = Rotate 1D Array(1:w1454, 2:1 ("n")) -> (0:w1452:dbl[])
        n928 = call-poly <vilib>:"DAQmx Write.vi"("task/channels in"=w1451, "data"=w1452) -> ("task out"=w1457:refnum<k21>, "error out"=w1456:errorcluster)  [unwired: 11 in, 1 out]
        n929 = call <vilib>:"DAQmx Stop Task.vi"("task/channels in"=w1457, "error in"=w1456) -> ("error out"=w1455:errorcluster)  [unwired: 12 in, 1 out]
        n930 = call <vilib>:"Simple Error Handler.vi"("error in (no error)"=w1455) -> ()  [unwired: 4 in, 5 out]
      }
      event "Trap delta (nm)": Value Change {
        n931 = event-data() -> ()  [unwired: 1 in, 6 out]
        n932 = local read "Pulling direction"() -> (w1459:bool)
        n933 = local read "Conv Y (nm/V)"() -> (w1460:dbl)
        n934 = local read "Conv X (nm/V)"() -> (w1461:dbl)
        n935 = Select(t=w1460, s=w1459, f=w1461) -> (s? t:f=w1462:dbl)
        n936 = local read "Fixed Y"() -> (w1468:dbl)
        n937 = Divide(x="Trap delta (nm)", y=w1462) -> (x/y=w1463:dbl)
        n938 = local read "Fixed X"() -> (w1467:dbl)
        n939 = Select(t=w1468, s=w1459, f=w1467) -> (s? t:f=w1466:dbl)
        n940 = Add(x=w1463, y=w1466) -> (x+y=w1464:dbl)
        n941 = case shown="False" w1459 {
          tunnel: w1464 -> [w1469 w1470]
          frame False {
            n942 = property on="X" class="DigNum (strict)"("Val(Sgnl)"=w1469) -> ()  [unwired: 2 in, 2 out]
          }
          frame True {
            n943 = property on="Y" class="DigNum (strict)"("Val(Sgnl)"=w1470) -> ()  [unwired: 2 in, 2 out]
          }
        }
      }
      event "Fish": Value Change {
        n944 = event-data() -> ()  [unwired: 1 in, 6 out]
        n945 = local read "Fish"() -> (w1471:bool)
        n946 = case shown="True" w1471 {
          frame False {
          }
          frame True {
            w1480 = 0.0 ("minimum value")
            w1481 = 10.0 ("maximum value")
            # "Grab offset in pulling\ndirection and add to \ndelta values"
            n947 = call-poly <vilib>:"DAQmx Create Virtual Channel.vi"("maximum value"=w1481, "minimum value"=w1480, "physical channels"=tag "Dev1/ao0") -> ("task out"=w1485:refnum<k21>, "error out"=w1484:errorcluster)  [unwired: 11 in]
            n948 = call-poly <vilib>:"DAQmx Create Virtual Channel.vi"("task in"=w1485, "maximum value"=w1481, "minimum value"=w1480, "physical channels"=tag "Dev1/ao1", "error in"=w1484) -> ("task out"=w1479:refnum<k21>, "error out"=w1478:errorcluster)  [unwired: 9 in]
            n949 = node-c288(i64 1 ("Period")) -> (w1487:T11)  [unwired: 3 in]
            n950 = timed-loop {
              timing: w1487 -> [_]
              timing-out: [_] -> w1486
              tunnel: w1479 -> [w1547]
              tunnel: w1478 -> [w1546]
              tunnel: [w1545] -> w1474
              tunnel: [w1544] -> w1473
              tunnel: [w1504] -> w1476
              tunnel: [w1505] -> w1472
              i -> [w1530]
              stop <- w1505 stop-if-true
              # "Send offset in direction\nof not-pulling to DAQ"
              n951 = node-c288() -> ()  [unwired: 1 in, 1 out]
              n952 = local read "Pulling direction"() -> (w1509:bool)
              n953 = local read "Conv Y (nm/V)"() -> (w1511:dbl)
              n954 = local read "Conv X (nm/V)"() -> (w1510:dbl)
              n955 = local read "Fixed X"() -> (w1518:dbl)
              n956 = local read "Fixed Y"() -> (w1517:dbl)
              n957 = Select(t=w1517, s=w1509, f=w1518) -> (s? t:f=w1519:dbl)
              n958 = Select(t=w1518, s=w1509, f=w1517) -> (s? t:f=w1516:dbl)
              n959 = Select(t=w1511, s=w1509, f=w1510) -> (s? t:f=w1506:dbl)
              n960 = Divide(x="Max fish\ndelta (nm)", y=w1506) -> (x/y=w1508:dbl)
              n961 = Divide(x="Min fish\ndelta (nm)", y=w1506) -> (x/y=w1507:dbl)
              n962 = Add(x=w1519, y=w1508) -> (x+y=w1521:dbl)
              n963 = Subtract(x=w1508, y=w1507) -> (x-y=w1523:dbl)
              n964 = Divide(x=w1523, y="Fish Speed (ms)") -> (x/y=w1524:dbl)
              n965 = flat-sequence {
                tunnel: w1509 -> [w1567]
                tunnel: w1516 -> [w1566]
                tunnel: w1547 -> [w1565]
                tunnel: w1546 -> [w1564]
                tunnel: w1524 -> [w1563]
                tunnel: w1521 -> [w1562]
                tunnel: "Fish Speed (ms)" -> [w1557]
                tunnel: [w1561] -> w1543
                tunnel: [w1560] -> w1542
                tunnel: [w1559] -> w1541
                tunnel: [w1558] -> w1540
                tunnel: [w1551] -> w1529
                tunnel: [w1550] -> w1515
                tunnel: [w1549] -> w1512
                tunnel: [w1548] -> w1502
                tunnel: [w1620] -> w1539
                tunnel: w1543 -> [w1620]
                tunnel: [w1619] -> w1538
                tunnel: w1542 -> [w1619]
                tunnel: [w1618] -> w1537
                tunnel: w1541 -> [w1618]
                tunnel: [w1617] -> w1536
                tunnel: w1540 -> [w1617]
                tunnel: w1529 -> [w1616]
                tunnel: [w1616] -> w1528
                tunnel: w1515 -> [w1615]
                tunnel: [w1614] -> w1513
                tunnel: w1512 -> [w1614]
                tunnel: [w1613] -> w1503
                tunnel: w1502 -> [w1613]
                tunnel: w1539 -> [w1632]
                tunnel: w1538 -> [w1631]
                tunnel: w1537 -> [w1630]
                tunnel: w1536 -> [w1629]
                tunnel: w1526 -> [w1628]
                tunnel: [w1627] -> w1545
                tunnel: [w1626] -> w1544
                tunnel: w1528 -> [w1625]
                tunnel: [w1624] -> w1514
                tunnel: w1513 -> [w1623]
                tunnel: [w1622] -> w1501
                tunnel: w1503 -> [w1622]
                frame #0 {
                  n966 = local read "Mean force (pN)"() -> (w1556:dbl)
                  n967 = local read "Cutoff force (pN)"() -> (w1555:dbl)
                  n968 = Less Or Equal?(x=w1556, y=w1555) -> (x <= y?=w1553:bool)
                  n969 = And(x="Fish", y=w1553) -> (x .and. y?=w1554:bool)
                  n970 = case shown="True" w1554 {
                    selector: w1554 -> [w1570 _]
                    tunnel: w1567 -> [w1573 w1590]
                    tunnel: w1566 -> [_ w1589]
                    tunnel: w1565 -> [w1575 w1588]
                    tunnel: w1564 -> [w1574 w1587]
                    tunnel: w1563 -> [w1572 w1586]
                    tunnel: w1562 -> [w1571 w1585]
                    tunnel: [w1575 w1584] -> w1561
                    tunnel: [w1574 w1583] -> w1560
                    tunnel: [w1573 w1582] -> w1559
                    tunnel: [w1571 w1581] -> w1549
                    tunnel: [w1572 w1580] -> w1558
                    tunnel: w1557 -> [_ w1579]
                    tunnel: [w1570 w1578] -> w1551
                    tunnel: [FALSE w1577] -> w1550
                    tunnel: [FALSE w1576] -> w1548
                    frame False {
                    }
                    frame True {
                      n971 = while {
                        tunnel: w1590 -> [w1602]
                        tunnel: w1589 -> [w1601]
                        tunnel: w1588 -> [w1609]
                        tunnel: w1587 -> [w1608]
                        tunnel: w1586 -> [w1600]
                        tunnel: w1585 -> [w1606]
                        tunnel: [w1604] -> w1584
                        tunnel: [w1603] -> w1583
                        tunnel: [w1602] -> w1582
                        tunnel: [w1601] -> w1581
                        tunnel: [w1600] -> w1580
                        tunnel: w1579 -> [w1599]
                        tunnel: [w1592] -> w1578
                        tunnel: [w1592] -> w1577
                        tunnel: [w1591] -> w1576
                        i -> [w1598]
                        stop <- w1595 stop-if-true
                        n972 = Multiply(x=w1600, y=w1598) -> (x*y=w1607:dbl)
                        n973 = local read "Cutoff force (pN)"() -> (w1593:dbl)
                        n974 = local read "Mean force (pN)"() -> (w1594:dbl)
                        n975 = Subtract(x=w1606, y=w1607) -> (x-y=w1605:dbl)
                        n976 = Build Array(w1601, w1605) -> (w1612:dbl[])
                        n977 = Build Array(w1605, w1601) -> (w1611:dbl[])
                        n978 = Greater Or Equal?(x=w1598, y=w1599) -> (x >= y?=w1592:bool)
                        n979 = Select(t=w1612, s=w1602, f=w1611) -> (s? t:f=w1610:dbl[])
                        n980 = Greater?(x=w1594, y=w1593) -> (0:w1591:bool)
                        n981 = local read "Fish"() -> (w1596:bool)
                        n982 = Not(x=w1596) -> (.not. x?=w1597:bool)
                        n983 = call-poly <vilib>:"DAQmx Write.vi"("task/channels in"=w1609, "data"=w1610, "error in"=w1608) -> ("task out"=w1604:refnum<k21>, "error out"=w1603:errorcluster)  [unwired: 10 in, 1 out]
                        n984 = Compound Arithmetic op=OR(w1592, w1597, w1591) -> (w1595:bool)
                      }
                    }
                  }
                }
                frame #1 {
                  n985 = case shown="True" w1615 {
                    frame False {
                    }
                    frame True {
                      n986 = Wait (ms)(milliseconds to wait="Wait (ms)") -> ()  [unwired: 1 out]
                    }
                  }
                }
                frame #2 {
                  n987 = case shown="True" w1625 {
                    tunnel: w1632 -> [w1635 w1644]
                    tunnel: w1631 -> [w1634 w1643]
                    tunnel: w1630 -> [_ w1642]
                    tunnel: w1629 -> [_ w1641]
                    tunnel: w1628 -> [_ w1640]
                    tunnel: [w1635 w1639] -> w1627
                    tunnel: [w1634 w1638] -> w1626
                    tunnel: [FALSE w1637] -> w1624
                    tunnel: w1623 -> [_ w1636]
                    frame False {
                    }
                    frame True {
                      n988 = while {
                        tunnel: w1644 -> [w1676]
                        tunnel: w1643 -> [w1675]
                        tunnel: w1642 -> [w1647]
                        tunnel: w1641 -> [w1673]
                        tunnel: w1640 -> [w1672]
                        tunnel: [w1670] -> w1639
                        tunnel: [w1669] -> w1638
                        tunnel: [w1654] -> w1637
                        tunnel: w1636 -> [w1645]
                        i -> [w1661]
                        stop <- w1666 stop-if-true
                        # "If tether formed,\nimmediately change\nto new delta."
                        n989 = local read "Conv Y (nm/V)"() -> (w1648:dbl)
                        n990 = local read "Conv X (nm/V)"() -> (w1646:dbl)
                        n991 = local read "Fixed Y"() -> (w1655:dbl)
                        n992 = local read "Fixed X"() -> (w1660:dbl)
                        n993 = Select(t=w1648, s=w1647, f=w1646) -> (s? t:f=w1649:dbl)
                        n994 = local read "Cutoff force (pN)"() -> (w1662:dbl)
                        n995 = Divide(x="Delta after tether", y=w1649) -> (x/y=w1650:dbl)
                        n996 = Multiply(x=w1673, y=w1661) -> (x*y=w1674:dbl)
                        n997 = local read "Mean force (pN)"() -> (w1663:dbl)
                        n998 = Add(x=w1672, y=w1674) -> (x+y=w1657:dbl)
                        n999 = Select(t=w1655, s=w1647, f=w1660) -> (s? t:f=w1659:dbl)
                        n1000 = Greater?(x=w1663, y=w1662) -> (0:w1654:bool)
                        n1001 = Add(x=w1659, y=w1650) -> (x+y=w1658:dbl)
                        n1002 = Select(t=w1658, s=w1654, f=w1657) -> (s? t:f=w1656:dbl)
                        n1003 = local read "Fish Speed (ms)"() -> (w1668:i32)
                        n1004 = Build Array(w1645, w1656) -> (w1671:dbl[])
                        n1005 = Build Array(w1656, w1645) -> (w1652:dbl[])
                        n1006 = Select(t=w1671, s=w1647, f=w1652) -> (s? t:f=w1651:dbl[])
                        n1007 = case shown="True" w1654 {
                          tunnel: w1650 -> [_ _]
                          tunnel: w1651 -> [_ w1678]
                          frame False {
                          }
                          frame True {
                            n1008 = Array To Cluster(array=w1678) -> (cluster=w1677:cluster{"[0]":dbl, "[1]":dbl})
                            n1009 = local write "Trap position (V)"(w1677) -> ()
                          }
                        }
                        n1010 = local read "Fish"() -> (w1665:bool)
                        n1011 = Greater Or Equal?(x=w1661, y=w1668) -> (x >= y?=w1667:bool)
                        n1012 = Not(x=w1665) -> (.not. x?=w1664:bool)
                        n1013 = call-poly <vilib>:"DAQmx Write.vi"("task/channels in"=w1676, "data"=w1651, "error in"=w1675) -> ("task out"=w1670:refnum<k21>, "error out"=w1669:errorcluster)  [unwired: 10 in, 1 out]
                        n1014 = Compound Arithmetic op=OR(w1667, w1664, w1654) -> (w1666:bool)
                      }
                    }
                  }
                }
              }
              n1015 = Add(x=w1519, y=w1507) -> (x+y=w1526:dbl)
              n1016 = Decrement(x="# attempts") -> (x-1=w1534:dbl)
              n1017 = Greater Or Equal?(x=w1530, y=w1534) -> (x >= y?=w1533:bool)
              n1018 = local read "Mean force (pN)"() -> (w1532:dbl)
              n1019 = Greater?(x=w1532, y="Cutoff force (pN)") -> (0:w1527:bool)
              n1020 = Compound Arithmetic op=OR(w1501, w1514, w1527, w1533) -> (w1505:bool)
              n1021 = Or(x=w1514, y=w1501) -> (x .or. y?=w1504:bool)
              "Tether" <- w1504
              n1022 = case shown="True" w1504 {
                frame False {
                }
                frame True {
                  n1023 = call <vilib>:"Beep.vi"() -> ()  [unwired: 12 in]
                }
              }
              n1024 = node-c288() -> ()  [unwired: 1 in, 1 out]
              "Attempt #" <- w1530
            }
            n1025 = node-c288(w1486) -> ()  [unwired: 1 out]
            n1026 = flat-sequence {
              tunnel: w1476 -> [w1495]
              tunnel: [w1495] -> w1475
              tunnel: w1474 -> [w1492]
              tunnel: w1473 -> [w1491]
              tunnel: w1472 -> [w1488]
              tunnel: w1475 -> [w1497]
              frame #0 {
                w1494 = T19 1 items=["no dialog", "OK message", "continue or stop message", "OK message + warnings", "continue/stop + warnings"] ("type of dialog (OK msg:1)")
                n1027 = call <vilib>:"DAQmx Clear Task.vi"("task in"=w1492, "error in"=w1491) -> ("error out"=w1493:errorcluster)  [unwired: 13 in]
                n1028 = Not(x=w1488) -> (.not. x?=w1489:bool)
                n1029 = local write "Fish"(w1489) -> ()
                n1030 = Wait (ms)(milliseconds to wait=u32 300) -> ()  [unwired: 1 out]
                n1031 = call <vilib>:"Simple Error Handler.vi"("type of dialog (OK msg:1)"=w1494, "error in (no error)"=w1493) -> ()  [unwired: 3 in, 5 out]
              }
              frame #1 {
                n1032 = And(x=w1497, y="Raster after\n tether?") -> (x .and. y?=w1498:bool)
                n1033 = case shown="True" w1498 {
                  selector: w1498 -> [_ w1500]
                  frame False {
                  }
                  frame True {
                    n1034 = property on="Raster scan" class="Bool (strict)"("Val(Sgnl)"=w1500) -> ()  [unwired: 2 in, 2 out]
                    n1035 = property on="Inject Sample" class="Bool (strict)"("Val(Sgnl)"=FALSE ("Value (Signaling)")) -> ()  [unwired: 2 in, 2 out]
                  }
                }
              }
            }
          }
        }
      }
      event "Load param": Value Change {
        n1036 = event-data() -> ()  [unwired: 1 in, 6 out]
        n1037 = property on="Scan Parameters" class="Arr (strict)"() -> ("Index Values"=w1691:u32[])  [unwired: 2 in, 2 out]
        n1038 = Index Array(array=w1691, index=0) -> (element=w1688:u32)
        n1039 = Index Array(array="Scan Parameters", index=w1688) -> (element=w1687:T22)
        n1040 = Unbundle(w1687) -> ("# scans 2"=w1686:i32)  [unwired: 4 out]
        n1041 = local write "Load param"(FALSE ("Load param")) -> ()
        n1042 = property on="# scans" class="DigNum (strict)"("Val(Sgnl)"=w1686) -> ()  [unwired: 2 in, 2 out]
      }
      event "# scans", "Pulling direction", "Scan range (nm)": Value Change {
        n1043 = event-data() -> ()  [unwired: 1 in, 6 out]
        n1044 = local read "Pulling direction"() -> (w1723:bool)
        n1045 = Reciprocal(x="Scan speed (nm/s)") -> (1/x=w1715:dbl)
        n1046 = local read "Conv Y (nm/V)"() -> (w1721:dbl)
        n1047 = local read "Conv X (nm/V)"() -> (w1722:dbl)
        n1048 = Multiply(x="Step size (nm)", y=w1715) -> (x*y=w1713:dbl)
        n1049 = Divide(x="Scan range (nm)", y="Step size (nm)") -> (x/y=w1720:dbl)
        n1050 = Absolute Value(x=w1720) -> (abs(x)=w1719:dbl)
        n1051 = Multiply(x=w1713, y=1000.0) -> (x*y=w1700:dbl)
        n1052 = Select(t=w1721, s=w1723, f=w1722) -> (s? t:f=w1711:dbl)
        n1053 = Multiply(x="# scans", y=2) -> (x*y=w1699:i32)
        n1054 = To Unsigned Quad Integer(1:w1719) -> (0:w1709:u64)
        "Scan steps (mirror)" <- w1709
        n1055 = Divide(x="Scan range (nm)", y=w1711) -> (x/y=→"Scan range (V)":dbl)
        n1056 = Multiply(x=w1709, y=w1700) -> (x*y=w1708:dbl)
        n1057 = Divide(x="Step size (nm)", y=w1711) -> (x/y=→"Scan increment (V)":dbl)
        n1058 = Round Toward +Infinity(x=w1700) -> (ceil(x): smallest int >= x=w1697:dbl)
        "Time per step (ms)" <- w1697
        n1059 = local read "Data update period (s/set)"() -> (w1703:dbl)
        n1060 = Multiply(x=w1699, y=w1708) -> (x*y=w1706:dbl)
        n1061 = local read "Pulling direction"() -> (w1692:bool)
        n1062 = Divide(x=w1706, y=1000.0) -> (x/y=w1704:dbl)
        "Total raster time (s)" <- w1704
        n1063 = local read "Data update period (s/set)"() -> (w1695:dbl)
        n1064 = case shown="False" w1692 {
          frame False {
            n1065 = local read "Fixed Y"() -> (w1726:dbl)
            n1066 = local read "Trap delta (nm)"() -> (w1731:dbl)
            n1067 = local read "Conv X (nm/V)"() -> (w1730:dbl)
            n1068 = local read "Fixed X"() -> (w1728:dbl)
            n1069 = Divide(x=w1731, y=w1730) -> (x/y=w1729:dbl)
            n1070 = Add(x=w1729, y=w1728) -> (x+y=w1727:dbl)
            n1071 = Build Array(w1727, w1726) -> (w1725:dbl[])
            n1072 = Array To Cluster(array=w1725) -> (cluster=w1724:cluster{"[0]":dbl, "[1]":dbl})
            n1073 = property on="Trap position (V)" class="Clust (strict)"("Val(Sgnl)"=w1724) -> ()  [unwired: 2 in, 2 out]
          }
          frame True {
            n1074 = local read "Trap delta (nm)"() -> (w1739:dbl)
            n1075 = local read "Conv Y (nm/V)"() -> (w1738:dbl)
            n1076 = local read "Fixed X"() -> (w1734:dbl)
            n1077 = local read "Fixed Y"() -> (w1736:dbl)
            n1078 = Divide(x=w1739, y=w1738) -> (x/y=w1737:dbl)
            n1079 = Add(x=w1737, y=w1736) -> (x+y=w1735:dbl)
            n1080 = Build Array(w1734, w1735) -> (w1733:dbl[])
            n1081 = Array To Cluster(array=w1733) -> (cluster=w1732:cluster{"[0]":dbl, "[1]":dbl})
            n1082 = property on="Trap position (V)" class="Clust (strict)"("Val(Sgnl)"=w1732) -> ()  [unwired: 2 in, 2 out]
          }
        }
        n1083 = Divide(x=w1704, y=w1703) -> (x/y=w1702:dbl)
        n1084 = Round Toward -Infinity(1:w1702) -> (0:→"N sets to be saved":dbl)
        n1085 = Multiply(x=w1695, y=1000.0) -> (x*y=w1693:dbl)
        n1086 = Less?(x=w1697, y=w1693) -> (x < y?=w1696:bool)
        n1087 = case shown="True" w1696 {
          selector: w1696 -> [_ w1740]
          frame False {
          }
          frame True {
            n1088 = call "Display Message to User"("Enable"=w1740) -> ()  [unwired: 9 in, 2 out]
          }
        }
      }
      event "Averaging Number": Value Change {
        n1089 = event-data() -> ()  [unwired: 1 in, 6 out]
        n1090 = local read "# Samples/channel (in)"() -> (w1744:i32)
        n1091 = local read "Averaging Number"() -> (w1742:i32)
        n1092 = Quotient & Remainder(x=w1744, y=w1742) -> (floor(x/y)=w1743:i32)  [unwired: 1 out]
        n1093 = Multiply(x=w1743, y=w1742) -> (x*y=w1741:i32)
        n1094 = local write "# Samples/channel (in)"(w1741) -> ()
      }
    }
    n1095 = node-c288() -> ()  [unwired: 1 in, 1 out]
  }
  n1096 = call <vilib>:"Simple Error Handler.vi"("error in (no error)"=w95) -> ()  [unwired: 4 in, 5 out]
  n1097 = disable-structure shown="Enabled" {
    frame Disabled {
      n1098 = node-c288(2 ("Processor")) -> (w1750:T11)  [unwired: 3 in]
      n1099 = timed-loop "Pump Control" {
        timing: w1750 -> [_]
        timing-out: [_] -> w1749
        tunnel: refnum<visa-resource-name> "COM6" ("VISA resource name") -> [w1752]
        stop <- w1751 stop-if-true
        n1100 = node-c288() -> ()  [unwired: 1 in, 1 out]
        n1101 = event shown="[4] \"Inject Pump 1\": Value Change" {
          selector: _ -> [_ _ _ _ _ _ _ _ _]
          dyn-events: _ -> [_ _ _ _ _ _ _ _ _]
          timeout: _ -> [_ _ _ _ _ _ _ _ _]
          tunnel: w1752 -> [w1760 w1856 _ w1932 w2060 w2203 w2248 w2306 w2365]
          tunnel: [_ _ w1931 _ _ _ _ _ _] -> w1751
          event "Flush Pump 1": Value Change {
            w1761 = "\r"
            n1102 = event-data() -> ()  [unwired: 1 in, 5 out]
            n1103 = call-poly "VISA Configure Serial Port"("VISA resource name"=w1760) -> ("VISA resource name out"=w1774:refnum<visa-resource-name>, "error out"=w1775:errorcluster)  [unwired: 13 in]
            n1104 = local read "Write Wait"() -> (w1753:i32)
            n1105 = Concatenate Strings("enter pump1", w1761) -> (w1762:string)
            n1106 = flat-sequence {
              tunnel: w1775 -> [w1794]
              tunnel: w1774 -> [w1796]
              tunnel: [w1795] -> w1791
              tunnel: [w1793] -> w1790
              tunnel: w1762 -> [w1792]
              tunnel: w1791 -> [w1799]
              tunnel: [w1799] -> w1789
              tunnel: w1790 -> [w1798]
              tunnel: [w1798] -> w1788
              tunnel: w1753 -> [w1797]
              tunnel: [w1804] -> w1787
              tunnel: w1767 -> [w1803]
              tunnel: [w1800] -> w1786
              tunnel: w1789 -> [w1802]
              tunnel: w1788 -> [w1801]
              tunnel: w1787 -> [w1807]
              tunnel: [w1807] -> w1785
              tunnel: [w1806] -> w1784
              tunnel: w1786 -> [w1806]
              tunnel: w1753 -> [w1805]
              tunnel: w1785 -> [w1812]
              tunnel: [w1811] -> w1783
              tunnel: w1770 -> [w1810]
              tunnel: w1784 -> [w1809]
              tunnel: [w1808] -> w1782
              tunnel: w1783 -> [w1815]
              tunnel: [w1815] -> w1781
              tunnel: [w1814] -> w1780
              tunnel: w1782 -> [w1814]
              tunnel: w1753 -> [w1813]
              tunnel: w1781 -> [w1820]
              tunnel: [w1819] -> w1779
              tunnel: w1773 -> [w1818]
              tunnel: w1780 -> [w1817]
              tunnel: [w1816] -> w1778
              tunnel: [w1823] -> w1777
              tunnel: w1779 -> [w1823]
              tunnel: [w1822] -> w1776
              tunnel: w1778 -> [w1822]
              tunnel: w1753 -> [w1821]
              tunnel: w1777 -> [w1828]
              tunnel: w1776 -> [w1825]
              tunnel: [w1827] -> w1756
              tunnel: [w1826] -> w1754
              tunnel: [w1833] -> w1757
              tunnel: w1756 -> [w1833]
              tunnel: [w1832] -> w1755
              tunnel: w1754 -> [w1832]
              tunnel: w1753 -> [w1831]
              tunnel: w1757 -> [w1835]
              tunnel: w1755 -> [w1834]
              frame #0 {
                n1107 = VISA Write(VISA resource name=w1796, write buffer=w1792, error in (no error)=w1794) -> (VISA resource name out=w1795:refnum<visa-resource-name>, error out=w1793:errorcluster)  [unwired: 1 out]
              }
              frame #1 {
                n1108 = Wait (ms)(milliseconds to wait=w1797) -> ()  [unwired: 1 out]
              }
              frame #2 {
                n1109 = VISA Write(VISA resource name=w1802, write buffer=w1803, error in (no error)=w1801) -> (VISA resource name out=w1804:refnum<visa-resource-name>, error out=w1800:errorcluster)  [unwired: 1 out]
              }
              frame #3 {
                n1110 = Wait (ms)(milliseconds to wait=w1805) -> ()  [unwired: 1 out]
              }
              frame #4 {
                n1111 = VISA Write(VISA resource name=w1812, write buffer=w1810, error in (no error)=w1809) -> (VISA resource name out=w1811:refnum<visa-resource-name>, error out=w1808:errorcluster)  [unwired: 1 out]
              }
              frame #5 {
                n1112 = Wait (ms)(milliseconds to wait=w1813) -> ()  [unwired: 1 out]
              }
              frame #6 {
                n1113 = VISA Write(VISA resource name=w1820, write buffer=w1818, error in (no error)=w1817) -> (VISA resource name out=w1819:refnum<visa-resource-name>, error out=w1816:errorcluster)  [unwired: 1 out]
              }
              frame #7 {
                n1114 = Wait (ms)(milliseconds to wait=w1821) -> ()  [unwired: 1 out]
              }
              frame #8 {
                n1115 = Concatenate Strings("start ", "\r") -> (w1824:string)
                n1116 = VISA Write(VISA resource name=w1828, write buffer=w1824, error in (no error)=w1825) -> (VISA resource name out=w1827:refnum<visa-resource-name>, error out=w1826:errorcluster)  [unwired: 1 out]
              }
              frame #9 {
                n1117 = Wait (ms)(milliseconds to wait=w1831) -> ()  [unwired: 1 out]
              }
              frame #10 {
                n1118 = local write "Flush Pump 1"(FALSE ("Flush Pump 1")) -> ()
                n1119 = Concatenate Strings("enter main ", "\r") -> (w1839:string)
                n1120 = VISA Write(VISA resource name=w1835, write buffer=w1839, error in (no error)=w1834) -> (VISA resource name out=w1838:refnum<visa-resource-name>, error out=w1837:errorcluster)  [unwired: 1 out]
                n1121 = VISA Close(VISA resource name=w1838, error in (no error)=w1837) -> ()  [unwired: 1 out]
              }
            }
            n1122 = Concatenate Strings("set units 4 ", w1761) -> (w1767:string)
            n1123 = Multiply(x="Flush\nRate (ul/min)", y=60) -> (x*y=w1765:dbl)
            n1124 = Number To Decimal String(number=w1765) -> (decimal integer string=w1768:string)  [unwired: 1 in]
            n1125 = Concatenate Strings("set rate ", w1768, w1761) -> (w1770:string)
            n1126 = Number To Decimal String(number="Flush\nVolume (ul)") -> (decimal integer string=w1772:string)  [unwired: 1 in]
            n1127 = Concatenate Strings("set volume ", w1772, w1761) -> (w1773:string)
          }
          event "Flush Pump 2": Value Change {
            w1847 = "\r"
            n1128 = event-data() -> ()  [unwired: 1 in, 5 out]
            n1129 = call-poly "VISA Configure Serial Port"("VISA resource name"=w1856) -> ("VISA resource name out"=w1867:refnum<visa-resource-name>, "error out"=w1868:errorcluster)  [unwired: 13 in]
            n1130 = local read "Write Wait"() -> (w1842:i32)
            n1131 = Concatenate Strings("enter pump2", w1847) -> (w1848:string)
            n1132 = flat-sequence {
              tunnel: w1868 -> [w1883]
              tunnel: w1867 -> [w1885]
              tunnel: [w1884] -> w1853
              tunnel: [w1882] -> w1851
              tunnel: w1848 -> [w1881]
              tunnel: w1853 -> [w1888]
              tunnel: [w1888] -> w1852
              tunnel: w1851 -> [w1887]
              tunnel: [w1887] -> w1850
              tunnel: w1842 -> [w1886]
              tunnel: [w1893] -> w1880
              tunnel: w1860 -> [w1892]
              tunnel: [w1889] -> w1879
              tunnel: w1852 -> [w1891]
              tunnel: w1850 -> [w1890]
              tunnel: w1880 -> [w1896]
              tunnel: [w1896] -> w1878
              tunnel: [w1895] -> w1877
              tunnel: w1879 -> [w1895]
              tunnel: w1842 -> [w1894]
              tunnel: w1878 -> [w1901]
              tunnel: [w1900] -> w1876
              tunnel: w1863 -> [w1899]
              tunnel: w1877 -> [w1898]
              tunnel: [w1897] -> w1875
              tunnel: w1876 -> [w1904]
              tunnel: [w1904] -> w1874
              tunnel: [w1903] -> w1873
              tunnel: w1875 -> [w1903]
              tunnel: w1842 -> [w1902]
              tunnel: w1874 -> [w1909]
              tunnel: [w1908] -> w1872
              tunnel: w1866 -> [w1907]
              tunnel: w1873 -> [w1906]
              tunnel: [w1905] -> w1871
              tunnel: [w1912] -> w1870
              tunnel: w1872 -> [w1912]
              tunnel: [w1911] -> w1869
              tunnel: w1871 -> [w1911]
              tunnel: w1842 -> [w1910]
              tunnel: w1870 -> [w1919]
              tunnel: w1869 -> [w1918]
              tunnel: [w1914] -> w1846
              tunnel: [w1913] -> w1844
              tunnel: w1846 -> [w1922]
              tunnel: [w1922] -> w1845
              tunnel: w1844 -> [w1921]
              tunnel: [w1921] -> w1843
              tunnel: w1842 -> [w1920]
              tunnel: w1845 -> [w1926]
              tunnel: w1843 -> [w1925]
              frame #0 {
                n1133 = VISA Write(VISA resource name=w1885, write buffer=w1881, error in (no error)=w1883) -> (VISA resource name out=w1884:refnum<visa-resource-name>, error out=w1882:errorcluster)  [unwired: 1 out]
              }
              frame #1 {
                n1134 = Wait (ms)(milliseconds to wait=w1886) -> ()  [unwired: 1 out]
              }
              frame #2 {
                n1135 = VISA Write(VISA resource name=w1891, write buffer=w1892, error in (no error)=w1890) -> (VISA resource name out=w1893:refnum<visa-resource-name>, error out=w1889:errorcluster)  [unwired: 1 out]
              }
              frame #3 {
                n1136 = Wait (ms)(milliseconds to wait=w1894) -> ()  [unwired: 1 out]
              }
              frame #4 {
                n1137 = VISA Write(VISA resource name=w1901, write buffer=w1899, error in (no error)=w1898) -> (VISA resource name out=w1900:refnum<visa-resource-name>, error out=w1897:errorcluster)  [unwired: 1 out]
              }
              frame #5 {
                n1138 = Wait (ms)(milliseconds to wait=w1902) -> ()  [unwired: 1 out]
              }
              frame #6 {
                n1139 = VISA Write(VISA resource name=w1909, write buffer=w1907, error in (no error)=w1906) -> (VISA resource name out=w1908:refnum<visa-resource-name>, error out=w1905:errorcluster)  [unwired: 1 out]
              }
              frame #7 {
                n1140 = Wait (ms)(milliseconds to wait=w1910) -> ()  [unwired: 1 out]
              }
              frame #8 {
                n1141 = Concatenate Strings("start ", "\r") -> (w1917:string)
                n1142 = VISA Write(VISA resource name=w1919, write buffer=w1917, error in (no error)=w1918) -> (VISA resource name out=w1914:refnum<visa-resource-name>, error out=w1913:errorcluster)  [unwired: 1 out]
              }
              frame #9 {
                n1143 = Wait (ms)(milliseconds to wait=w1920) -> ()  [unwired: 1 out]
              }
              frame #10 {
                n1144 = local write "Flush Pump 2"(FALSE ("Flush Pump 1")) -> ()
                n1145 = Concatenate Strings("enter main ", "\r") -> (w1927:string)
                n1146 = VISA Write(VISA resource name=w1926, write buffer=w1927, error in (no error)=w1925) -> (VISA resource name out=w1924:refnum<visa-resource-name>, error out=w1923:errorcluster)  [unwired: 1 out]
                n1147 = VISA Close(VISA resource name=w1924, error in (no error)=w1923) -> ()  [unwired: 1 out]
              }
            }
            n1148 = Concatenate Strings("set units 4 ", w1847) -> (w1860:string)
            n1149 = Multiply(x="Flush \nRate (ul/min)  2", y=60) -> (x*y=w1858:dbl)
            n1150 = Number To Decimal String(number=w1858) -> (decimal integer string=w1861:string)  [unwired: 1 in]
            n1151 = Concatenate Strings("set rate ", w1861, w1847) -> (w1863:string)
            n1152 = Number To Decimal String(number="Flush\nVolume (ul)  2") -> (decimal integer string=w1865:string)  [unwired: 1 in]
            n1153 = Concatenate Strings("set volume ", w1865, w1847) -> (w1866:string)
          }
          event "Stop": Value Change {
            n1154 = event-data() -> ()  [unwired: 1 in, 5 out]
            n1155 = local read "Stop"() -> (w1931:bool)
          }
          event "Inject Pump 2": Value Change {
            n1156 = event-data() -> ()  [unwired: 1 in, 5 out]
            n1157 = case shown="True" "Inject Pump 2" {
              tunnel: w1932 -> [w1935 w1977]
              frame False {
                n1158 = local read "Write Wait"() -> (w1934:i32)
                n1159 = call-poly "VISA Configure Serial Port"("VISA resource name"=w1935) -> ("VISA resource name out"=w1939:refnum<visa-resource-name>, "error out"=w1940:errorcluster)  [unwired: 13 in]
                n1160 = Concatenate Strings("enter pump2", "\r") -> (w1937:string)
                n1161 = flat-sequence {
                  tunnel: w1940 -> [w1951]
                  tunnel: w1939 -> [w1953]
                  tunnel: [w1952] -> w1948
                  tunnel: [w1950] -> w1947
                  tunnel: w1937 -> [w1949]
                  tunnel: w1948 -> [w1956]
                  tunnel: w1947 -> [w1955]
                  tunnel: [w1956] -> w1946
                  tunnel: [w1955] -> w1945
                  tunnel: w1934 -> [w1954]
                  tunnel: [w1960] -> w1944
                  tunnel: [w1959] -> w1943
                  tunnel: w1946 -> [w1958]
                  tunnel: w1945 -> [w1957]
                  tunnel: w1944 -> [w1966]
                  tunnel: [w1966] -> w1942
                  tunnel: w1943 -> [w1965]
                  tunnel: [w1965] -> w1941
                  tunnel: w1934 -> [w1964]
                  tunnel: w1942 -> [w1970]
                  tunnel: w1941 -> [w1969]
                  frame #0 {
                    n1162 = VISA Write(VISA resource name=w1953, write buffer=w1949, error in (no error)=w1951) -> (VISA resource name out=w1952:refnum<visa-resource-name>, error out=w1950:errorcluster)  [unwired: 1 out]
                  }
                  frame #1 {
                    n1163 = Wait (ms)(milliseconds to wait=w1954) -> ()  [unwired: 1 out]
                  }
                  frame #2 {
                    n1164 = Concatenate Strings("stop ", "\r") -> (w1963:string)
                    n1165 = VISA Write(VISA resource name=w1958, write buffer=w1963, error in (no error)=w1957) -> (VISA resource name out=w1960:refnum<visa-resource-name>, error out=w1959:errorcluster)  [unwired: 1 out]
                  }
                  frame #3 {
                    n1166 = Wait (ms)(milliseconds to wait=w1964) -> ()  [unwired: 1 out]
                  }
                  frame #4 {
                    n1167 = Concatenate Strings("enter main ", "\r") -> (w1971:string)
                    n1168 = VISA Write(VISA resource name=w1970, write buffer=w1971, error in (no error)=w1969) -> (VISA resource name out=w1968:refnum<visa-resource-name>, error out=w1967:errorcluster)  [unwired: 1 out]
                    n1169 = VISA Close(VISA resource name=w1968, error in (no error)=w1967) -> ()  [unwired: 1 out]
                  }
                }
              }
              frame True {
                w1990 = "\r"
                n1170 = call-poly "VISA Configure Serial Port"("VISA resource name"=w1977) -> ("VISA resource name out"=w1979:refnum<visa-resource-name>, "error out"=w1978:errorcluster)  [unwired: 13 in]
                n1171 = local read "Write Wait"() -> (w1974:i32)
                n1172 = Concatenate Strings("enter pump2", w1990) -> (w1989:string)
                n1173 = flat-sequence {
                  tunnel: w1978 -> [w2013]
                  tunnel: w1979 -> [w2015]
                  tunnel: [w2014] -> w2010
                  tunnel: [w2012] -> w2009
                  tunnel: w1989 -> [w2011]
                  tunnel: w2010 -> [w2018]
                  tunnel: [w2018] -> w2008
                  tunnel: w2009 -> [w2017]
                  tunnel: [w2017] -> w2007
                  tunnel: w1974 -> [w2016]
                  tunnel: [w2023] -> w2006
                  tunnel: w1986 -> [w2022]
                  tunnel: [w2019] -> w2005
                  tunnel: w2008 -> [w2021]
                  tunnel: w2007 -> [w2020]
                  tunnel: w2006 -> [w2026]
                  tunnel: [w2026] -> w2004
                  tunnel: [w2025] -> w2003
                  tunnel: w2005 -> [w2025]
                  tunnel: w1974 -> [w2024]
                  tunnel: w2004 -> [w2031]
                  tunnel: [w2030] -> w2002
                  tunnel: w1983 -> [w2029]
                  tunnel: w2003 -> [w2028]
                  tunnel: [w2027] -> w2001
                  tunnel: w2002 -> [w2034]
                  tunnel: [w2034] -> w2000
                  tunnel: [w2033] -> w1999
                  tunnel: w2001 -> [w2033]
                  tunnel: w1974 -> [w2032]
                  tunnel: w2000 -> [w2039]
                  tunnel: [w2038] -> w1998
                  tunnel: w1980 -> [w2037]
                  tunnel: w1999 -> [w2036]
                  tunnel: [w2035] -> w1997
                  tunnel: [w2042] -> w1996
                  tunnel: w1998 -> [w2042]
                  tunnel: [w2041] -> w1995
                  tunnel: w1997 -> [w2041]
                  tunnel: w1974 -> [w2040]
                  tunnel: w1996 -> [w2049]
                  tunnel: w1995 -> [w2048]
                  tunnel: [w2044] -> w1994
                  tunnel: [w2043] -> w1993
                  tunnel: w1994 -> [w2052]
                  tunnel: [w2052] -> w1992
                  tunnel: w1993 -> [w2051]
                  tunnel: [w2051] -> w1991
                  tunnel: w1974 -> [w2050]
                  tunnel: w1992 -> [w2056]
                  tunnel: w1991 -> [w2055]
                  frame #0 {
                    n1174 = VISA Write(VISA resource name=w2015, write buffer=w2011, error in (no error)=w2013) -> (VISA resource name out=w2014:refnum<visa-resource-name>, error out=w2012:errorcluster)  [unwired: 1 out]
                  }
                  frame #1 {
                    n1175 = Wait (ms)(milliseconds to wait=w2016) -> ()  [unwired: 1 out]
                  }
                  frame #2 {
                    n1176 = VISA Write(VISA resource name=w2021, write buffer=w2022, error in (no error)=w2020) -> (VISA resource name out=w2023:refnum<visa-resource-name>, error out=w2019:errorcluster)  [unwired: 1 out]
                  }
                  frame #3 {
                    n1177 = Wait (ms)(milliseconds to wait=w2024) -> ()  [unwired: 1 out]
                  }
                  frame #4 {
                    n1178 = VISA Write(VISA resource name=w2031, write buffer=w2029, error in (no error)=w2028) -> (VISA resource name out=w2030:refnum<visa-resource-name>, error out=w2027:errorcluster)  [unwired: 1 out]
                  }
                  frame #5 {
                    n1179 = Wait (ms)(milliseconds to wait=w2032) -> ()  [unwired: 1 out]
                  }
                  frame #6 {
                    n1180 = VISA Write(VISA resource name=w2039, write buffer=w2037, error in (no error)=w2036) -> (VISA resource name out=w2038:refnum<visa-resource-name>, error out=w2035:errorcluster)  [unwired: 1 out]
                  }
                  frame #7 {
                    n1181 = Wait (ms)(milliseconds to wait=w2040) -> ()  [unwired: 1 out]
                  }
                  frame #8 {
                    n1182 = Concatenate Strings("start ", "\r") -> (w2047:string)
                    n1183 = VISA Write(VISA resource name=w2049, write buffer=w2047, error in (no error)=w2048) -> (VISA resource name out=w2044:refnum<visa-resource-name>, error out=w2043:errorcluster)  [unwired: 1 out]
                  }
                  frame #9 {
                    n1184 = Wait (ms)(milliseconds to wait=w2050) -> ()  [unwired: 1 out]
                  }
                  frame #10 {
                    n1185 = Concatenate Strings("enter main ", "\r") -> (w2057:string)
                    n1186 = VISA Write(VISA resource name=w2056, write buffer=w2057, error in (no error)=w2055) -> (VISA resource name out=w2054:refnum<visa-resource-name>, error out=w2053:errorcluster)  [unwired: 1 out]
                    n1187 = VISA Close(VISA resource name=w2054, error in (no error)=w2053) -> ()  [unwired: 1 out]
                  }
                }
                n1188 = local read "Normal \nRate (ul/hr)  2"() -> (w1975:dbl)
                n1189 = Concatenate Strings("set units 4 ", w1990) -> (w1986:string)
                n1190 = local read "Normal \nVolume (ul) 2"() -> (w1976:dbl)
                n1191 = Number To Decimal String(number=w1975) -> (decimal integer string=w1985:string)  [unwired: 1 in]
                n1192 = Concatenate Strings("set rate ", w1985, w1990) -> (w1983:string)
                n1193 = Number To Decimal String(number=w1976) -> (decimal integer string=w1981:string)  [unwired: 1 in]
                n1194 = Concatenate Strings("set volume ", w1981, w1990) -> (w1980:string)
              }
            }
          }
          event "Inject Pump 1": Value Change {
            n1195 = event-data() -> ()  [unwired: 1 in, 5 out]
            n1196 = case shown="True" "Inject Pump 1" {
              tunnel: w2060 -> [w2063 w2105]
              frame False {
                n1197 = local read "Write Wait"() -> (w2062:i32)
                n1198 = call-poly "VISA Configure Serial Port"("VISA resource name"=w2063) -> ("VISA resource name out"=w2067:refnum<visa-resource-name>, "error out"=w2068:errorcluster)  [unwired: 13 in]
                n1199 = Concatenate Strings("enter pump1", "\r") -> (w2065:string)
                n1200 = flat-sequence {
                  tunnel: w2068 -> [w2079]
                  tunnel: w2067 -> [w2081]
                  tunnel: [w2080] -> w2076
                  tunnel: [w2078] -> w2075
                  tunnel: w2065 -> [w2077]
                  tunnel: w2076 -> [w2084]
                  tunnel: w2075 -> [w2083]
                  tunnel: [w2084] -> w2074
                  tunnel: [w2083] -> w2073
                  tunnel: w2062 -> [w2082]
                  tunnel: [w2088] -> w2072
                  tunnel: [w2087] -> w2071
                  tunnel: w2074 -> [w2086]
                  tunnel: w2073 -> [w2085]
                  tunnel: w2072 -> [w2094]
                  tunnel: [w2094] -> w2070
                  tunnel: w2071 -> [w2093]
                  tunnel: [w2093] -> w2069
                  tunnel: w2062 -> [w2092]
                  tunnel: w2070 -> [w2098]
                  tunnel: w2069 -> [w2097]
                  frame #0 {
                    n1201 = VISA Write(VISA resource name=w2081, write buffer=w2077, error in (no error)=w2079) -> (VISA resource name out=w2080:refnum<visa-resource-name>, error out=w2078:errorcluster)  [unwired: 1 out]
                  }
                  frame #1 {
                    n1202 = Wait (ms)(milliseconds to wait=w2082) -> ()  [unwired: 1 out]
                  }
                  frame #2 {
                    n1203 = Concatenate Strings("stop ", "\r") -> (w2091:string)
                    n1204 = VISA Write(VISA resource name=w2086, write buffer=w2091, error in (no error)=w2085) -> (VISA resource name out=w2088:refnum<visa-resource-name>, error out=w2087:errorcluster)  [unwired: 1 out]
                  }
                  frame #3 {
                    n1205 = Wait (ms)(milliseconds to wait=w2092) -> ()  [unwired: 1 out]
                  }
                  frame #4 {
                    n1206 = Concatenate Strings("enter main ", "\r") -> (w2099:string)
                    n1207 = VISA Write(VISA resource name=w2098, write buffer=w2099, error in (no error)=w2097) -> (VISA resource name out=w2096:refnum<visa-resource-name>, error out=w2095:errorcluster)  [unwired: 1 out]
                    n1208 = VISA Close(VISA resource name=w2096, error in (no error)=w2095) -> ()  [unwired: 1 out]
                  }
                }
              }
              frame True {
                w2118 = "\r"
                n1209 = call-poly "VISA Configure Serial Port"("VISA resource name"=w2105) -> ("VISA resource name out"=w2107:refnum<visa-resource-name>, "error out"=w2106:errorcluster)  [unwired: 13 in]
                n1210 = local read "Write Wait"() -> (w2102:i32)
                n1211 = flat-sequence {
                  tunnel: w2106 -> [w2141]
                  tunnel: w2107 -> [w2143]
                  tunnel: [w2142] -> w2138
                  tunnel: [w2140] -> w2137
                  tunnel: w2117 -> [w2139]
                  tunnel: w2138 -> [w2146]
                  tunnel: [w2146] -> w2136
                  tunnel: w2137 -> [w2145]
                  tunnel: [w2145] -> w2135
                  tunnel: w2102 -> [w2144]
                  tunnel: [w2151] -> w2134
                  tunnel: w2114 -> [w2150]
                  tunnel: [w2147] -> w2133
                  tunnel: w2136 -> [w2149]
                  tunnel: w2135 -> [w2148]
                  tunnel: w2134 -> [w2154]
                  tunnel: [w2154] -> w2132
                  tunnel: [w2153] -> w2131
                  tunnel: w2133 -> [w2153]
                  tunnel: w2102 -> [w2152]
                  tunnel: w2132 -> [w2159]
                  tunnel: [w2158] -> w2130
                  tunnel: w2111 -> [w2157]
                  tunnel: w2131 -> [w2156]
                  tunnel: [w2155] -> w2129
                  tunnel: w2130 -> [w2162]
                  tunnel: [w2162] -> w2128
                  tunnel: [w2161] -> w2127
                  tunnel: w2129 -> [w2161]
                  tunnel: w2102 -> [w2160]
                  tunnel: w2128 -> [w2167]
                  tunnel: [w2166] -> w2126
                  tunnel: w2108 -> [w2165]
                  tunnel: w2127 -> [w2164]
                  tunnel: [w2163] -> w2125
                  tunnel: [w2170] -> w2124
                  tunnel: w2126 -> [w2170]
                  tunnel: [w2169] -> w2123
                  tunnel: w2125 -> [w2169]
                  tunnel: w2102 -> [w2168]
                  tunnel: w2124 -> [w2177]
                  tunnel: w2123 -> [w2176]
                  tunnel: [w2172] -> w2122
                  tunnel: [w2171] -> w2121
                  tunnel: w2122 -> [w2180]
                  tunnel: [w2180] -> w2120
                  tunnel: w2121 -> [w2179]
                  tunnel: [w2179] -> w2119
                  tunnel: w2102 -> [w2178]
                  tunnel: w2120 -> [w2184]
                  tunnel: w2119 -> [w2183]
                  frame #0 {
                    n1212 = VISA Write(VISA resource name=w2143, write buffer=w2139, error in (no error)=w2141) -> (VISA resource name out=w2142:refnum<visa-resource-name>, error out=w2140:errorcluster)  [unwired: 1 out]
                  }
                  frame #1 {
                    n1213 = Wait (ms)(milliseconds to wait=w2144) -> ()  [unwired: 1 out]
                  }
                  frame #2 {
                    n1214 = VISA Write(VISA resource name=w2149, write buffer=w2150, error in (no error)=w2148) -> (VISA resource name out=w2151:refnum<visa-resource-name>, error out=w2147:errorcluster)  [unwired: 1 out]
                  }
                  frame #3 {
                    n1215 = Wait (ms)(milliseconds to wait=w2152) -> ()  [unwired: 1 out]
                  }
                  frame #4 {
                    n1216 = VISA Write(VISA resource name=w2159, write buffer=w2157, error in (no error)=w2156) -> (VISA resource name out=w2158:refnum<visa-resource-name>, error out=w2155:errorcluster)  [unwired: 1 out]
                  }
                  frame #5 {
                    n1217 = Wait (ms)(milliseconds to wait=w2160) -> ()  [unwired: 1 out]
                  }
                  frame #6 {
                    n1218 = VISA Write(VISA resource name=w2167, write buffer=w2165, error in (no error)=w2164) -> (VISA resource name out=w2166:refnum<visa-resource-name>, error out=w2163:errorcluster)  [unwired: 1 out]
                  }
                  frame #7 {
                    n1219 = Wait (ms)(milliseconds to wait=w2168) -> ()  [unwired: 1 out]
                  }
                  frame #8 {
                    n1220 = Concatenate Strings("start ", "\r") -> (w2175:string)
                    n1221 = VISA Write(VISA resource name=w2177, write buffer=w2175, error in (no error)=w2176) -> (VISA resource name out=w2172:refnum<visa-resource-name>, error out=w2171:errorcluster)  [unwired: 1 out]
                  }
                  frame #9 {
                    n1222 = Wait (ms)(milliseconds to wait=w2178) -> ()  [unwired: 1 out]
                  }
                  frame #10 {
                    n1223 = Concatenate Strings("enter main ", "\r") -> (w2185:string)
                    n1224 = VISA Write(VISA resource name=w2184, write buffer=w2185, error in (no error)=w2183) -> (VISA resource name out=w2182:refnum<visa-resource-name>, error out=w2181:errorcluster)  [unwired: 1 out]
                    n1225 = VISA Close(VISA resource name=w2182, error in (no error)=w2181) -> ()  [unwired: 1 out]
                  }
                }
                n1226 = Concatenate Strings("enter pump1", w2118) -> (w2117:string)
                n1227 = local read "Normal \nRate (ul/hr)"() -> (w2103:dbl)
                n1228 = Concatenate Strings("set units 4 ", w2118) -> (w2114:string)
                n1229 = local read "Normal \nVolume (ul)"() -> (w2104:dbl)
                n1230 = Number To Decimal String(number=w2103) -> (decimal integer string=w2113:string)  [unwired: 1 in]
                n1231 = Concatenate Strings("set rate ", w2113, w2118) -> (w2111:string)
                n1232 = Number To Decimal String(number=w2104) -> (decimal integer string=w2109:string)  [unwired: 1 in]
                n1233 = Concatenate Strings("set volume ", w2109, w2118) -> (w2108:string)
              }
            }
          }
          event "Normal \nVolume (ul)": Value Change {
            n1234 = event-data() -> ()  [unwired: 1 in, 5 out]
            n1235 = call-poly "VISA Configure Serial Port"("VISA resource name"=w2203) -> ("VISA resource name out"=w2205:refnum<visa-resource-name>, "error out"=w2204:errorcluster)  [unwired: 13 in]
            n1236 = local read "Write Wait"() -> (w2188:i32)
            n1237 = Concatenate Strings("enter pump1", "\r") -> (w2207:string)
            n1238 = flat-sequence {
              tunnel: w2204 -> [w2217]
              tunnel: w2205 -> [w2219]
              tunnel: [w2218] -> w2197
              tunnel: [w2216] -> w2196
              tunnel: w2207 -> [w2215]
              tunnel: w2197 -> [w2222]
              tunnel: [w2222] -> w2195
              tunnel: w2196 -> [w2221]
              tunnel: [w2221] -> w2193
              tunnel: w2188 -> [w2220]
              tunnel: w2195 -> [w2226]
              tunnel: [w2227] -> w2194
              tunnel: w2193 -> [w2225]
              tunnel: [w2224] -> w2192
              tunnel: w2189 -> [w2223]
              tunnel: w2194 -> [w2230]
              tunnel: w2192 -> [w2229]
              tunnel: [w2230] -> w2214
              tunnel: [w2229] -> w2213
              tunnel: w2188 -> [w2228]
              tunnel: [w2235] -> w2212
              tunnel: [w2234] -> w2211
              tunnel: w2214 -> [w2233]
              tunnel: w2213 -> [w2232]
              tunnel: w2198 -> [w2231]
              tunnel: w2212 -> [w2238]
              tunnel: [w2238] -> w2210
              tunnel: w2211 -> [w2237]
              tunnel: [w2237] -> w2209
              tunnel: w2188 -> [w2236]
              tunnel: w2210 -> [w2242]
              tunnel: w2209 -> [w2241]
              frame #0 {
                n1239 = VISA Write(VISA resource name=w2219, write buffer=w2215, error in (no error)=w2217) -> (VISA resource name out=w2218:refnum<visa-resource-name>, error out=w2216:errorcluster)  [unwired: 1 out]
              }
              frame #1 {
                n1240 = Wait (ms)(milliseconds to wait=w2220) -> ()  [unwired: 1 out]
              }
              frame #2 {
                n1241 = VISA Write(VISA resource name=w2226, write buffer=w2223, error in (no error)=w2225) -> (VISA resource name out=w2227:refnum<visa-resource-name>, error out=w2224:errorcluster)  [unwired: 1 out]
              }
              frame #3 {
                n1242 = Wait (ms)(milliseconds to wait=w2228) -> ()  [unwired: 1 out]
              }
              frame #4 {
                n1243 = VISA Write(VISA resource name=w2233, write buffer=w2231, error in (no error)=w2232) -> (VISA resource name out=w2235:refnum<visa-resource-name>, error out=w2234:errorcluster)  [unwired: 1 out]
              }
              frame #5 {
                n1244 = Wait (ms)(milliseconds to wait=w2236) -> ()  [unwired: 1 out]
              }
              frame #6 {
                n1245 = Concatenate Strings("enter main ", "\r") -> (w2243:string)
                n1246 = VISA Write(VISA resource name=w2242, write buffer=w2243, error in (no error)=w2241) -> (VISA resource name out=w2240:refnum<visa-resource-name>, error out=w2239:errorcluster)  [unwired: 1 out]
                n1247 = VISA Close(VISA resource name=w2240, error in (no error)=w2239) -> ()  [unwired: 1 out]
              }
            }
            n1248 = Concatenate Strings("set units 4", "\r") -> (w2189:string)
            n1249 = Number To Decimal String(number="Normal \nVolume (ul)") -> (decimal integer string=w2200:string)  [unwired: 1 in]
            n1250 = Concatenate Strings("set volume", w2200, "\r") -> (w2198:string)
          }
          event "Normal \nRate (ul/hr)": Value Change {
            n1251 = event-data() -> ()  [unwired: 1 in, 5 out]
            n1252 = call-poly "VISA Configure Serial Port"("VISA resource name"=w2248) -> ("VISA resource name out"=w2256:refnum<visa-resource-name>, "error out"=w2255:errorcluster)  [unwired: 13 in]
            n1253 = local read "Write Wait"() -> (w2246:i32)
            n1254 = Concatenate Strings("enter pump1", "\r") -> (w2258:string)
            n1255 = flat-sequence {
              tunnel: w2255 -> [w2275]
              tunnel: w2256 -> [w2277]
              tunnel: [w2276] -> w2271
              tunnel: [w2274] -> w2270
              tunnel: w2258 -> [w2273]
              tunnel: w2271 -> [w2280]
              tunnel: [w2280] -> w2269
              tunnel: w2270 -> [w2279]
              tunnel: [w2279] -> w2268
              tunnel: w2246 -> [w2278]
              tunnel: w2269 -> [w2284]
              tunnel: [w2285] -> w2267
              tunnel: w2268 -> [w2283]
              tunnel: [w2282] -> w2266
              tunnel: w2249 -> [w2281]
              tunnel: w2267 -> [w2288]
              tunnel: w2266 -> [w2287]
              tunnel: [w2288] -> w2265
              tunnel: [w2287] -> w2264
              tunnel: w2246 -> [w2286]
              tunnel: [w2293] -> w2263
              tunnel: [w2292] -> w2262
              tunnel: w2265 -> [w2291]
              tunnel: w2264 -> [w2290]
              tunnel: w2252 -> [w2289]
              tunnel: w2263 -> [w2296]
              tunnel: [w2296] -> w2261
              tunnel: w2262 -> [w2295]
              tunnel: [w2295] -> w2260
              tunnel: w2246 -> [w2294]
              tunnel: w2261 -> [w2300]
              tunnel: w2260 -> [w2299]
              frame #0 {
                n1256 = VISA Write(VISA resource name=w2277, write buffer=w2273, error in (no error)=w2275) -> (VISA resource name out=w2276:refnum<visa-resource-name>, error out=w2274:errorcluster)  [unwired: 1 out]
              }
              frame #1 {
                n1257 = Wait (ms)(milliseconds to wait=w2278) -> ()  [unwired: 1 out]
              }
              frame #2 {
                n1258 = VISA Write(VISA resource name=w2284, write buffer=w2281, error in (no error)=w2283) -> (VISA resource name out=w2285:refnum<visa-resource-name>, error out=w2282:errorcluster)  [unwired: 1 out]
              }
              frame #3 {
                n1259 = Wait (ms)(milliseconds to wait=w2286) -> ()  [unwired: 1 out]
              }
              frame #4 {
                n1260 = VISA Write(VISA resource name=w2291, write buffer=w2289, error in (no error)=w2290) -> (VISA resource name out=w2293:refnum<visa-resource-name>, error out=w2292:errorcluster)  [unwired: 1 out]
              }
              frame #5 {
                n1261 = Wait (ms)(milliseconds to wait=w2294) -> ()  [unwired: 1 out]
              }
              frame #6 {
                n1262 = Concatenate Strings("enter main ", "\r") -> (w2301:string)
                n1263 = VISA Write(VISA resource name=w2300, write buffer=w2301, error in (no error)=w2299) -> (VISA resource name out=w2298:refnum<visa-resource-name>, error out=w2297:errorcluster)  [unwired: 1 out]
                n1264 = VISA Close(VISA resource name=w2298, error in (no error)=w2297) -> ()  [unwired: 1 out]
              }
            }
            n1265 = Concatenate Strings("set units 4", "\r") -> (w2249:string)
            n1266 = Number To Decimal String(number="Normal \nRate (ul/hr)") -> (decimal integer string=w2247:string)  [unwired: 1 in]
            n1267 = Concatenate Strings("set rate", w2247, "\r") -> (w2252:string)
          }
          event "Normal \nRate (ul/hr)  2": Value Change {
            n1268 = event-data() -> ()  [unwired: 1 in, 5 out]
            n1269 = call-poly "VISA Configure Serial Port"("VISA resource name"=w2306) -> ("VISA resource name out"=w2314:refnum<visa-resource-name>, "error out"=w2313:errorcluster)  [unwired: 13 in]
            n1270 = local read "Write Wait"() -> (w2304:i32)
            n1271 = Concatenate Strings("enter pump2", "\r") -> (w2316:string)
            n1272 = flat-sequence {
              tunnel: w2313 -> [w2333]
              tunnel: w2314 -> [w2335]
              tunnel: [w2334] -> w2329
              tunnel: [w2332] -> w2328
              tunnel: w2316 -> [w2331]
              tunnel: w2329 -> [w2338]
              tunnel: [w2338] -> w2327
              tunnel: w2328 -> [w2337]
              tunnel: [w2337] -> w2326
              tunnel: w2304 -> [w2336]
              tunnel: w2327 -> [w2342]
              tunnel: [w2343] -> w2325
              tunnel: w2326 -> [w2341]
              tunnel: [w2340] -> w2324
              tunnel: w2307 -> [w2339]
              tunnel: w2325 -> [w2346]
              tunnel: w2324 -> [w2345]
              tunnel: [w2346] -> w2323
              tunnel: [w2345] -> w2322
              tunnel: w2304 -> [w2344]
              tunnel: [w2351] -> w2321
              tunnel: [w2350] -> w2320
              tunnel: w2323 -> [w2349]
              tunnel: w2322 -> [w2348]
              tunnel: w2310 -> [w2347]
              tunnel: w2321 -> [w2354]
              tunnel: [w2354] -> w2319
              tunnel: w2320 -> [w2353]
              tunnel: [w2353] -> w2318
              tunnel: w2304 -> [w2352]
              tunnel: w2319 -> [w2358]
              tunnel: w2318 -> [w2357]
              frame #0 {
                n1273 = VISA Write(VISA resource name=w2335, write buffer=w2331, error in (no error)=w2333) -> (VISA resource name out=w2334:refnum<visa-resource-name>, error out=w2332:errorcluster)  [unwired: 1 out]
              }
              frame #1 {
                n1274 = Wait (ms)(milliseconds to wait=w2336) -> ()  [unwired: 1 out]
              }
              frame #2 {
                n1275 = VISA Write(VISA resource name=w2342, write buffer=w2339, error in (no error)=w2341) -> (VISA resource name out=w2343:refnum<visa-resource-name>, error out=w2340:errorcluster)  [unwired: 1 out]
              }
              frame #3 {
                n1276 = Wait (ms)(milliseconds to wait=w2344) -> ()  [unwired: 1 out]
              }
              frame #4 {
                n1277 = VISA Write(VISA resource name=w2349, write buffer=w2347, error in (no error)=w2348) -> (VISA resource name out=w2351:refnum<visa-resource-name>, error out=w2350:errorcluster)  [unwired: 1 out]
              }
              frame #5 {
                n1278 = Wait (ms)(milliseconds to wait=w2352) -> ()  [unwired: 1 out]
              }
              frame #6 {
                n1279 = Concatenate Strings("enter main ", "\r") -> (w2359:string)
                n1280 = VISA Write(VISA resource name=w2358, write buffer=w2359, error in (no error)=w2357) -> (VISA resource name out=w2356:refnum<visa-resource-name>, error out=w2355:errorcluster)  [unwired: 1 out]
                n1281 = VISA Close(VISA resource name=w2356, error in (no error)=w2355) -> ()  [unwired: 1 out]
              }
            }
            n1282 = Concatenate Strings("set units 4", "\r") -> (w2307:string)
            n1283 = Number To Decimal String(number="Normal \nRate (ul/hr)  2") -> (decimal integer string=w2305:string)  [unwired: 1 in]
            n1284 = Concatenate Strings("set rate", w2305, "\r") -> (w2310:string)
          }
          event "Normal \nVolume (ul) 2": Value Change {
            n1285 = event-data() -> ()  [unwired: 1 in, 5 out]
            n1286 = call-poly "VISA Configure Serial Port"("VISA resource name"=w2365) -> ("VISA resource name out"=w2369:refnum<visa-resource-name>, "error out"=w2370:errorcluster)  [unwired: 13 in]
            n1287 = local read "Write Wait"() -> (w2362:i32)
            n1288 = Concatenate Strings("enter pump2", "\r") -> (w2367:string)
            n1289 = flat-sequence {
              tunnel: w2370 -> [w2391]
              tunnel: w2369 -> [w2393]
              tunnel: [w2392] -> w2388
              tunnel: [w2390] -> w2387
              tunnel: w2367 -> [w2389]
              tunnel: w2388 -> [w2396]
              tunnel: [w2396] -> w2386
              tunnel: w2387 -> [w2395]
              tunnel: [w2395] -> w2385
              tunnel: w2362 -> [w2394]
              tunnel: w2386 -> [w2400]
              tunnel: [w2401] -> w2384
              tunnel: w2385 -> [w2399]
              tunnel: [w2398] -> w2383
              tunnel: w2376 -> [w2397]
              tunnel: w2384 -> [w2404]
              tunnel: w2383 -> [w2403]
              tunnel: [w2404] -> w2382
              tunnel: [w2403] -> w2381
              tunnel: w2362 -> [w2402]
              tunnel: [w2409] -> w2380
              tunnel: [w2408] -> w2379
              tunnel: w2382 -> [w2407]
              tunnel: w2381 -> [w2406]
              tunnel: w2373 -> [w2405]
              tunnel: w2380 -> [w2412]
              tunnel: [w2412] -> w2378
              tunnel: w2379 -> [w2411]
              tunnel: [w2411] -> w2377
              tunnel: w2362 -> [w2410]
              tunnel: w2378 -> [w2416]
              tunnel: w2377 -> [w2415]
              frame #0 {
                n1290 = VISA Write(VISA resource name=w2393, write buffer=w2389, error in (no error)=w2391) -> (VISA resource name out=w2392:refnum<visa-resource-name>, error out=w2390:errorcluster)  [unwired: 1 out]
              }
              frame #1 {
                n1291 = Wait (ms)(milliseconds to wait=w2394) -> ()  [unwired: 1 out]
              }
              frame #2 {
                n1292 = VISA Write(VISA resource name=w2400, write buffer=w2397, error in (no error)=w2399) -> (VISA resource name out=w2401:refnum<visa-resource-name>, error out=w2398:errorcluster)  [unwired: 1 out]
              }
              frame #3 {
                n1293 = Wait (ms)(milliseconds to wait=w2402) -> ()  [unwired: 1 out]
              }
              frame #4 {
                n1294 = VISA Write(VISA resource name=w2407, write buffer=w2405, error in (no error)=w2406) -> (VISA resource name out=w2409:refnum<visa-resource-name>, error out=w2408:errorcluster)  [unwired: 1 out]
              }
              frame #5 {
                n1295 = Wait (ms)(milliseconds to wait=w2410) -> ()  [unwired: 1 out]
              }
              frame #6 {
                n1296 = Concatenate Strings("enter main ", "\r") -> (w2417:string)
                n1297 = VISA Write(VISA resource name=w2416, write buffer=w2417, error in (no error)=w2415) -> (VISA resource name out=w2414:refnum<visa-resource-name>, error out=w2413:errorcluster)  [unwired: 1 out]
                n1298 = VISA Close(VISA resource name=w2414, error in (no error)=w2413) -> ()  [unwired: 1 out]
              }
            }
            n1299 = Concatenate Strings("set units 4", "\r") -> (w2376:string)
            n1300 = Number To Decimal String(number="Normal \nVolume (ul) 2") -> (decimal integer string=w2363:string)  [unwired: 1 in]
            n1301 = Concatenate Strings("set volume", w2363, "\r") -> (w2373:string)
          }
        }
        n1302 = node-c288() -> ()  [unwired: 1 in, 1 out]
      }
      n1303 = node-c288(w1749) -> ()  [unwired: 1 out]
    }
    frame Enabled {
      n1304 = node-c288(2 ("Processor")) -> (w2429:T11)  [unwired: 3 in]
      n1305 = timed-loop "Pump Control" {
        timing: w2429 -> [_]
        timing-out: [_] -> w2428
        tunnel: refnum<visa-resource-name> "COM5" ("VISA resource name") -> [w2431]
        stop <- w2430 stop-if-true
        n1306 = node-c288() -> ()  [unwired: 1 in, 1 out]
        n1307 = event shown="[2] \"Inject Sample\": Value Change" {
          selector: _ -> [_ _ _ _ _]
          dyn-events: _ -> [_ _ _ _ _]
          timeout: _ -> [_ _ _ _ _]
          tunnel: w2431 -> [w2437 _ w2511 w2538 w2543]
          tunnel: [_ w2509 _ _ _] -> w2430
          event "Flush Sample": Value Change {
            n1308 = event-data() -> ()  [unwired: 1 in, 5 out]
            n1309 = local read "Write Wait"() -> (w2451:i32)
            n1310 = flat-sequence {
              tunnel: [w2475] -> w2471
              tunnel: [w2474] -> w2470
              tunnel: "CLD" -> [w2473]
              tunnel: w2437 -> [w2472]
              tunnel: w2471 -> [w2478]
              tunnel: [w2478] -> w2469
              tunnel: w2470 -> [w2477]
              tunnel: [w2477] -> w2468
              tunnel: w2451 -> [w2476]
              tunnel: [w2483] -> w2467
              tunnel: [w2480] -> w2466
              tunnel: w2469 -> [w2482]
              tunnel: w2468 -> [w2481]
              tunnel: "MODVOL" -> [w2479]
              tunnel: w2467 -> [w2486]
              tunnel: [w2486] -> w2465
              tunnel: [w2485] -> w2464
              tunnel: w2466 -> [w2485]
              tunnel: w2451 -> [w2484]
              tunnel: w2465 -> [w2491]
              tunnel: [w2490] -> w2463
              tunnel: w2453 -> [w2489]
              tunnel: w2464 -> [w2488]
              tunnel: [w2487] -> w2462
              tunnel: w2463 -> [w2494]
              tunnel: [w2494] -> w2461
              tunnel: [w2493] -> w2460
              tunnel: w2462 -> [w2493]
              tunnel: w2451 -> [w2492]
              tunnel: w2461 -> [w2499]
              tunnel: [w2498] -> w2459
              tunnel: w2455 -> [w2497]
              tunnel: w2460 -> [w2496]
              tunnel: [w2495] -> w2458
              tunnel: [w2502] -> w2456
              tunnel: w2459 -> [w2502]
              tunnel: [w2501] -> w2457
              tunnel: w2458 -> [w2501]
              tunnel: w2451 -> [w2500]
              tunnel: w2457 -> [w2507]
              tunnel: w2456 -> [w2508]
              tunnel: [w2506] -> w2446
              tunnel: "RUN " -> [w2505]
              frame #0 {
                n1311 = call "Write to pump 2.vi"("String to write"=w2473, "VISA resource name"=w2472) -> ("error out"=w2474:errorcluster, "VISA resource name out"=w2475:refnum<visa-resource-name>)  [unwired: 8 in]
              }
              frame #1 {
                n1312 = Wait (ms)(milliseconds to wait=w2476) -> ()  [unwired: 1 out]
              }
              frame #2 {
                n1313 = call "Write to pump 2.vi"("error in (no error)"=w2481, "String to write"=w2479, "VISA resource name"=w2482) -> ("error out"=w2480:errorcluster, "VISA resource name out"=w2483:refnum<visa-resource-name>)  [unwired: 7 in]
              }
              frame #3 {
                n1314 = Wait (ms)(milliseconds to wait=w2484) -> ()  [unwired: 1 out]
              }
              frame #4 {
                n1315 = call "Write to pump 2.vi"("error in (no error)"=w2488, "String to write"=w2489, "VISA resource name"=w2491) -> ("error out"=w2487:errorcluster, "VISA resource name out"=w2490:refnum<visa-resource-name>)  [unwired: 7 in]
              }
              frame #5 {
                n1316 = Wait (ms)(milliseconds to wait=w2492) -> ()  [unwired: 1 out]
              }
              frame #6 {
                n1317 = call "Write to pump 2.vi"("error in (no error)"=w2496, "String to write"=w2497, "VISA resource name"=w2499) -> ("error out"=w2495:errorcluster, "VISA resource name out"=w2498:refnum<visa-resource-name>)  [unwired: 7 in]
              }
              frame #7 {
                n1318 = Wait (ms)(milliseconds to wait=w2500) -> ()  [unwired: 1 out]
              }
              frame #8 {
                w2504 = TRUE ("Inject Pump 3")
                n1319 = Tick Count (ms)() -> (millisecond timer value=→"Flush Sample Start Time":u32)
                n1320 = call "Write to pump 2.vi"("error in (no error)"=w2507, "String to write"=w2505, "VISA resource name"=w2508) -> ("error out"=w2506:errorcluster)  [unwired: 7 in, 1 out]
                n1321 = local write "Inject Sample"(w2504) -> ()
                "Flushing Sample" <- w2504
              }
            }
            n1322 = Number To Fractional String(number="Flush \nRate (ul/min)  3") -> (F-format string=w2439:string)  [unwired: 3 in]
            n1323 = String Subset(string=w2439, length (rest)=6 ("length (rest)")) -> (substring=w2438:string)  [unwired: 1 in]
            n1324 = Concatenate Strings("RAT", w2438, "UM") -> (w2453:string)
            n1325 = Divide(x="Flush\nVolume (ul)  3", y=1000.0) -> (x/y=w2444:dbl)
            n1326 = Number To Fractional String(number=w2444) -> (F-format string=w2443:string)  [unwired: 3 in]
            n1327 = Divide(x="Flush\nVolume (ul)  3", y="Flush \nRate (ul/min)  3") -> (x/y=w2434:dbl)
            n1328 = Multiply(x=w2434, y=60.0) -> (x*y=→"Sample flush time (s)":dbl)
            n1329 = String Subset(string=w2443, length (rest)=6 ("length (rest)")) -> (substring=w2442:string)  [unwired: 1 in]
            n1330 = Concatenate Strings("TGT", w2442) -> (w2455:string)
            "error out" <- w2446
          }
          event "Stop": Value Change {
            n1331 = event-data() -> ()  [unwired: 1 in, 5 out]
            n1332 = local read "Stop"() -> (w2509:bool)
          }
          event "Inject Sample": Value Change {
            n1333 = event-data() -> ()  [unwired: 1 in, 5 out]
            n1334 = case shown="True" "Inject Sample" {
              tunnel: w2511 -> [w2513 w2514]
              frame False {
                n1335 = call "Write to pump 2.vi"("String to write"="STP", "VISA resource name"=w2513) -> ()  [unwired: 8 in, 2 out]
              }
              frame True {
                n1336 = local read "Normal \nRate (ul/hr)  3"() -> (w2515:dbl)
                n1337 = Number To Fractional String(number=w2515) -> (F-format string=w2518:string)  [unwired: 3 in]
                n1338 = String Subset(string=w2518, length (rest)=6 ("length (rest)")) -> (substring=w2516:string)  [unwired: 1 in]
                n1339 = flat-sequence {
                  tunnel: "RUN " -> [w2530]
                  tunnel: [w2532] -> _
                  tunnel: [w2531] -> _
                  tunnel: w2514 -> [w2529]
                  frame #0 {
                    n1340 = call "Write to pump 2.vi"("String to write"=w2530, "VISA resource name"=w2529) -> ("error out"=w2531:errorcluster, "VISA resource name out"=w2532:refnum<visa-resource-name>)  [unwired: 8 in]
                  }
                }
                n1341 = Concatenate Strings("RAT", w2516, "UH" ("string")) -> ()  [unwired: 1 out]
                n1342 = local read "Normal \nVolume (ul) 3"() -> (w2524:dbl)
                n1343 = Divide(x=w2524, y=1000.0) -> (x/y=w2519:dbl)
                n1344 = Number To Fractional String(number=w2519) -> (F-format string=w2522:string)  [unwired: 3 in]
                n1345 = String Subset(string=w2522, length (rest)=6 ("length (rest)")) -> (substring=w2520:string)  [unwired: 1 in]
                n1346 = Concatenate Strings("TGT", w2520) -> ()  [unwired: 1 out]
              }
            }
          }
          event "Normal \nRate (ul/hr)  3": Value Change {
            n1347 = event-data() -> ()  [unwired: 1 in, 5 out]
            n1348 = Number To Fractional String(number="Normal \nRate (ul/hr)  3") -> (F-format string=w2536:string)  [unwired: 3 in]
            n1349 = String Subset(string=w2536, length (rest)=6 ("length (rest)")) -> (substring=w2534:string)  [unwired: 1 in]
            n1350 = Concatenate Strings("RAT", w2534, "UH") -> (w2537:string)
            n1351 = call "Write to pump 2.vi"("String to write"=w2537, "VISA resource name"=w2538) -> ()  [unwired: 8 in, 2 out]
          }
          event "Clear Volume": Value Change {
            n1352 = event-data() -> ()  [unwired: 1 in, 5 out]
            n1353 = Divide(x="Normal \nVolume (ul) 3", y=1000.0) -> (x/y=w2556:dbl)
            n1354 = Number To Fractional String(number=w2556) -> (F-format string=w2559:string)  [unwired: 3 in]
            n1355 = String Subset(string=w2559, length (rest)=6 ("length (rest)")) -> (substring=w2557:string)  [unwired: 1 in]
            n1356 = flat-sequence {
              tunnel: [w2566] -> w2554
              tunnel: [w2565] -> w2553
              tunnel: w2543 -> [w2564]
              tunnel: w2542 -> [w2563]
              tunnel: [w2568] -> w2551
              tunnel: [w2567] -> w2552
              tunnel: w2548 -> [w2569]
              tunnel: w2554 -> [w2568]
              tunnel: w2553 -> [w2567]
              tunnel: w2552 -> [w2573]
              tunnel: w2551 -> [w2574]
              tunnel: [w2572] -> _
              tunnel: [w2571] -> _
              tunnel: w2541 -> [w2570]
              frame #0 {
                n1357 = call "Write to pump 2.vi"("String to write"=w2563, "VISA resource name"=w2564) -> ("error out"=w2565:errorcluster, "VISA resource name out"=w2566:refnum<visa-resource-name>)  [unwired: 8 in]
              }
              frame #1 {
                n1358 = Wait (ms)(milliseconds to wait=w2569) -> ()  [unwired: 1 out]
              }
              frame #2 {
                n1359 = call "Write to pump 2.vi"("error in (no error)"=w2573, "String to write"=w2570, "VISA resource name"=w2574) -> ("error out"=w2571:errorcluster, "VISA resource name out"=w2572:refnum<visa-resource-name>)  [unwired: 7 in]
              }
            }
            n1360 = local read "Write Wait"() -> (w2548:i32)
            n1361 = Concatenate Strings("TGT", w2557) -> (w2542:string)
            n1362 = local read "Normal \nRate (ul/hr)  3"() -> (w2544:dbl)
            n1363 = local write "Clear Volume"(FALSE ("Clear Volume")) -> ()
            n1364 = Number To Fractional String(number=w2544) -> (F-format string=w2547:string)  [unwired: 3 in]
            n1365 = String Subset(string=w2547, length (rest)=6 ("length (rest)")) -> (substring=w2545:string)  [unwired: 1 in]
            n1366 = Concatenate Strings("RAT", w2545, "UH" ("string")) -> (w2541:string)
          }
        }
        n1367 = node-c288() -> ()  [unwired: 1 in, 1 out]
      }
      n1368 = node-c288(w2428) -> ()  [unwired: 1 out]
    }
  }
  n1369 = node-c288() -> (w80:T11)  [unwired: 4 in]
  n1370 = timed-loop {
    timing: w80 -> [_]
    timing-out: [_] -> w79
    stop <- w2581 stop-if-true
    n1371 = node-c288() -> ()  [unwired: 1 in, 1 out]
    n1372 = event shown="[1] \"Stop\": Value Change" {
      selector: _ -> [_ _]
      dyn-events: _ -> [_ _]
      timeout: _ -> [_ _]
      tunnel: [_ "Stop"] -> w2581
      event Timeout {
        n1373 = event-data() -> ()  [unwired: 1 in, 2 out]
      }
      event "Stop": Value Change {
        n1374 = event-data() -> ()  [unwired: 1 in, 4 out]
        n1375 = local write "Force Feedback"(FALSE ("Force Feedback")) -> ()
      }
    }
    n1376 = node-c288() -> ()  [unwired: 1 in, 1 out]
  }
  n1377 = case shown="True" w69 {
    tunnel: w74 -> [_ w2588]
    tunnel: w73 -> [_ w2587]
    tunnel: w72 -> [_ w2586]
    frame False {
    }
    frame True {
      w2590 = T19 3 items=["no dialog", "OK message", "continue or stop message", "OK message + warnings", "continue/stop + warnings"] ("type of dialog (OK msg:1)")
      w2589 = T19 3 items=["no dialog", "OK message", "continue or stop message", "OK message + warnings", "continue/stop + warnings"] ("type of dialog (OK msg:1)")
      n1378 = call <vilib>:"DAQmx Clear Task.vi"("task in"=w2588, "error in"=w2586) -> ("error out"=w2591:errorcluster)  [unwired: 13 in]
      n1379 = call <vilib>:"DAQmx Clear Task.vi"("task in"=w2587) -> ("error out"=w2592:errorcluster)  [unwired: 14 in]
      n1380 = call <vilib>:"Simple Error Handler.vi"("type of dialog (OK msg:1)"=w2590, "error in (no error)"=w2591) -> ()  [unwired: 3 in, 5 out]
      n1381 = call <vilib>:"Simple Error Handler.vi"("type of dialog (OK msg:1)"=w2589, "error in (no error)"=w2592) -> ()  [unwired: 3 in, 5 out]
    }
  }
  n1382 = case shown="\"Force Feedback\", Default" "?" {
    frame "Force Feedback", Default {
    }
    frame "Raster scan" {
    }
  }
  n1383 = node-c288(w79) -> ()  [unwired: 1 out]
  n1384 = node-c288(w82) -> ()  [unwired: 1 out]
  n1385 = local write "Pause Mouse/Mirror Connection"(FALSE ("Pause Mouse/Mirror Connection")) -> ()
  n1386 = local write "Stop"(FALSE ("Stop all")) -> ()
  "CoordinatesMousePressed" <- T5 {"Horizontal"=0, "Vertical"=0} ("Coords when pressed")
  "Deflection" <- T5 {"Horizontal"=0, "Vertical"=0} ("Coords when pressed")
